vi "myRIO_BRig_RT_v0,85__PortC.vi"() -> ()   [LabVIEW 2014]
uses:
  myRIO_BRig_RT__Case_Exp_stateList.ctl
  myRIO_BRig_RT__Case_NonExp_stateList.ctl
  <vilib>/Platform/TimedLoop/XDataNode/timing_clust.ctl
  <vilib>/Platform/TimedLoop/XDataNode/nitl_modes.ctl
  <vilib>/Platform/TimedLoop/XDataNode/wakeup.ctl
  <vilib>/WebDAVClient/Advanced/SessionHandle.ctl
  <vilib>/myRIO/Common/Instrument Driver Framework/myRIO v1.0/UART/vis/myRIO v1.0 Close UART.vi
  <vilib>/FPGAPlugInAG/myRIO-1900/niLvFpga_Open_myRIO-1900.vi
  <vilib>/rvi/interface/common/dynamic/niFpgaDynamicAddResources.vi
  <vilib>/Utility/error.llb/Error Cluster From Error Code.vi
  <vilib>/rvi/errors/niLvFpgaAdjustHostInterfaceError.vi
  <vilib>/FPGAPlugInAG/Dynamic/niLvFpga_Close_Dynamic.vi
  <vilib>/myRIO/Common/Instrument Driver Framework/Utilities/vis/FPGA Ref Manager.vi
  <vilib>/myRIO/Common/Instrument Driver Framework/myRIO v1.0/myRIO v1.0 Reset FPGA.vi
  <vilib>/myRIO/Common/Instrument Driver Framework/myRIO v1.0/IRQ/vis/myRIO v1.0 IRQ Info FGV.vi
  <vilib>/myRIO/Common/Instrument Driver Framework/myRIO v1.0/IRQ/vis/myRIO v1.0 Timer IRQ Info FGV.vi
  <vilib>/myRIO/Common/Instrument Driver Framework/myRIO v1.0/IRQ/vis/myRIO v1.0 ISR Agent.vi
  <vilib>/rvi/interface/nirviOpenFPGA/nirviOpenFPGA.xnode
  myRIO_BRig_FPGA_v3,81__PortC__build.lvbitx
  myRIO_BRig_FPGA_v3,81__PortC.vi
  <vilib>/rvi/interface/nirviReadWriteControl/nirviReadWriteControl.xnode
  <vilib>/Platform/TimedLoop/XDataNode/XDataNode.xnode
  <vilib>/rvi/interface/nirviCloseFPGA/nirviCloseFPGA.xnode
  <vilib>/Platform/TimedLoop/XDataNode/XDNodeRunTimeDep.lvlib
  <vilib>/rvi/interface/Simulation/niFpgaSimulationCallBeginRW.vi
  <vilib>/myRIO/Instrument Drivers/Utilities/Utilities.lvlib
  <vilib>/WebDAVClient/NI_WebDAV.lvlib
  NiFpgaLv.dll
panel:
  in  "CueLed_baseline":bool
  out "allReward_R":bool
  out "allReward_L":bool
  in  "I_allReward":bool caption="NonSpecific Lick Direction"
  in  "Tcycle_Reward_max_R":u16=1000 caption="Max" min=5 max=5000 step=5
  in  "Tcycle_Reward_min_R":u16=1000 caption="Min" min=5 max=5000 step=5
  in  "Tcycle_Reward_step_R":u16=1000 caption="Penalty" min=1 max=10000 step=1
  in  "Tcycle_Reward_max_L":u16=1000 caption="Max" min=5 max=5000 step=5
  in  "Tcycle_Reward_min_L":u16=1000 caption="Min" min=5 max=5000 step=5
  in  "Tcycle_Reward_step_L":u16=1000 caption="Penalty" min=1 max=10000 step=1
  in  "MTrig_CueLed":bool
  out "Threshold":bool
  out "tLoop":dbl
  in  "Tcycle_Cue_LED_max":u16=1000 caption="Max" min=5 max=5000 step=5
  in  "Tcycle_Cue_LED_min":u16=1000 caption="Min" min=5 max=5000 step=5
  in  "Tcycle_CuePenalty_LED":u16=1000 caption="Penalty" min=1 max=10000 step=1
  out "power_l2":dbl
  in  "MTrig_Laser_Switch":bool
  in  "Cue1Param_AudioLed_Count_NS":u16
  in  "Cue1Param_AudioLed_Count_Switch":u16
  in  "Cue1Param_AudioLed_Probability_NS":u16
  in  "Cue1Param_CueType_NS":u16(slide) max=2 step=1 scale=0.0..2.0
  in  "Cue1Param_AudioLed_Probability_Switch":u16
  in  "Cue1Param_CueType_Switch":u16(slide) max=2 step=1 scale=0.0..2.0
  in  "CueLed_Freq":dbl=10.0
  in  "CueLed_Tpeak":dbl=2.0
  in  "Laser_power_step_l2":dbl
  in  "Laser_power_max_l2":dbl
  in  "Laser_power_min_l2":dbl
  in  "Laser_Tshutter_l2":dbl=2.0
  in  "Laser_Freq_l2":dbl=10.0
  in  "Laser_Tpeak_l2":dbl=2.0
  in  "Laser_duration_l2":u16
  in  "LC_Sel_Count_NS_l2":u16
  in  "LC_Sel_Count_Switch_l2":u16
  in  "LC_Sel_Probability_NS_l2":u16
  in  "LC_Sel_Block_NS_l2":u16(slide) max=2 step=1 scale=0.0..2.0
  in  "LC_Sel_OnOff_NS_l2":bool
  in  "LC_Sel_Probability_Switch_l2":u16
  in  "LC_Sel_Block_Switch_l2":u16(slide) max=2 step=1 scale=0.0..2.0
  in  "LC_Sel_OnOff_Switch_l2":bool
  in  "LC_Sel_Tdelay_NS_l2":u16
  in  "LC_Sel_Tdelay_Switch_l2":u16
  in  "LC_Cue1_Count_NS_l2":u16
  in  "LC_Cue1_Count_Switch_l2":u16
  in  "LC_Cue1_delayOpt_NS_l2":bool
  in  "LC_ENL1_delayOpt_NS_l2":bool
  in  "LC_ENL1_Count_NS_l2":u16
  in  "LC_ENL1_Count_Switch_l2":u16
  in  "LC_Cue1_delayOpt_Switch_l2":bool
  in  "LC_ENL1_delayOpt_Switch_l2":bool
  in  "LC_Cue1_Probability_NS_l2":u16
  in  "LC_Cue1_Block_NS_l2":u16(slide) max=2 step=1 scale=0.0..2.0
  in  "LC_Cue1_OnOff_NS_l2":bool
  in  "LC_Cue1_Probability_Switch_l2":u16
  in  "LC_Cue1_Block_Switch_l2":u16(slide) max=2 step=1 scale=0.0..2.0
  in  "LC_Cue1_OnOff_Switch_l2":bool
  in  "LC_ENL1_Probability_NS_l2":u16 max=100 step=1
  in  "LC_ENL1_Block_NS_l2":u16(slide) max=2 step=1 scale=0.0..2.0
  in  "LC_ENL1_OnOff_NS_l2":bool
  in  "LC_ENL1_Probability_Switch_l2":u16 max=100 step=1
  in  "LC_ENL1_Block_Switch_l2":u16(slide) max=2 step=1 scale=0.0..2.0
  in  "LC_Cue1_Tdelay_NS_l2":u16
  in  "LC_ENL1_Tdelay_NS_l2":u16
  in  "LC_Cue1_Tdelay_Switch_l2":u16
  in  "LC_ENL1_Tdelay_Switch_l2":u16
  in  "LC_ENL1_OnOff_Switch_l2":bool
  in  "LC_Wrong_Probability_l2":u16
  in  "LC_Wrong_Trial_l2":u16(slide) max=2 step=1 scale=0.0..2.0
  in  "LC_Wrong_Block_l2":u16(slide) max=2 step=1 scale=0.0..2.0
  in  "LC_Wrong_OnOff_l2":bool
  in  "LC_Reward_Probability_l2":u16
  in  "LC_Reward_Trial_l2":u16(slide) max=2 step=1 scale=0.0..2.0
  in  "LC_Reward_Block_l2":u16(slide) max=2 step=1 scale=0.0..2.0
  in  "LC_Reward_OnOff_l2":bool
  in  "LC_Wrong_Tdelay_l2":u16
  in  "LC_Reward_Tdelay_l2":u16
  in  "LC_Sel_Count_NS_l1":u16
  in  "LC_Sel_Count_Switch_l1":u16
  in  "LC_Sel_Probability_NS_l1":u16
  in  "LC_Sel_Block_NS_l1":u16(slide) max=2 step=1 scale=0.0..2.0
  in  "LC_Sel_OnOff_NS_l1":bool
  in  "LC_Sel_Probability_Switch_l1":u16
  in  "LC_Sel_Block_Switch_l1":u16(slide) max=2 step=1 scale=0.0..2.0
  in  "LC_Sel_OnOff_Switch_l1":bool
  in  "LC_Sel_Tdelay_NS_l1":u16
  in  "LC_Sel_Tdelay_Switch_l1":u16
  out "I_connect_TCP":bool
  in  "get_countPerMS":bool
  in  "count_warmup_R_reset":bool
  in  "count_warmup_L_reset":bool
  out "count_warmup_R":u16
  out "count_warmup_L":u16
  out "SolenoidReward":bool
  in  "SolenoidProbability_L":u16=100 caption="Reward Time [ms]" min=1 max=1000 step=1
  in  "SolenoidProbability_R":u16=100 caption="Reward Time [ms]" min=1 max=1000 step=1
  out "power_l1":dbl caption="LaserPower"
  in  "Laser_power_step_l1":dbl
  in  "Laser_power_max_l1":dbl
  in  "Recording":bool
  in  "Laser_power_min_l1":dbl
  in  "FPGA_count2ms":dbl=159.0
  in  "Laser_Tshutter_l1":dbl=2.0
  in  "Laser_Freq_l1":dbl=10.0
  in  "Laser_Tpeak_l1":dbl=2.0
  in  "Laser_duration_l1":u16
  out "error out":errorcluster
  in  "LC_Cue1_Count_NS_l1":u16
  in  "LC_Cue1_Count_Switch_l1":u16
  in  "LC_Cue1_delayOpt_NS_l1":bool
  in  "LC_ENL1_delayOpt_NS_l1":bool
  in  "LC_ENL1_Count_NS_l1":u16
  in  "LC_ENL1_Count_Switch_l1":u16
  in  "LC_Cue1_delayOpt_Switch_l1":bool
  in  "LC_ENL1_delayOpt_Switch_l1":bool
  in  "Tcycle_Cue_Audio_max":u16=1000 caption="Max" min=5 max=5000 step=5
  in  "Tcycle_Cue_Audio_min":u16=1000 caption="Min" min=5 max=5000 step=5
  in  "SendData":bool
  out "cSpout":enum16{"Left", "Right"}(ring) caption="Left or Right Spout"
  out "A4":u32 caption="LickCounter_Right"
  out "A2":u32 caption="LickCounter_Left"
  in  "LR_wrong_Event":bool
  out "SelectWrong":bool
  out "SelectReward":bool
  in  "Left(F)_or_Right(T)":bool
  in  "ignoreWrong":bool
  in  "SelectionState":bool
  in  "LR_wrong_Laser":bool
  in  "LR_reward_Laser":bool
  in  "LR_reward_Event":bool
  out "nRewards_Right":u16 caption="# Rewards Total (Right)"
  out "nRewards_Left":u16 caption="# Rewards Total (Left)"
  out "nRewards_cur":u16 caption="# Rewards in Current Block"
  out "TpB_target":u16 caption="Target Trials Per Block"
  out "cState_NonExp":T1 caption="WarmUp State"
  out "iBlock":u16 caption="Current Block"
  out "cState":T2 caption="Experimental State"
  out "iTrial":u16 caption="Current Trial"
  in  "warmupType":u8(slide) max=2 step=1 scale=0.0..2.0
  in  "TestConnection":bool
  in  "warmup":bool caption="WarmUp"
  in  "Data Set Prefix":string="Exp1_TM2"
  out "Connected To Host?":bool
  in  "Host Password":string="sabalab"
  in  "Host UserName":string="Test2"
  in  "sp_RightSpout":u16(slide)=2 max=2 step=1 scale=0.0..2.0
  in  "sp_LeftSpout":u16(slide)=2 max=2 step=1 scale=0.0..2.0
  in  "BUR_max":u16 caption="Count Reward Structure  (0 = off)"
  in  "LC_Wrong_Probability_l1":u16
  in  "LC_Wrong_Trial_l1":u16(slide) max=2 step=1 scale=0.0..2.0
  in  "LC_Wrong_Block_l1":u16(slide) max=2 step=1 scale=0.0..2.0
  in  "LC_Wrong_OnOff_l1":bool
  in  "LC_Reward_Probability_l1":u16
  in  "LC_Reward_Trial_l1":u16(slide) max=2 step=1 scale=0.0..2.0
  in  "LC_Reward_Block_l1":u16(slide) max=2 step=1 scale=0.0..2.0
  in  "LC_Reward_OnOff_l1":bool
  in  "LC_Cue1_Probability_NS_l1":u16
  in  "LC_Cue1_Block_NS_l1":u16(slide) max=2 step=1 scale=0.0..2.0
  in  "LC_Cue1_OnOff_NS_l1":bool
  in  "LC_Cue1_Probability_Switch_l1":u16
  in  "LC_Cue1_Block_Switch_l1":u16(slide) max=2 step=1 scale=0.0..2.0
  in  "LC_Cue1_OnOff_Switch_l1":bool
  in  "LC_ENL1_Probability_NS_l1":u16 max=100 step=1
  in  "LC_ENL1_Block_NS_l1":u16(slide) max=2 step=1 scale=0.0..2.0
  in  "LC_ENL1_OnOff_NS_l1":bool
  in  "LC_ENL1_Probability_Switch_l1":u16 max=100 step=1
  in  "LC_ENL1_Block_Switch_l1":u16(slide) max=2 step=1 scale=0.0..2.0
  in  "Tcycle_Timeout":u16=1000 caption="Timeout Time [ms]" min=10 max=10000 step=1
  in  "Tcycle_Wrong":u16=1000 caption="Wrong Time [ms]" min=10 max=10000 step=1
  in  "Tcycle_Selection":u16=1000 caption="Answer Time [ms]" min=1 max=10000 step=1
  in  "Tcycle_RewardPost":u16=1000 caption="Consumption Time [ms]" min=250 max=10000 step=250
  in  "TpB_Max_R":u16=4 caption="Max TrialsPerBlock" min=1 max=12 step=1
  in  "TpB_Min_R":u16=4 caption="Min TrialsPerBlock" min=1 max=12 step=1
  in  "TpB_Max_L":u16=4 caption="Max TrialsPerBlock" min=1 max=12 step=1
  in  "TpB_Min_L":u16=4 caption="Min TrialsPerBlock" min=1 max=12 step=1
  in  "BUR_min":u16 caption="Count Reward Structure\n(0 = off)"
  in  "TrialUntilReward":bool caption="Ignore Wrong Selection"
  in  "CueCycles":u16=1 caption="Cue Structure" min=1 max=1 step=1
  in  "MTrig_Laser_Tcycle":u16=10 caption="Time [ms]"
  in  "MTrig_Laser_trig":bool
  in  "MTrig_Audio_trig__R":bool caption="Trigger Audio"
  in  "MTrig_Audio_trig__L":bool caption="Trigger Audio"
  in  "RewCalib_Trig_R":bool caption="Calibrate_R"
  in  "RewCalib_Trig_L":bool caption="Calibrate_L"
  in  "MTrig_Solenoid_Tcycle__R":u16=300 caption="Time [ms]"
  in  "MTrig_Solenoid_Tcycle__L":u16=300 caption="Time [ms]"
  in  "MTrig_Solenoid_trig__R":bool caption="Solenoid"
  in  "MTrig_Solenoid_trig__L":bool caption="Solenoid"
  in  "STOP_abort":bool caption="Stop LabView\n(Stops myRio and FPGA)"
  in  "STOP_endBlock":bool caption="Stop Experiment\n@ End of Block"
  in  "STOP_endTrial":bool caption="Stop Experiment\n@ End of Trial"
  in  "START":bool caption="Start Experiment"
  in  "Tcycle_CuePenalty_Audio":u16=1000 caption="Penalty" min=1 max=10000 step=1
  in  "Audio_Amp__R":u16=100 caption="Amp"
  in  "Audio_Freq__R":u8=5 caption="Freq [kHz]" max=14 step=1
  in  "Audio_Amp__L":u16=100 caption="Amp"
  in  "Audio_Freq__L":u8=5 caption="Freq [kHz]" max=14 step=1
  in  "LC_Wrong_Tdelay_l1":u16
  in  "LC_Cue1_Tdelay_NS_l1":u16
  in  "LC_ENL1_Tdelay_NS_l1":u16
  in  "LC_Reward_Tdelay_l1":u16
  in  "LC_Cue1_Tdelay_Switch_l1":u16
  in  "LC_ENL1_Tdelay_Switch_l1":u16
  in  "LC_ENL1_OnOff_Switch_l1":bool
  in  "Tcycle_ENLPenalty":u16=100 caption="Penalty" min=10 max=10000 step=10
  in  "Tcycle_ENL_max":u16=1000 caption="Max" min=250 max=10000 step=250
  in  "Tcycle_ENL_min":u16=1000 caption="Min" min=250 max=10000 step=250
  # "Communication (Host PC)"
  # "Recording Rig"
  # "Experimental Run"
  # "Experiment Task Structure"
  # "STOP experiment at"
  # "Min            Max            Penalty"
  # "(1) = Switching\n(2) = Two Choice"
  # "Enforced\nNonLick"
  # "FPGA Count per [ms]"
  # "Cue Audio"
  # "Current State"
  # "Cue LED"
  # "Global Parameters                                                         Trial Parameters"
  # "Selection"
  # "WarmUp"
  # "Reward - Dispense Water"
  # "Left/Right        Give Reward?        Laser Power [V]"
  # "Laser1      Laser2"
  # "Left"
  # "Cue then reward (no lick)\n \nLeft                    Right"
  # "Right"
  # "Min"
  # "Max"
  # "Dispense Water Probability"
  # "Block                   Trial            Target Trials       # Rewards \n                                                            Per Block             Current"
  # "Left"
  # "WarmUp State"
  # "Trial Per Block Structure \n               Left                        Right"
  # "Lick Counter"
  # "Right"
  # "Left           Right"
  # "Reward - Consumption"
  # "Manual Control"
  # "Min"
  # "# Rewards Total\n                                                                  Left                    Right"
  # "Experimental State"
  # "Penalty - Wrong Choice"
  # "Solenoid\n \nLeft              Right"
  # "Speaker\n \nLeft                    Right"
  # "Laser 1  |  Laser 2"
  # "Max"
  # "Penalty - Choice Timeout"
  # "Time\n[ms]"
  # "Time\n[ms]"
  # "Time = Cue Min"
  # "Cue LED"
  # "Power = Min"
  # "Cue1 Control\n                                  Cue Type           LED Probability [%]      Count"
  # "Laser1 Control\n                               On/Off      Block        Probability [%]   Delay [ms]                              Count"
  # "Laser2 Control\n                               On/Off      Block        Probability [%]   Delay [ms]                              Count"
  # "Audio or LED"
  # "Cue 1"
  # "Enforced\nNonLick\n      1"
  # "Enforced\nNonLick\n      1"
  # "from end"
  # "from end"
  # "Switch\nTrial"
  # "Switch\nTrial"
  # "Switch\nTrial"
  # "from start"
  # "from start"
  # "from end"
  # "from end"
  # "NonSwitch\nTrials"
  # "NonSwitch\nTrials"
  # "NonSwitch\nTrials"
  # "from start"
  # "from start"
  # "Cue 1"
  # "Cue 1"
  # "from end"
  # "from end"
  # "Switch\nTrial"
  # "Switch\nTrial"
  # "Cue Audio Parameters"
  # "Cue LED Parameters"
  # "from start"
  # "from start"
  # "Left                  Right"
  # "Frequency\n[Hz]"
  # "Frequency\n[kHz]"
  # "from end"
  # "from end"
  # "NonSwitch\nTrials"
  # "NonSwitch\nTrials"
  # "Timing [ms]\n                    Peak Width"
  # "from start"
  # "from start"
  # "Amp\n(0 - 32,000)"
  # "Selection"
  # "Selection"
  # "from start"
  # "from start"
  # "Switch\nTrial"
  # "Switch\nTrial"
  # "Speaker\nPattern\nDuring Cue"
  # "from start"
  # "from start"
  # "NonSwitch\nTrials"
  # "NonSwitch\nTrials"
  # "Laser1 Parameters"
  # "Laser2 Parameters"
  # "Laser1 Response\n                               On/Off      Block       Trial       Probability [%]   Delay [ms]"
  # "Laser2 Response\n                               On/Off      Block       Trial       Probability [%]   Delay [ms]"
  # "Frequency\n[Hz]"
  # "Frequency\n[Hz]"
  # "Timing [ms]\n Duration     Peak Width   Shutter"
  # "Timing [ms]\n Duration     Peak Width   Shutter"
  # "Selection Reward"
  # "Selection Reward"
  # "Laser Power [V]\nMin          Max              Step"
  # "Laser Power [V]\nMin          Max              Step"
  # "Selection Wrong"
  # "Selection Wrong"
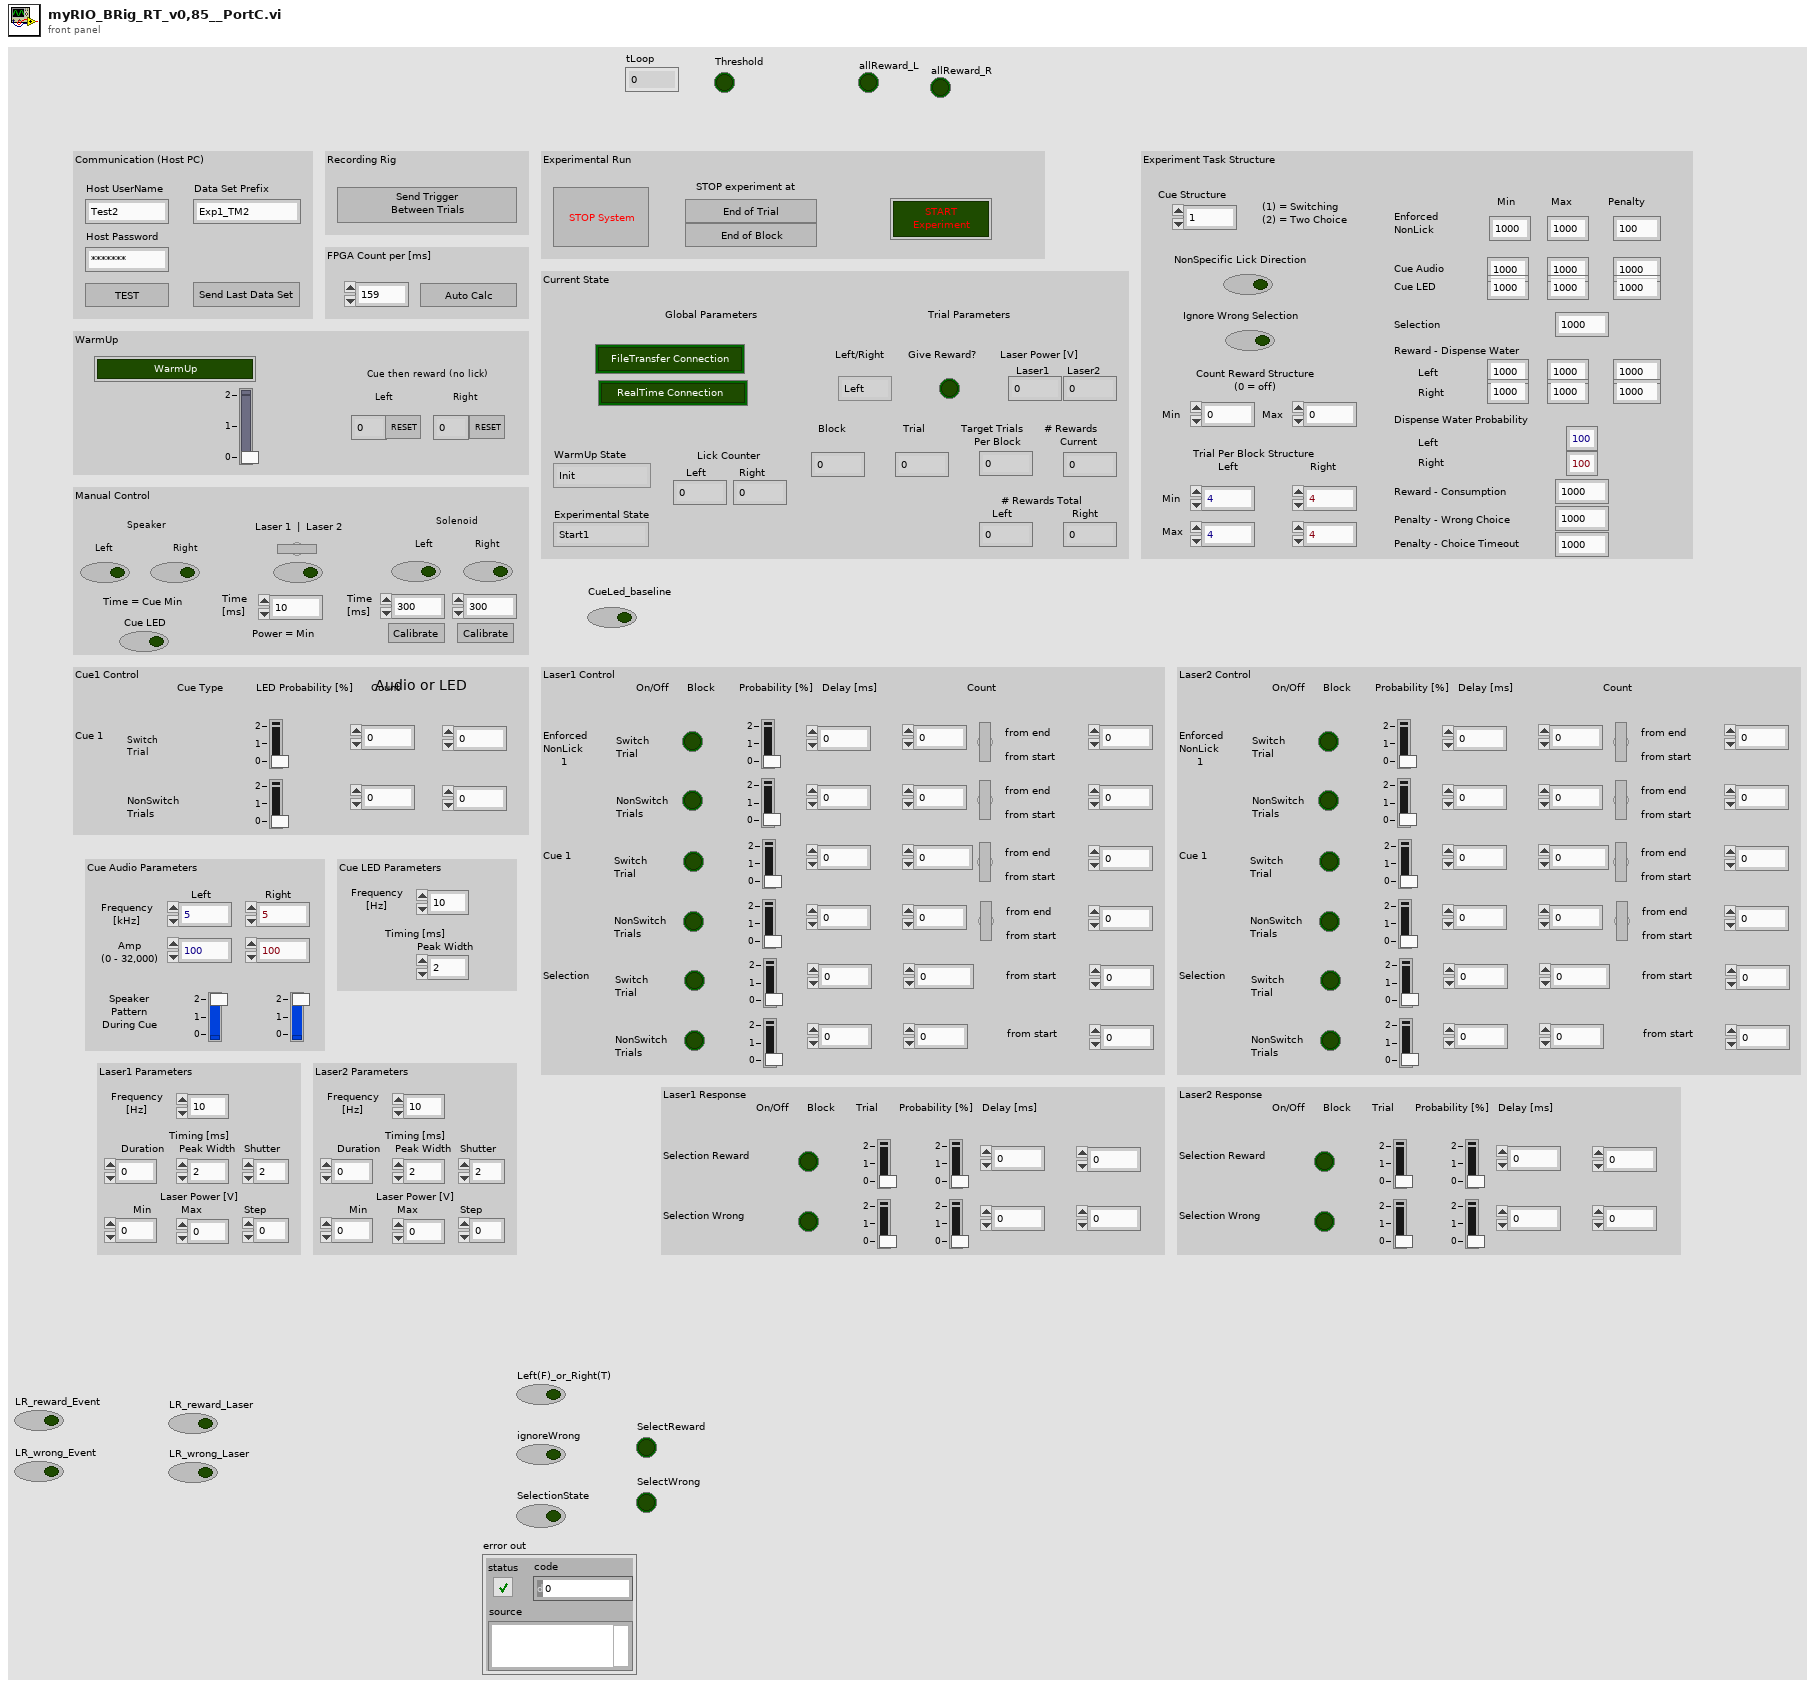
[diagram p1: front panel]
types:
  T1 = typedef "myRIO_BRig_RT__Case_NonExp_stateList.ctl" = enum16{"Init", "UploadSettings_pre", "UploadSettings_Read_dataExp", "UploadSettings_dataExp_1", "UploadSettings_dataExp_2", "UploadSettings_Read_dataLC", "UploadSettings_dataLC_1", "UploadSettings_dataLC_2", "UploadSettings_dataLC_3", "UploadSettings_dataLC_4", "UploadSettings_Read_dataMTrig", "UploadSettings_dataMTrig_1", "UploadSettings_post", "Idle_pre", "IdleEmpty", "IdleEmpty2", "IdleEmpty3", "IdleEmpty4", "Idle", "Idle_2", "Idle_3", "Idle_4", "Idle_5", "Idle_6", "Idle_post", "Cue_pre__pre", "Cue_pre", "Cue", "Cue_LED", "Cue_post", "RewardCalibration_pre", "DispenseWater_pre__pre", "DispenseWater_pre", "DispenseWater", "DispenseWater_post", "TestConnection", "SendData", "Get_FPGA_count_per_ms", "End"}
  T2 = typedef "myRIO_BRig_RT__Case_Exp_stateList.ctl" = enum16{"Start1", "Start2", "Start3", "saveSettings1", "saveSettings2", "saveSettings3", "saveSettings4", "saveSettings_LC_ENL_l1", "saveSettings_LC_ENL_l2", "saveSettings_LC_Cue_l1", "saveSettings_LC_Cue_l2", "saveSettings6_LC_l1_Other", "SaveSettings6_LC_l2_Other", "setSettings_Audio", "setSettings_Laser", "initBlock_pre", "initBlock", "initBlock2", "initBlock_post", "initTrial_pre", "initTrial", "initTrial2", "initTrial3", "initTrial4", "initTrial_LC_ENL1", "initTrial_LC_Cue1", "initTrial_LC_Cue1_2", "initTrial_LC_Sel", "initTrial_post", "ENL1_pre", "ENL1", "ENL1_post", "ENL1Penalty_pre", "ENL1Penalty", "ENL2_pre", "ENL2", "ENL2Penalty_pre", "ENL2Penalty", "Cue1_pre", "Cue1", "Cue1_post", "Cue1Penalty_pre", "Cue1Penalty", "Cue2_pre", "Cue2", "Cue2Penalty_pre", "Cue2Penalty", "Selection_pre", "Selection", "Select_post", "SelectReward_pre", "SelectReward", "SelectRewardPost_pre", "SelectRewardPost", "SelectWrong_pre", "SelectWrong", "SelectWrong_post", "SelectTimeout_pre", "SelectTimeout", "SelectTimeout_post", "endTrial_pre", "endTrial1", "endTrial2", "endTrial3", "endTrial_post", "endBlock_pre", "endBlock", "endBlock_post", "endExp", "commConnect", "commUpload_pre", "commUpload_dataBlock", "commUpload_dataCurrent", "commUpload_dataExp", "commUpload_dataLC", "commUpload_dataTrial", "commUpload_post", "saveData_pre", "saveData_dataBlock", "saveData_dataCurrent", "saveData_dataExp", "saveData_dataLC", "saveData_dataTrial", "saveData_post", "empty_endBlock1", "empty_endBlock2", "empty_endTrial1", "empty_endTrial2", "empty_endTrial3", "empty_endTrial4", "empty_endTrial5", "dummyState", "dummyState_endBlock"}
  T3 = typedef "XDNodeRunTimeDep.lvlib/timing_clust.ctl" = cluster{"Expected End [f-1]":u64, "Actual End [f-1]":u64, "Finished Late? [f-1]":bool, "Expected End [i-1]":u64, "Actual End [i-1]":u64, "Finished Late? [i-1]":bool, "Expected Start [i]":u64, "Actual Start [i]":u64, "Expected Start [f]":u64, "Actual Start [f]":u64, "Source Name":string, "Structure Name":string, "Period":i64, "Deadline":i64, "Offset":i64, "Start":i64, "Priority":i32, "Timeout":i32, "Mode":T4, "Wakeup Reason":T5, "Error":errorcluster, "Source Type":string, "Secondary Source Type":string, "Global End Time":u64, "Global Start Time":u64, "Frame Duration":u64, "Iteration Duration":u64, "Assigned CPU":i32, "I/O Scan Engine Mode":u32}
  T4 = typedef "XDNodeRunTimeDep.lvlib/nitl_modes.ctl" = enum32{"No Change", "Process missed periods, maintain original phase", "Discard missed periods, maintain original phase", "Process missed periods, ignore original phase", "Discard missed periods, ignore original phase"}
  T5 = typedef "XDNodeRunTimeDep.lvlib/wakeup.ctl" = enum32{"Normal", "Aborted", "Asynchronous wakeup", "Timing source error", "Timed loop error", "Timeout"}
  T6 = typedef "NI_WebDAV.lvlib/SessionHandle.ctl" = refnum<k1>
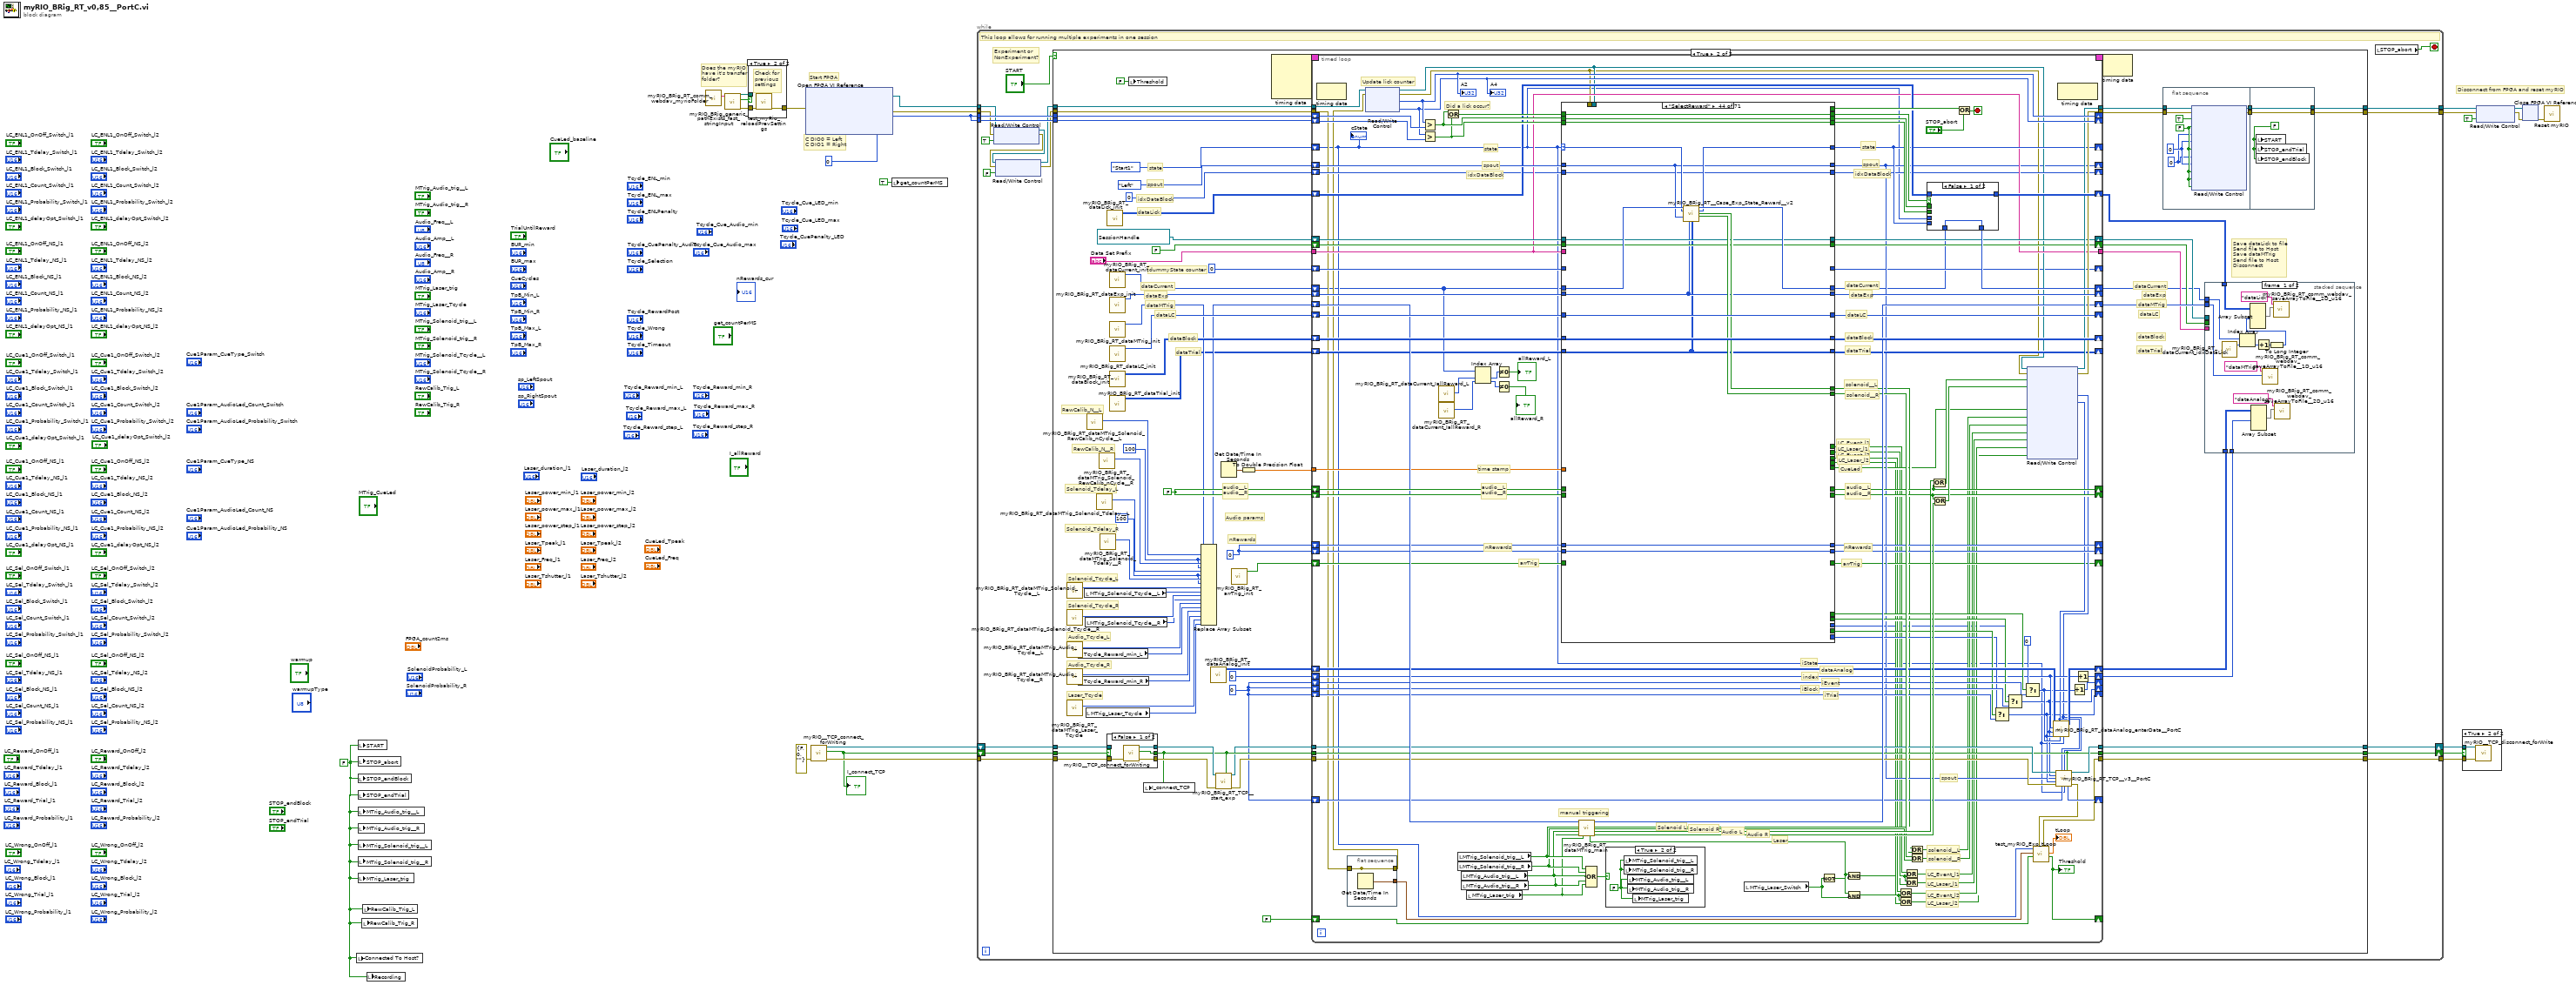
[diagram p0: block diagram]
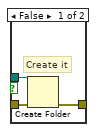
[diagram p3: hidden frame]
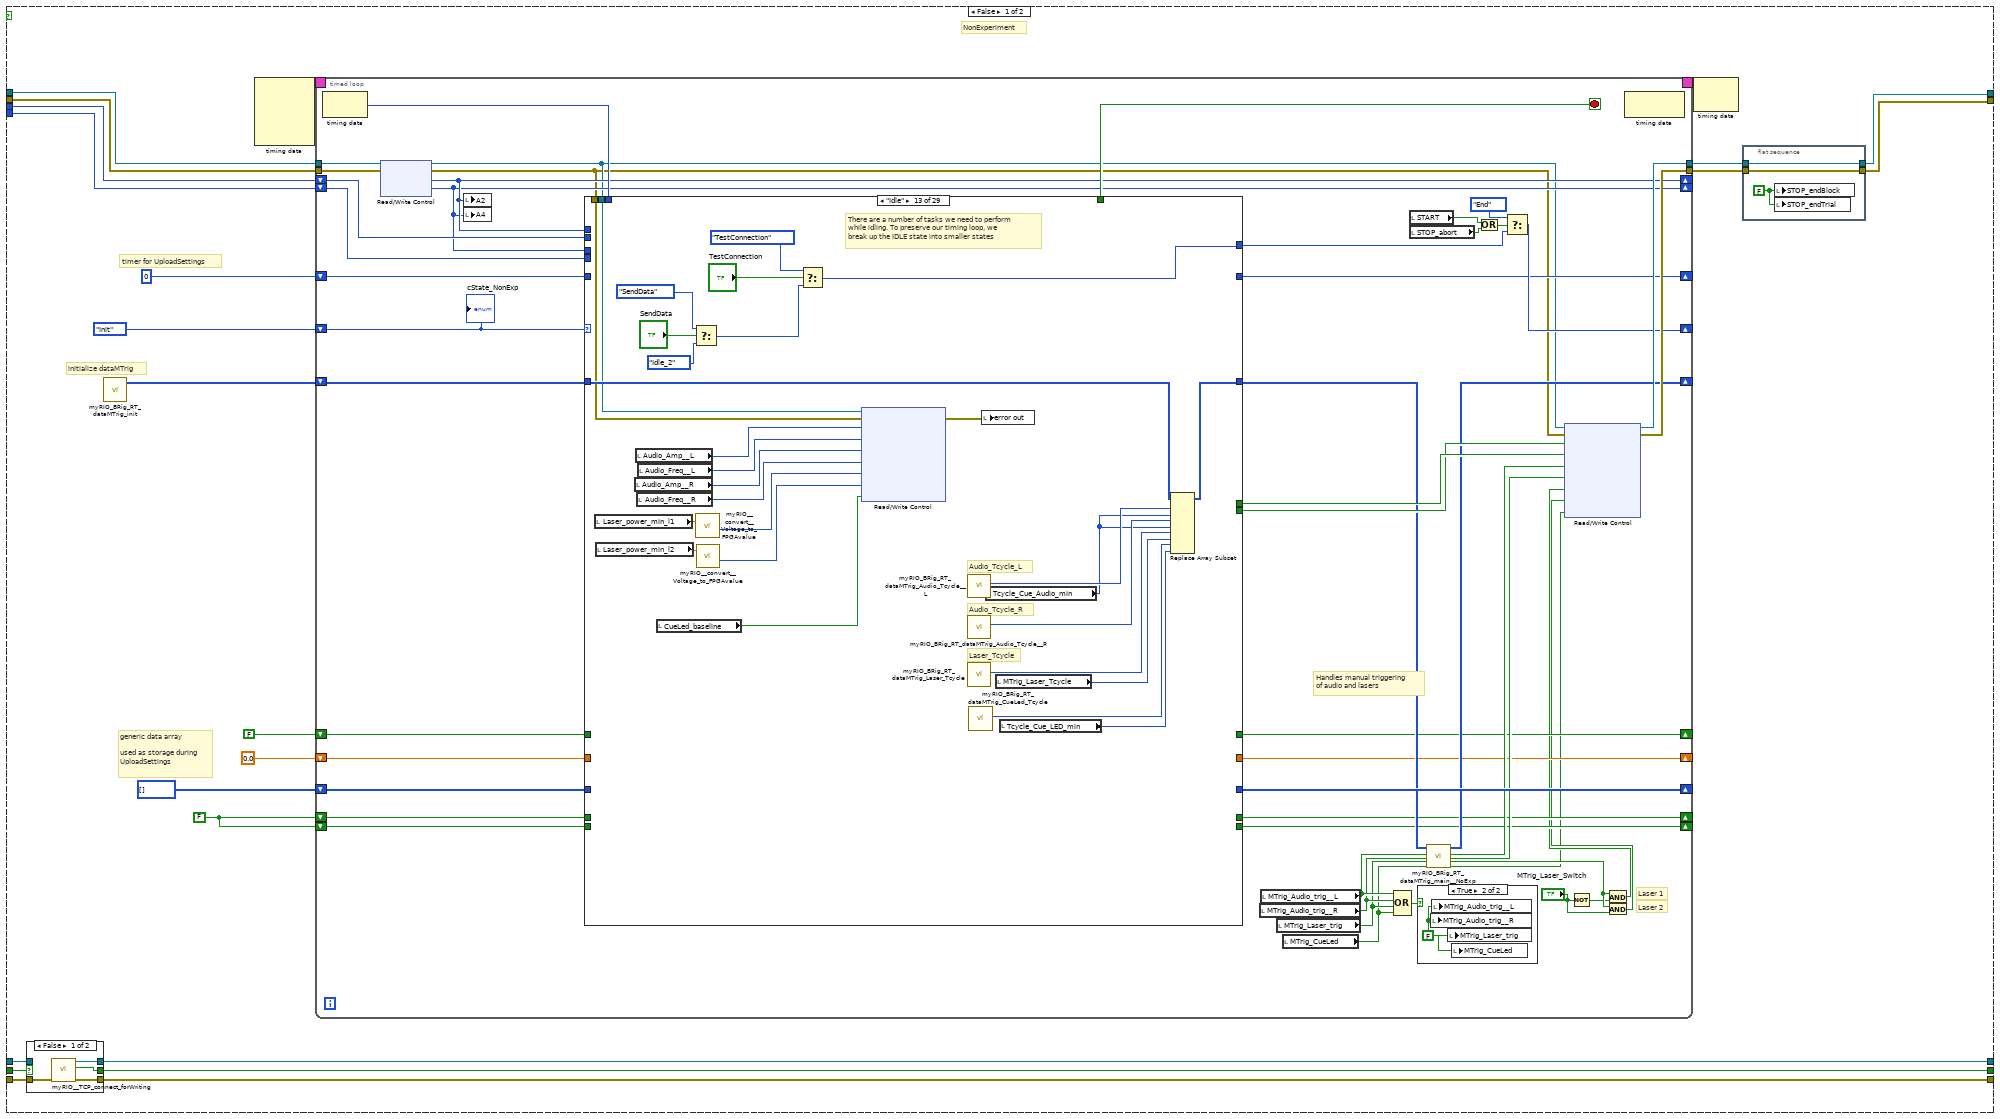
[diagram p4: hidden frame]
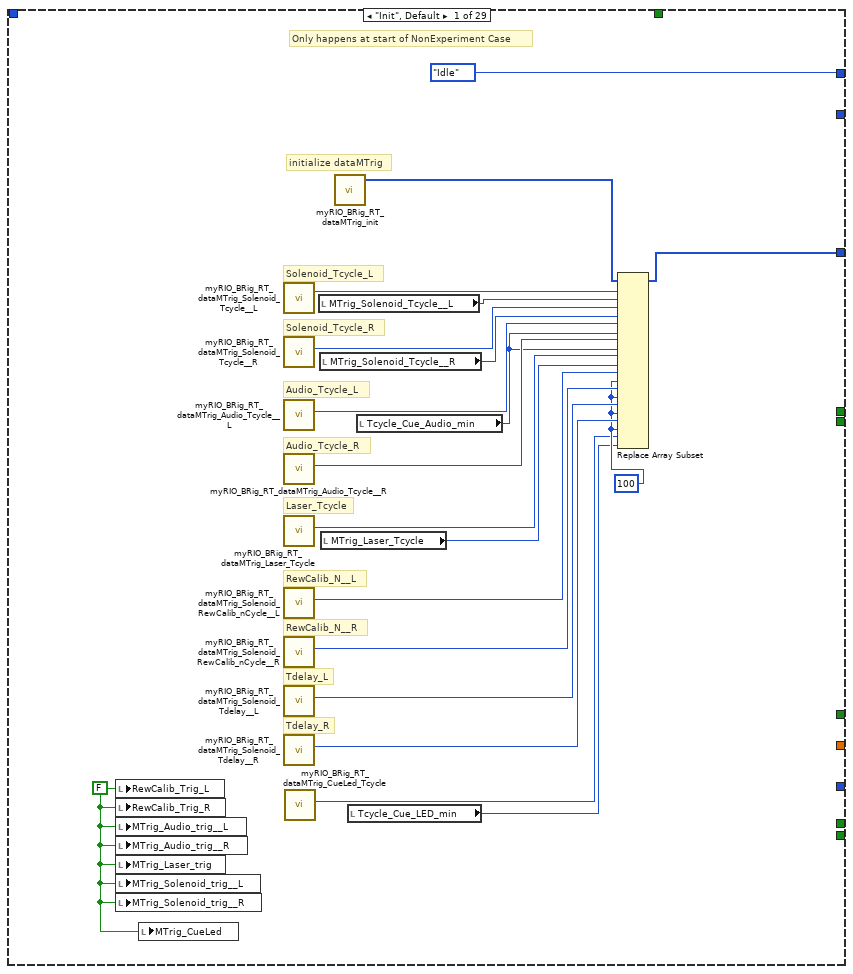
[diagram p7: hidden frame]
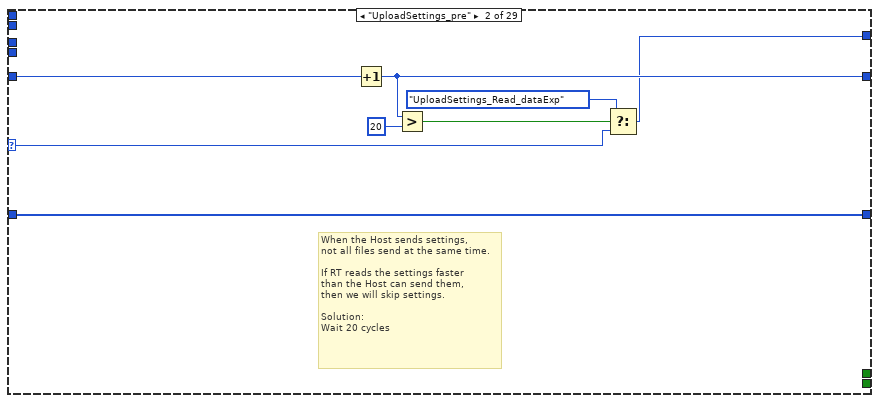
[diagram p8: hidden frame]
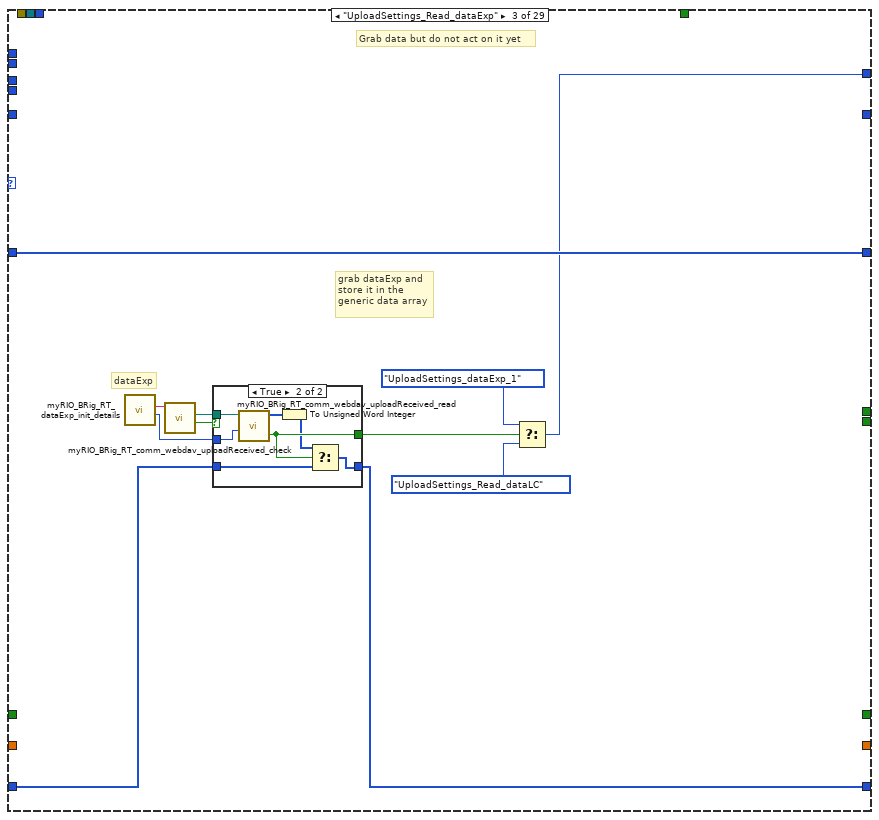
[diagram p9: hidden frame]
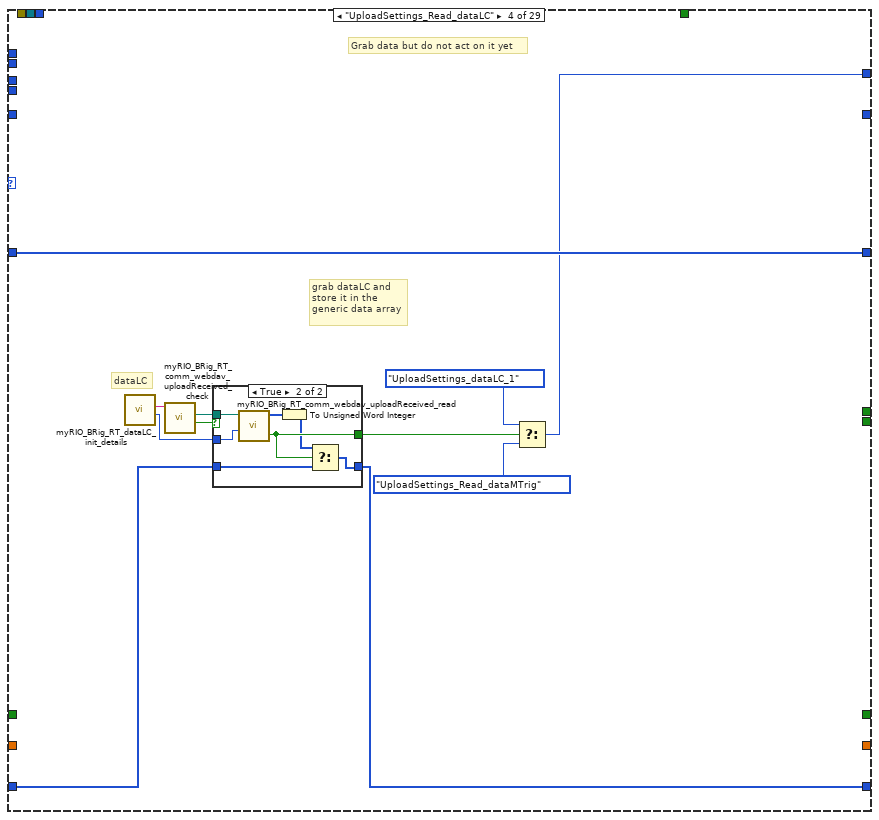
[diagram p11: hidden frame]
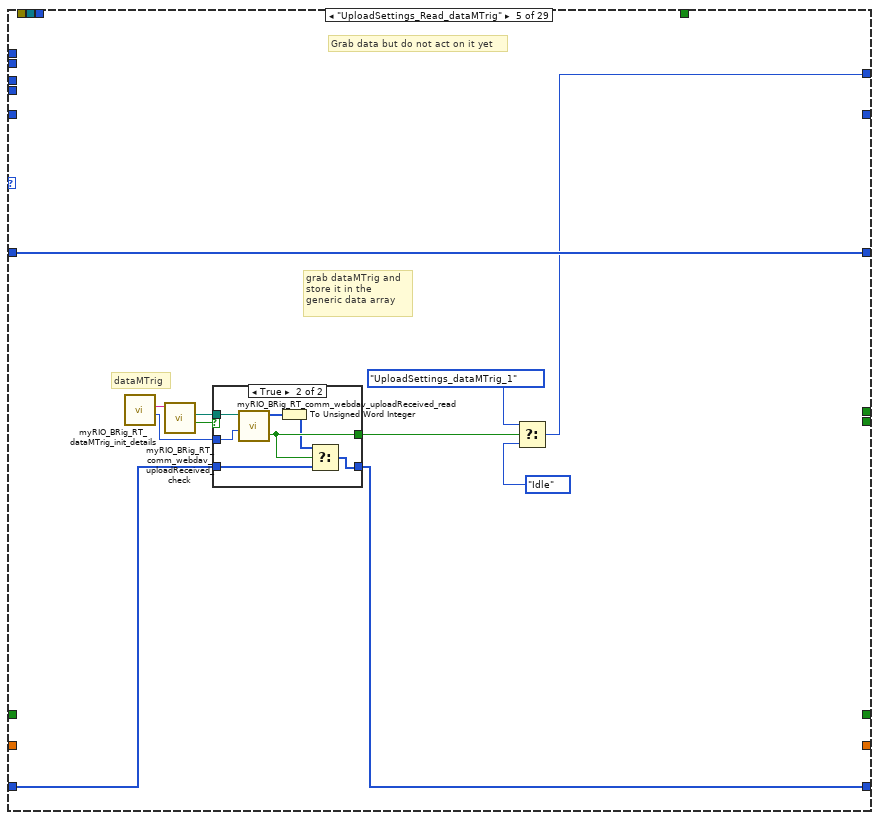
[diagram p13: hidden frame]
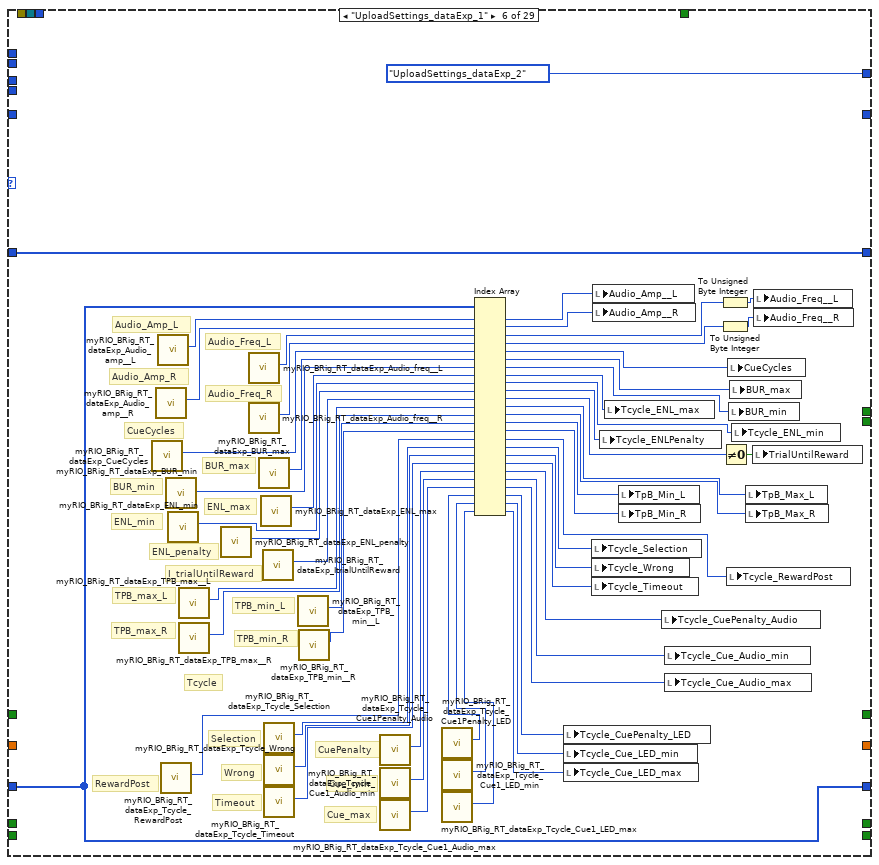
[diagram p15: hidden frame]
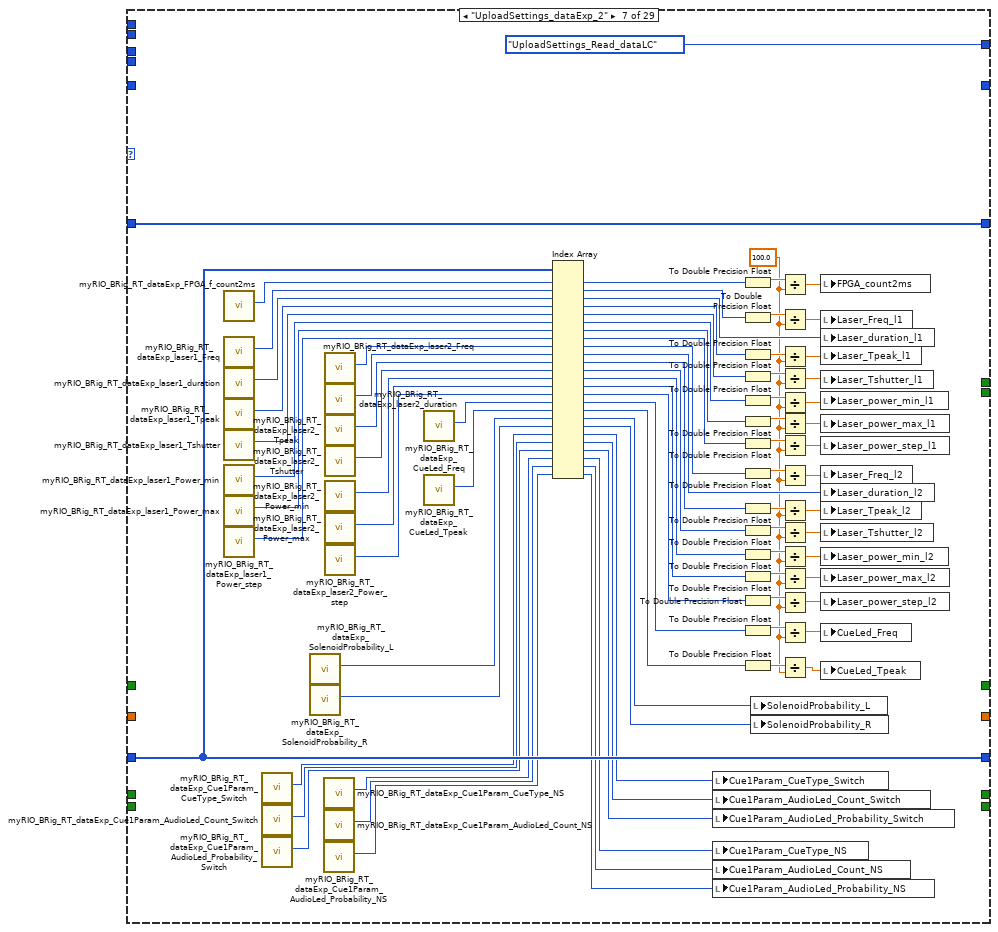
[diagram p16: hidden frame]
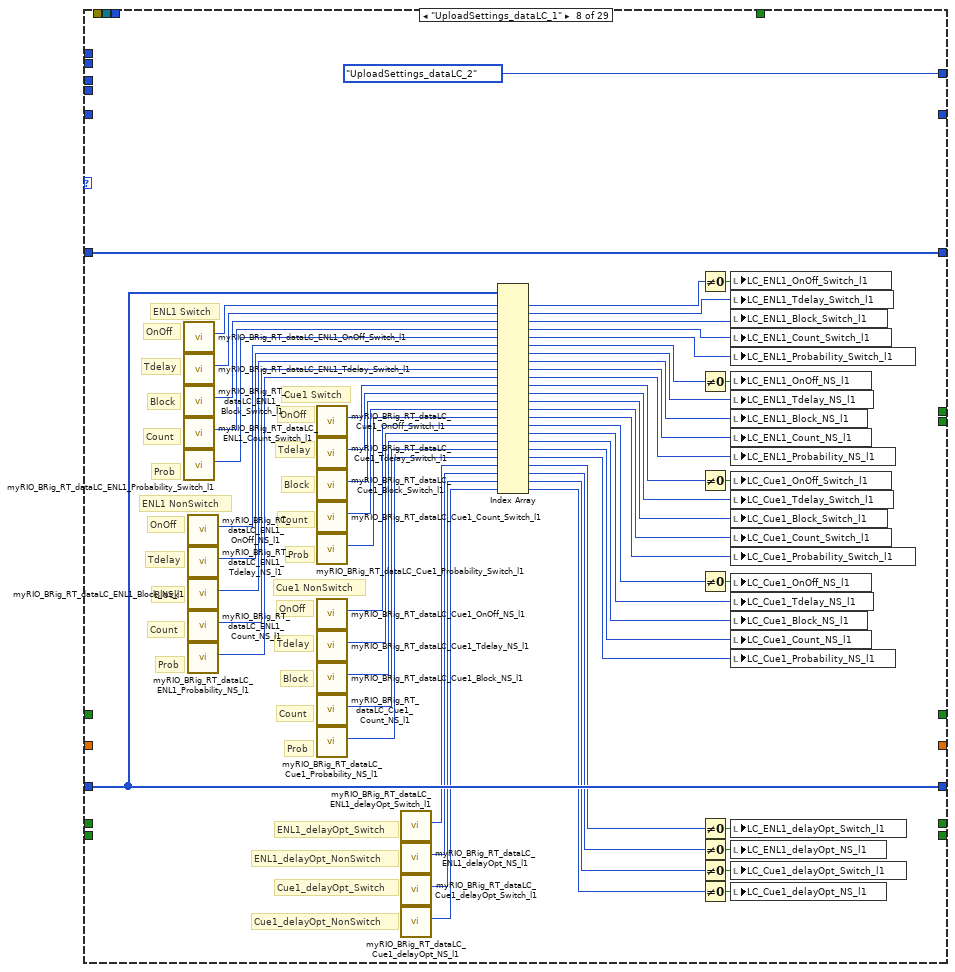
[diagram p17: hidden frame]
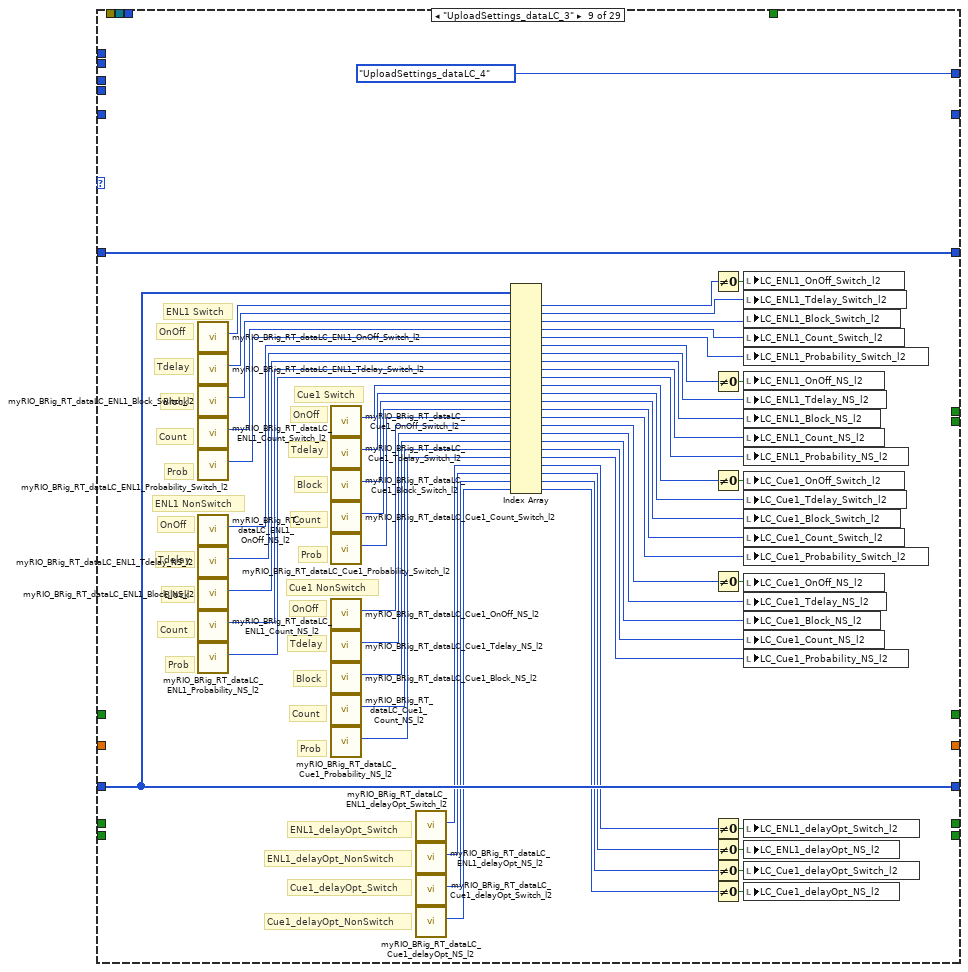
[diagram p18: hidden frame]
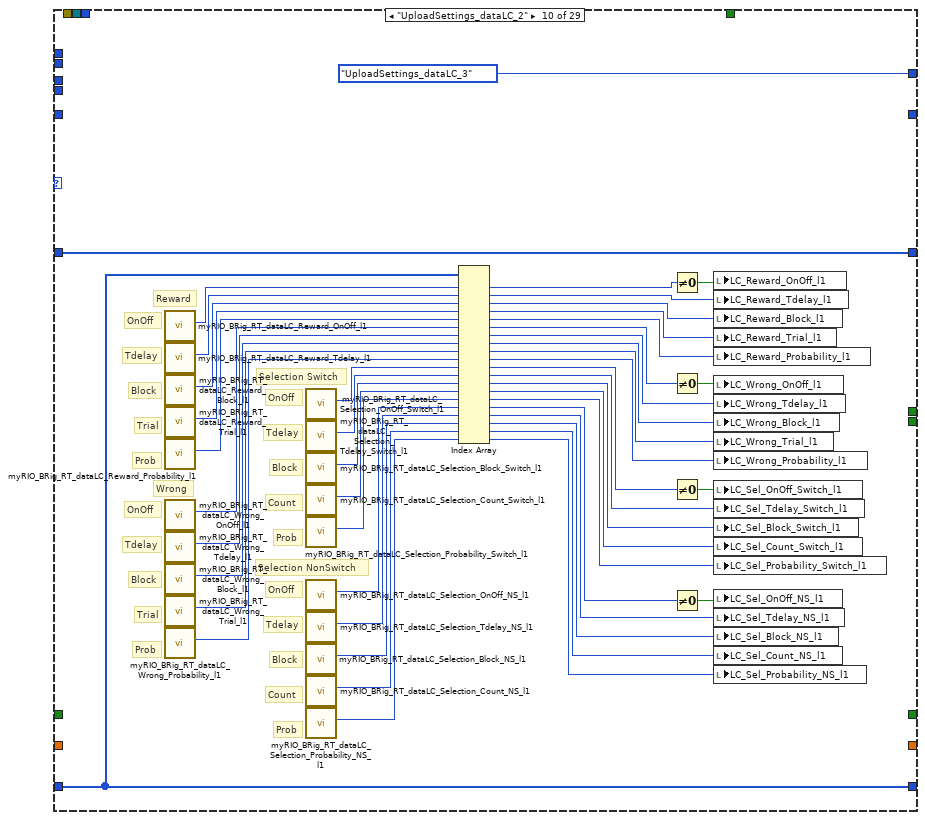
[diagram p19: hidden frame]
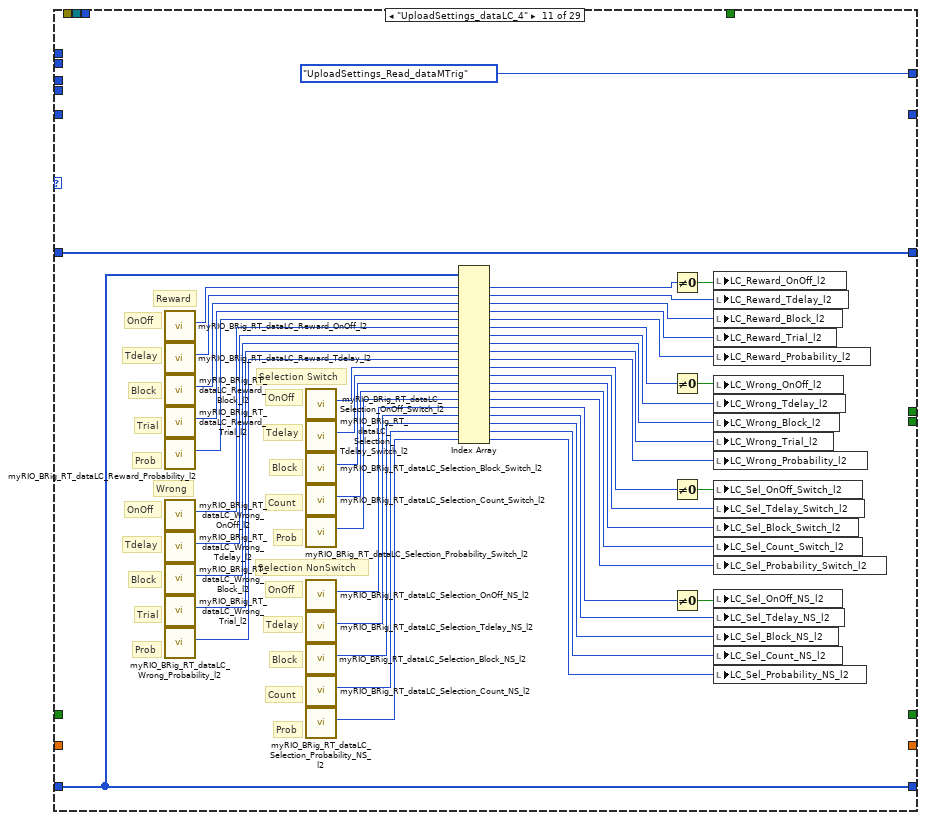
[diagram p20: hidden frame]
diagram:
  w17 = u32 0
  w1 = FALSE
  # "Does the myRIO\nhave it's transfer\nfolder?"
  # "C DIO0 = Left\nC DIO1 = Right"
  # "Start FPGA"
  # "Disconnect from FPGA and reset myRIO"
  n1 = local write "Connected To Host?"(w1) -> ()
  n2 = local write "START"(w1) -> ()
  n3 = local write "STOP_abort"(w1) -> ()
  n4 = local write "STOP_endBlock"(w1) -> ()
  n5 = local write "STOP_endTrial"(w1) -> ()
  n6 = local write "MTrig_Audio_trig__L"(w1) -> ()
  n7 = local write "MTrig_Audio_trig__R"(w1) -> ()
  n8 = local write "MTrig_Solenoid_trig__L"(w1) -> ()
  n9 = local write "MTrig_Solenoid_trig__R"(w1) -> ()
  n10 = local write "MTrig_Laser_trig"(w1) -> ()
  n11 = local write "RewCalib_Trig_R"(w1) -> ()
  n12 = local write "RewCalib_Trig_L"(w1) -> ()
  n13 = local write "Recording"(w1) -> ()
  n14 = call "myRIO_BRig_RT_comm_webdav_myrioFolder.vi"() -> ("output_myrioFolder"=w14:string)  [unwired: 11 in]
  n15 = call "myRIO_BRig_generic_pathExists_fast_stringInput.vi"("input_filePath"=w14) -> ("output_error"=w13:errorcluster, "output_Iexist"=w12:bool, "output_filePath"=w11:path)  [unwired: 8 in]
  n16 = case shown="True" w12 {
    tunnel: w11 -> [w26 _]
    tunnel: w13 -> [w25 w28]
    tunnel: [w24 w27] -> w9
    frame False {
      # "Create it"
      n17 = Create Folder(path (use dialog)=w26, error in=w25) -> (error out=w24:errorcluster)  [unwired: 1 in, 2 out]
    }
    frame True {
      # "Check for\nprevious\nsettings"
      n18 = call "test_myRio_reloadPrevSettings.vi"("input_error"=w28) -> ("output_error"=w27:errorcluster)  [unwired: 10 in]
    }
  }
  n19 = xnode "Open FPGA VI Reference"("error in"=w9) -> ("FPGA VI Reference Out"=w19:refnum<k20>, "error out"=w18:errorcluster)  [unwired: 1 in]
  n20 = call "myRIO__TCP_connect_forWriting.vi"("input_error"=errorcluster {"status"=FALSE, "code"=0, "source"=""}) -> ("output_error"=w7:errorcluster, "output_connected"=w6:bool, "output_hTCP"=w10:refnum<k5>)  [unwired: 8 in]
  "I_connect_TCP" <- w6
  n21 = local write "get_countPerMS"(TRUE ("get_countPerMS")) -> ()
  n22 = while {
    tunnel: w19 -> [w38]
    tunnel: w18 -> [w43]
    tunnel: w17 -> [w46]
    tunnel: w17 -> [w45]
    tunnel: [w36] -> w16
    tunnel: [w35] -> w15
    shift-right: [w32] -> w5
    shift-left: w6 -> [w33]
    tunnel: w7 -> [w31]
    shift-right: [w30] -> w4
    shift-left: w10 -> [w34]
    tunnel: [w29] -> w3
    stop <- w44 stop-if-true
    # "Experiment or\nNonExperiment?"
    # "This loop allows for running multiple experiments in one session"
    n23 = xnode "Read/Write Control"("FPGA VI Reference In"=w38, "error in"=w43, "Counts_Reset"=TRUE) -> ("FPGA VI Reference Out"=w40:refnum<k20>, "error out"=w41:errorcluster)
    n24 = xnode "Read/Write Control"("FPGA VI Reference In"=w40, "error in"=w41, "Counts_Reset"=FALSE) -> ("FPGA VI Reference Out"=w37:refnum<k20>, "error out"=w39:errorcluster)
    n25 = case shown="True" "START" {
      tunnel: w46 -> [w67 w1512]
      tunnel: w45 -> [w66 w1511]
      tunnel: w39 -> [w64 w1446]
      tunnel: w37 -> [w65 w1447]
      tunnel: [w62 w1508] -> w36
      tunnel: [w60 w1503] -> w35
      tunnel: w34 -> [w53 w1457]
      tunnel: [w51 w1461] -> w30
      tunnel: w33 -> [w52 w1459]
      tunnel: [w50 w1460] -> w32
      tunnel: w31 -> [w54 w1458]
      tunnel: [w49 w1456] -> w29
      frame False {
        w57 = FALSE
        # "generic data array\n\nused as storage during\nUploadSettings"
        # "timer for UploadSettings"
        # "initialize dataMTrig"
        # "NonExperiment"
        n26 = case shown="False" w52 {
          selector: w52 -> [_ w76]
          tunnel: w54 -> [w73 w78]
          tunnel: [w74 w78] -> w49
          tunnel: w53 -> [_ w77]
          tunnel: [w75 w77] -> w51
          tunnel: [w72 w76] -> w50
          frame False {
            n27 = call "myRIO__TCP_connect_forWriting.vi"("input_error"=w73) -> ("output_error"=w74:errorcluster, "output_connected"=w72:bool, "output_hTCP"=w75:refnum<k5>)  [unwired: 8 in]
          }
          frame True {
          }
        }
        n28 = call "myRIO_BRig_RT_dataMTrig_init.vi"() -> ("output_dataMTrig"=w68:u16[])  [unwired: 5 in]
        n29 = node-c288() -> (w71:T3)  [unwired: 4 in]
        n30 = timed-loop {
          timing: w71 -> [_]
          timing-out: [_] -> w70
          shift-right: [w117] -> _
          shift-left: w68 -> [w129]
          shift-right: [w111] -> _
          shift-left: myRIO_BRig_RT__Case_NonExp_stateList."Init" ("Enum") -> [w123]
          shift-right: [w105] -> _
          shift-left: w67 -> [w106]
          shift-right: [w103] -> _
          shift-left: w66 -> [w104]
          tunnel: [w125] -> w63
          tunnel: [w124] -> w61
          tunnel: w64 -> [w127]
          tunnel: w65 -> [w126]
          shift-right: [w122] -> _
          shift-left: u16[] [] ("output_data") -> [w121]
          shift-right: [w107] -> _
          shift-left: u16 0 ("Audio_Amp__L") -> [w108]
          shift-right: [w100] -> _
          shift-left: w57 -> [w102]
          shift-right: [w99] -> _
          shift-left: w57 -> [w101]
          shift-right: [w95] -> _
          shift-left: FALSE -> [w96]
          shift-right: [w93] -> _
          shift-left: 0.0 -> [w94]
          stop <- w130 stop-if-true
          # "Laser 2"
          # "Laser 1"
          # "Handles manual triggering\nof audio and lasers"
          n31 = node-c288() -> (w128:i64)  [unwired: 1 in]
          n32 = xnode "Read/Write Control"("FPGA VI Reference In"=w126, "error in"=w127) -> ("FPGA VI Reference Out"=w98:refnum<k20>, "error out"=w97:errorcluster, "A2_LickL"=w105:u32, "A4_LickR"=w103:u32)
          n33 = local write "A2"(w105) -> ()
          n34 = local write "A4"(w103) -> ()
          n35 = case shown="\"Idle\"" w123 {
            selector: w123 -> [_ w155 _ _ _ _ _ _ _ _ _ _ _ _ _ _ _ _ _ w1060 w1119 _ _ w1324 _ _ _ w1397 w1438]
            tunnel: [myRIO_BRig_RT__Case_NonExp_stateList."Idle" ("Enum") w153 w160 w179 w198 myRIO_BRig_RT__Case_NonExp_stateList."UploadSettings_dataExp_2" ("Enum") myRIO_BRig_RT__Case_NonExp_stateList."UploadSettings_Read_dataLC" ("Enum") myRIO_BRig_RT__Case_NonExp_stateList."UploadSettings_dataLC_2" ("Enum") myRIO_BRig_RT__Case_NonExp_stateList."UploadSettings_dataLC_4" ("Enum") myRIO_BRig_RT__Case_NonExp_stateList."UploadSettings_dataLC_3" ("f") myRIO_BRig_RT__Case_NonExp_stateList."UploadSettings_Read_dataMTrig" ("f") myRIO_BRig_RT__Case_NonExp_stateList."Idle" ("Enum") w607 w643 myRIO_BRig_RT__Case_NonExp_stateList."Idle_5" ("Enum") w716 w834 w996 w1027 w1055 w1114 myRIO_BRig_RT__Case_NonExp_stateList."DispenseWater_pre" ("Enum") w1270 w1322 w1344 myRIO_BRig_RT__Case_NonExp_stateList."Idle" ("Enum") myRIO_BRig_RT__Case_NonExp_stateList."Idle" ("Enum") w1396 w1438] -> w112
            tunnel: [w143 w152 w170 w189 w208 w272 w356 w409 w468 w521 w568 w584 w611 w658 w702 w721 w839 w994 w1034 w1061 w1120 w1181 w1307 w1329 w1355 w1389 w1394 w1406 w1436] -> w118
            tunnel: [_ _ _ _ _ _ _ _ _ _ _ _ _ _ _ _ _ _ _ _ _ _ _ _ _ _ _ _ TRUE] -> w130
            tunnel: w129 -> [_ w152 w170 w189 w208 w272 w356 w409 w468 w521 w568 w585 w610 w658 w702 w722 w840 w994 w1035 w1062 w1121 w1167 w1303 w1330 w1356 w1389 w1394 w1406 w1436]
            tunnel: w128 -> [_ _ _ _ _ _ _ _ _ _ _ _ _ _ _ _ _ _ _ _ _ _ _ w1334 _ _ _ _ _]
            tunnel: [_ _ w161 w180 w199 w237 w354 w410 w469 w517 w564 w569 _ _ _ _ _ _ w1023 _ w1108 _ _ _ _ _ _ _ _] -> w122
            tunnel: w121 -> [_ _ w162 w181 w200 w237 w354 w410 w469 w517 w564 w569 _ _ _ _ _ _ _ _ w1109 _ _ _ _ _ _ _ _]
            tunnel: [_ _ _ _ _ _ _ _ _ _ _ _ _ _ _ _ _ _ _ _ _ _ _ w1331 _ _ _ _ _] -> w120
            tunnel: [_ _ _ _ _ _ _ _ _ _ _ _ _ _ _ _ _ _ _ _ _ _ _ w1313 _ _ _ _ _] -> w119
            tunnel: w108 -> [_ w159 _ _ _ _ _ _ _ _ _ _ _ _ _ _ _ _ _ _ _ _ _ _ _ _ _ _ _]
            tunnel: [_ w158 _ _ _ _ _ _ _ _ _ _ _ _ _ _ _ _ _ _ _ _ _ _ _ _ _ _ _] -> w107
            tunnel: w106 -> [_ _ _ _ _ _ _ _ _ _ _ _ _ _ _ _ _ _ _ w1066 w1125 _ _ _ _ _ _ _ _]
            tunnel: w105 -> [_ _ _ _ _ _ _ _ _ _ _ _ _ _ _ _ _ _ _ w1067 w1126 _ _ _ _ _ _ _ _]
            tunnel: w104 -> [_ _ _ _ _ _ _ _ _ _ _ _ _ _ _ _ _ _ _ w1064 w1123 _ _ _ _ _ _ _ _]
            tunnel: w103 -> [_ _ _ _ _ _ _ _ _ _ _ _ _ _ _ _ _ _ _ w1065 w1124 _ _ _ _ _ _ _ _]
            tunnel: w102 -> [_ _ _ _ _ _ _ _ _ _ _ _ _ _ _ _ _ _ _ w1052 w1111 _ _ _ _ _ _ _ _]
            tunnel: w101 -> [_ _ _ _ _ _ _ _ _ _ _ _ _ _ _ _ _ _ _ w1051 w1110 _ _ _ _ _ _ _ _]
            tunnel: [_ _ _ _ _ _ _ _ _ _ _ _ _ _ _ _ _ _ w1025 w1052 w1111 _ _ _ _ _ _ _ _] -> w100
            tunnel: [_ _ _ _ _ _ _ _ _ _ _ _ _ _ _ _ _ _ w1024 w1051 w1110 _ _ _ _ _ _ _ _] -> w99
            tunnel: w98 -> [_ _ _ _ _ _ _ _ _ _ _ _ w600 w616 w704 _ _ _ _ _ w1107 _ _ _ _ _ _ w1401 _]
            tunnel: w97 -> [_ _ _ _ _ _ _ _ _ _ _ _ w599 w617 w703 _ _ _ _ _ w1106 _ _ _ _ _ _ w1400 _]
            tunnel: w96 -> [_ _ _ _ _ _ _ _ _ _ _ _ _ _ _ _ _ _ _ _ _ _ _ _ _ _ _ w1405 _]
            tunnel: [_ _ _ _ _ _ _ _ _ _ _ _ _ _ _ _ _ _ _ _ _ _ _ _ _ _ _ TRUE _] -> w95
            tunnel: w94 -> [_ _ _ _ _ _ _ _ _ _ _ _ _ _ _ _ _ _ _ _ _ _ _ _ _ _ _ w1403 _]
            tunnel: [_ _ _ _ _ _ _ _ _ _ _ _ _ _ _ _ _ _ _ _ _ _ _ _ _ _ _ w1402 _] -> w93
            frame "Init", Default {
              w134 = FALSE ("RewCalib_Trig_L")
              w135 = u16 100 ("new element/subarray")
              # "Only happens at start of NonExperiment Case"
              # "Tdelay_R"
              # "Tdelay_L"
              # "RewCalib_N__R"
              # "RewCalib_N__L"
              # "Solenoid_Tcycle_R"
              # "Solenoid_Tcycle_L"
              # "Laser_Tcycle"
              # "Audio_Tcycle_R"
              # "Audio_Tcycle_L"
              # "initialize dataMTrig"
              n36 = local write "RewCalib_Trig_L"(w134) -> ()
              n37 = local write "RewCalib_Trig_R"(w134) -> ()
              n38 = local write "MTrig_Audio_trig__L"(w134) -> ()
              n39 = local write "MTrig_Audio_trig__R"(w134) -> ()
              n40 = local write "MTrig_Laser_trig"(w134) -> ()
              n41 = local write "MTrig_Solenoid_trig__L"(w134) -> ()
              n42 = local write "MTrig_Solenoid_trig__R"(w134) -> ()
              n43 = local write "MTrig_CueLed"(w134) -> ()
              n44 = call "myRIO_BRig_RT_dataMTrig_Solenoid_Tcycle__L.vi"() -> ("output_Solenoid_Tcycle__L"=w145:i32)  [unwired: 11 in]
              n45 = call "myRIO_BRig_RT_dataMTrig_Solenoid_Tcycle__R.vi"() -> ("output_Solenoid_Tcycle__R"=w146:i32)  [unwired: 11 in]
              n46 = call "myRIO_BRig_RT_dataMTrig_Audio_Tcycle__L.vi"() -> ("output_Audio_Tcycle__L"=w147:i32)  [unwired: 11 in]
              n47 = call "myRIO_BRig_RT_dataMTrig_Audio_Tcycle__R.vi"() -> ("output_Audio_Tcycle__R"=w148:i32)  [unwired: 11 in]
              n48 = call "myRIO_BRig_RT_dataMTrig_Laser_Tcycle.vi"() -> ("output_Laser_Tcycle"=w149:i32)  [unwired: 11 in]
              n49 = call "myRIO_BRig_RT_dataMTrig_Solenoid_RewCalib_nCycle__L.vi"() -> ("output_Solenoid_RewCalib_nCycle__L"=w141:i32)  [unwired: 11 in]
              n50 = call "myRIO_BRig_RT_dataMTrig_Solenoid_RewCalib_nCycle__R.vi"() -> ("output_Solenoid_RewCalib_nCycle__R"=w140:i32)  [unwired: 11 in]
              n51 = call "myRIO_BRig_RT_dataMTrig_Solenoid_Tdelay__L.vi"() -> ("output_Solenoid_Tdelay__L"=w139:i32)  [unwired: 11 in]
              n52 = call "myRIO_BRig_RT_dataMTrig_Solenoid_Tdelay__R.vi"() -> ("output_Solenoid_Tdelay__R"=w138:i32)  [unwired: 11 in]
              n53 = call "myRIO_BRig_RT_dataMTrig_CueLed_Tcycle.vi"() -> ("output_CueLed_Tcycle"=w133:i32)  [unwired: 11 in]
              n54 = local read "MTrig_Solenoid_Tcycle__L"() -> (w150:u16)
              n55 = local read "MTrig_Solenoid_Tcycle__R"() -> (w151:u16)
              n56 = local read "MTrig_Laser_Tcycle"() -> (w136:u16)
              n57 = call "myRIO_BRig_RT_dataMTrig_init.vi"() -> ("output_dataMTrig"=w144:u16[])  [unwired: 5 in]
              n58 = local read "Tcycle_Cue_LED_min"() -> (w132:u16)
              n59 = local read "Tcycle_Cue_Audio_min"() -> (w137:u16)
              n60 = Replace Array Subset(array=w144, new element #1=w150, index #1=w145, new element #2=w151, index #2=w146, new element #3=w137, index #3=w147, new element #4=w137, index #4=w148, new element #5=w136, index #5=w149, new element #6=w135, index #6=w141, new element #7=w135, index #7=w140, new element #8=w135, index #8=w139, new element #9=w135, index #9=w138, new element #10=w132, index #10=w133) -> (w143:u16[])
            }
            frame "UploadSettings_pre" {
              # "When the Host sends settings,\nnot all files send at the same time.\n\nIf RT reads the settings faster\nthan the Host can send them,\nthen we will skip settings.\n\nSolution:\nWait 20 cycles"
              n61 = Increment(x=w159) -> (x+1=w158:u16)
              n62 = Greater?(x=w158, y=u16 20) -> (0:w156:bool)
              n63 = Select(t=myRIO_BRig_RT__Case_NonExp_stateList."UploadSettings_Read_dataExp", s=w156, f=w155) -> (s? t:f=w153:T1)
            }
            frame "UploadSettings_Read_dataExp" {
              # "Grab data but do not act on it yet"
              # "grab dataExp and\nstore it in the\ngeneric data array"
              # "dataExp"
              n64 = call "myRIO_BRig_RT_dataExp_init_details.vi"() -> ("output_dataSize"=w166:i32, "output_dataName"=w169:string)  [unwired: 10 in]
              n65 = call "myRIO_BRig_RT_comm_webdav_uploadReceived_check.vi"("input_dataName"=w169) -> ("output_Iexist"=w168:bool, "output_dataPath"=w167:path)  [unwired: 9 in]
              n66 = case shown="True" w168 {
                tunnel: w167 -> [_ w178]
                tunnel: w166 -> [_ w177]
                tunnel: [_ w176] -> w165
                tunnel: w162 -> [w171 w175]
                tunnel: [w171 w172] -> w161
                frame False {
                }
                frame True {
                  n67 = call "myRIO_BRig_RT_comm_webdav_uploadReceived_read.vi"("input_dataSize"=w177, "input_filePath"=w178) -> ("output_Ivalid"=w176:bool, "output_data"=w174:i64[])  [unwired: 8 in]
                  n68 = To Unsigned Word Integer(number=w174) -> (unsigned 16bit integer=w173:u16[])
                  n69 = Select(t=w173, s=w176, f=w175) -> (s? t:f=w172:u16[])
                }
              }
              n70 = Select(t=myRIO_BRig_RT__Case_NonExp_stateList."UploadSettings_dataExp_1", s=w165, f=myRIO_BRig_RT__Case_NonExp_stateList."UploadSettings_Read_dataLC" ("t")) -> (s? t:f=w160:T1)
            }
            frame "UploadSettings_Read_dataLC" {
              # "Grab data but do not act on it yet"
              # "grab dataLC and\nstore it in the\ngeneric data array"
              # "dataLC"
              n71 = call "myRIO_BRig_RT_dataLC_init_details.vi"() -> ("output_dataSize"=w185:i32, "output_dataName"=w188:string)  [unwired: 10 in]
              n72 = call "myRIO_BRig_RT_comm_webdav_uploadReceived_check.vi"("input_dataName"=w188) -> ("output_Iexist"=w187:bool, "output_dataPath"=w186:path)  [unwired: 9 in]
              n73 = case shown="True" w187 {
                tunnel: w186 -> [_ w197]
                tunnel: w185 -> [_ w196]
                tunnel: [_ w195] -> w184
                tunnel: w181 -> [w190 w194]
                tunnel: [w190 w191] -> w180
                frame False {
                }
                frame True {
                  n74 = call "myRIO_BRig_RT_comm_webdav_uploadReceived_read.vi"("input_dataSize"=w196, "input_filePath"=w197) -> ("output_Ivalid"=w195:bool, "output_data"=w193:i64[])  [unwired: 8 in]
                  n75 = To Unsigned Word Integer(number=w193) -> (unsigned 16bit integer=w192:u16[])
                  n76 = Select(t=w192, s=w195, f=w194) -> (s? t:f=w191:u16[])
                }
              }
              n77 = Select(t=myRIO_BRig_RT__Case_NonExp_stateList."UploadSettings_dataLC_1", s=w184, f=myRIO_BRig_RT__Case_NonExp_stateList."UploadSettings_Read_dataMTrig" ("t")) -> (s? t:f=w179:T1)
            }
            frame "UploadSettings_Read_dataMTrig" {
              # "Grab data but do not act on it yet"
              # "grab dataMTrig and\nstore it in the\ngeneric data array"
              # "dataMTrig"
              n78 = call "myRIO_BRig_RT_dataMTrig_init_details.vi"() -> ("output_dataSize"=w204:i32, "output_dataName"=w207:string)  [unwired: 10 in]
              n79 = call "myRIO_BRig_RT_comm_webdav_uploadReceived_check.vi"("input_dataName"=w207) -> ("output_Iexist"=w206:bool, "output_dataPath"=w205:path)  [unwired: 9 in]
              n80 = case shown="True" w206 {
                tunnel: w205 -> [_ w216]
                tunnel: w204 -> [_ w215]
                tunnel: [_ w214] -> w203
                tunnel: w200 -> [w209 w213]
                tunnel: [w209 w210] -> w199
                frame False {
                }
                frame True {
                  n81 = call "myRIO_BRig_RT_comm_webdav_uploadReceived_read.vi"("input_dataSize"=w215, "input_filePath"=w216) -> ("output_Ivalid"=w214:bool, "output_data"=w212:i64[])  [unwired: 8 in]
                  n82 = To Unsigned Word Integer(number=w212) -> (unsigned 16bit integer=w211:u16[])
                  n83 = Select(t=w211, s=w214, f=w213) -> (s? t:f=w210:u16[])
                }
              }
              n84 = Select(t=myRIO_BRig_RT__Case_NonExp_stateList."UploadSettings_dataMTrig_1", s=w203, f=myRIO_BRig_RT__Case_NonExp_stateList."Idle" ("t")) -> (s? t:f=w198:T1)
            }
            frame "UploadSettings_dataExp_1" {
              # "Cue_max"
              # "Cue_min"
              # "CuePenalty"
              # "Timeout"
              # "Wrong"
              # "Selection"
              # "RewardPost"
              # "Tcycle"
              # "TPB_min_R"
              # "TPB_min_L"
              # "TPB_max_R"
              # "TPB_max_L"
              # "I_trialUntilReward"
              # "ENL_penalty"
              # "ENL_min"
              # "ENL_max"
              # "BUR_max"
              # "BUR_min"
              # "CueCycles"
              # "Audio_Freq_R"
              # "Audio_Freq_L"
              # "Audio_Amp_R"
              # "Audio_Amp_L"
              n85 = call "myRIO_BRig_RT_dataExp_CueCycles.vi"() -> ("output_CueCycles"=w264:i32)  [unwired: 11 in]
              n86 = call "myRIO_BRig_RT_dataExp_Audio_amp__R.vi"() -> ("output_Audio_amp__R"=w268:i32)  [unwired: 11 in]
              n87 = call "myRIO_BRig_RT_dataExp_Audio_amp__L.vi"() -> ("output_Audio_amp__L"=w270:i32)  [unwired: 11 in]
              n88 = call "myRIO_BRig_RT_dataExp_Tcycle_RewardPost.vi"() -> ("output_Tcycle_RewardPost"=w236:i32)  [unwired: 11 in]
              n89 = call "myRIO_BRig_RT_dataExp_BUR_min.vi"() -> ("output_BUR_min"=w261:i32)  [unwired: 11 in]
              n90 = call "myRIO_BRig_RT_dataExp_ENL_min.vi"() -> ("output_ENL_min"=w257:i32)  [unwired: 11 in]
              n91 = call "myRIO_BRig_RT_dataExp_TPB_max__L.vi"() -> ("output_TPB_max__L"=w249:i32)  [unwired: 11 in]
              n92 = call "myRIO_BRig_RT_dataExp_TPB_max__R.vi"() -> ("output_TPB_max__R"=w248:i32)  [unwired: 11 in]
              n93 = call "myRIO_BRig_RT_dataExp_ENL_penalty.vi"() -> ("output_ENL_penalty"=w256:i32)  [unwired: 11 in]
              n94 = call "myRIO_BRig_RT_dataExp_Audio_freq__L.vi"() -> ("output_Audio_freq__L"=w266:i32)  [unwired: 11 in]
              n95 = call "myRIO_BRig_RT_dataExp_Audio_freq__R.vi"() -> ("output_Audio_freq__R"=w265:i32)  [unwired: 11 in]
              n96 = call "myRIO_BRig_RT_dataExp_BUR_max.vi"() -> ("output_BUR_max"=w262:i32)  [unwired: 11 in]
              n97 = call "myRIO_BRig_RT_dataExp_ENL_max.vi"() -> ("output_ENL_max"=w258:i32)  [unwired: 11 in]
              n98 = call "myRIO_BRig_RT_dataExp_ItrialUntilReward.vi"() -> ("output_I_trialUntilReward"=w252:i32)  [unwired: 11 in]
              n99 = call "myRIO_BRig_RT_dataExp_Tcycle_Selection.vi"() -> ("output_Tcycle_Selection"=w235:i32)  [unwired: 11 in]
              n100 = call "myRIO_BRig_RT_dataExp_Tcycle_Wrong.vi"() -> ("output_Tcycle_Wrong"=w234:i32)  [unwired: 11 in]
              n101 = call "myRIO_BRig_RT_dataExp_Tcycle_Timeout.vi"() -> ("output_Tcycle_Timeout"=w230:i32)  [unwired: 11 in]
              n102 = call "myRIO_BRig_RT_dataExp_TPB_min__L.vi"() -> ("output_TPB_min__L"=w247:i32)  [unwired: 11 in]
              n103 = call "myRIO_BRig_RT_dataExp_TPB_min__R.vi"() -> ("output_TPB_min__R"=w246:i32)  [unwired: 11 in]
              n104 = call "myRIO_BRig_RT_dataExp_Tcycle_Cue1Penalty_Audio.vi"() -> ("output_Tcycle_Cue1Penalty_Audio"=w228:i32)  [unwired: 11 in]
              n105 = call "myRIO_BRig_RT_dataExp_Tcycle_Cue1_Audio_min.vi"() -> ("output_Tcycle_Cue1_Audio_min"=w226:i32)  [unwired: 11 in]
              n106 = call "myRIO_BRig_RT_dataExp_Tcycle_Cue1_Audio_max.vi"() -> ("output_Tcycle_Cue1_Audio_max"=w224:i32)  [unwired: 11 in]
              n107 = call "myRIO_BRig_RT_dataExp_Tcycle_Cue1Penalty_LED.vi"() -> ("output_Tcycle_Cue1Penalty_LED"=w222:i32)  [unwired: 11 in]
              n108 = call "myRIO_BRig_RT_dataExp_Tcycle_Cue1_LED_min.vi"() -> ("output_Tcycle_Cue1_LED_min"=w221:i32)  [unwired: 11 in]
              n109 = call "myRIO_BRig_RT_dataExp_Tcycle_Cue1_LED_max.vi"() -> ("output_Tcycle_Cue1_LED_max"=w220:i32)  [unwired: 11 in]
              n110 = Index Array(array=w237, index #1=w270, index #2=w268, index #3=w266, index #4=w265, index #5=w264, index #6=w262, index #7=w261, index #8=w258, index #9=w257, index #10=w256, index #11=w252, index #12=w249, index #13=w248, index #14=w247, index #15=w246, index #16=w236, index #17=w235, index #18=w234, index #19=w230, index #20=w228, index #21=w226, index #22=w224, index #23=w222, index #24=w221, index #25=w220) -> (element #1=w269:u16, element #2=w267:u16, element #3=w240:u16, element #4=w239:u16, element #5=w263:u16, element #6=w260:u16, element #7=w259:u16, element #8=w255:u16, element #9=w254:u16, element #10=w253:u16, element #11=w250:u16, element #12=w245:u16, element #13=w244:u16, element #14=w243:u16, element #15=w242:u16, element #16=w233:u16, element #17=w232:u16, element #18=w231:u16, element #19=w229:u16, element #20=w227:u16, element #21=w225:u16, element #22=w223:u16, element #23=w219:u16, element #24=w218:u16, element #25=w217:u16)
              n111 = local write "Tcycle_CuePenalty_LED"(w219) -> ()
              n112 = local write "Tcycle_Cue_LED_min"(w218) -> ()
              n113 = local write "Tcycle_Cue_LED_max"(w217) -> ()
              n114 = local write "Tcycle_Selection"(w232) -> ()
              n115 = local write "Tcycle_Wrong"(w231) -> ()
              n116 = local write "Tcycle_Timeout"(w229) -> ()
              n117 = local write "Audio_Amp__L"(w269) -> ()
              n118 = local write "Audio_Amp__R"(w267) -> ()
              n119 = local write "Tcycle_ENLPenalty"(w253) -> ()
              n120 = local write "Tcycle_ENL_max"(w255) -> ()
              n121 = local write "TpB_Min_L"(w243) -> ()
              n122 = local write "TpB_Min_R"(w242) -> ()
              n123 = local write "Tcycle_CuePenalty_Audio"(w227) -> ()
              n124 = local write "Tcycle_Cue_Audio_min"(w225) -> ()
              n125 = local write "Tcycle_Cue_Audio_max"(w223) -> ()
              n126 = To Unsigned Byte Integer(number=w240) -> (unsigned 8bit integer=w241:u8)
              n127 = To Unsigned Byte Integer(number=w239) -> (unsigned 8bit integer=w238:u8)
              n128 = Not Equal To 0?(x=w250) -> (x != 0?=w251:bool)
              n129 = local write "Tcycle_RewardPost"(w233) -> ()
              n130 = local write "CueCycles"(w263) -> ()
              n131 = local write "BUR_min"(w259) -> ()
              n132 = local write "BUR_max"(w260) -> ()
              n133 = local write "Tcycle_ENL_min"(w254) -> ()
              n134 = local write "TpB_Max_L"(w245) -> ()
              n135 = local write "TpB_Max_R"(w244) -> ()
              n136 = local write "TrialUntilReward"(w251) -> ()
              n137 = local write "Audio_Freq__L"(w241) -> ()
              n138 = local write "Audio_Freq__R"(w238) -> ()
            }
            frame "UploadSettings_dataExp_2" {
              w292 = 100.0 ("y")
              n139 = call "myRIO_BRig_RT_dataExp_FPGA_f_count2ms.vi"() -> ("output_FPGA_f_count2ms"=w353:i32)  [unwired: 11 in]
              n140 = call "myRIO_BRig_RT_dataExp_laser1_Freq.vi"() -> ("output_laser1_Freq"=w341:i32)  [unwired: 11 in]
              n141 = call "myRIO_BRig_RT_dataExp_laser1_duration.vi"() -> ("output_laser1_duration"=w340:i32)  [unwired: 11 in]
              n142 = call "myRIO_BRig_RT_dataExp_laser1_Tpeak.vi"() -> ("output_laser1_Tpeak"=w339:i32)  [unwired: 11 in]
              n143 = call "myRIO_BRig_RT_dataExp_laser1_Tshutter.vi"() -> ("output_laser1_Tshutter"=w338:i32)  [unwired: 11 in]
              n144 = call "myRIO_BRig_RT_dataExp_laser1_Power_min.vi"() -> ("output_laser1_Power_min"=w337:i32)  [unwired: 11 in]
              n145 = call "myRIO_BRig_RT_dataExp_laser1_Power_max.vi"() -> ("output_laser1_Power_max"=w336:i32)  [unwired: 11 in]
              n146 = call "myRIO_BRig_RT_dataExp_laser1_Power_step.vi"() -> ("output_laser1_Power_step"=w335:i32)  [unwired: 11 in]
              n147 = call "myRIO_BRig_RT_dataExp_Cue1Param_CueType_Switch.vi"() -> ("output_Cue1Param_CueType_Switch"=w286:i32)  [unwired: 11 in]
              n148 = call "myRIO_BRig_RT_dataExp_Cue1Param_AudioLed_Count_Switch.vi"() -> ("output_Cue1Param_AudioLed_Count_Switch"=w285:i32)  [unwired: 11 in]
              n149 = call "myRIO_BRig_RT_dataExp_Cue1Param_AudioLed_Probability_Switch.vi"() -> ("output_Cue1Param_AudioLed_Probability_Switch"=w284:i32)  [unwired: 11 in]
              n150 = call "myRIO_BRig_RT_dataExp_SolenoidProbability_L.vi"() -> ("output_SolenoidProbability_L"=w288:i32)  [unwired: 11 in]
              n151 = call "myRIO_BRig_RT_dataExp_SolenoidProbability_R.vi"() -> ("output_SolenoidProbability_R"=w287:i32)  [unwired: 11 in]
              n152 = call "myRIO_BRig_RT_dataExp_Cue1Param_CueType_NS.vi"() -> ("output_Cue1Param_CueType_NS"=w283:i32)  [unwired: 11 in]
              n153 = call "myRIO_BRig_RT_dataExp_Cue1Param_AudioLed_Count_NS.vi"() -> ("output_Cue1Param_AudioLed_Count_NS"=w282:i32)  [unwired: 11 in]
              n154 = call "myRIO_BRig_RT_dataExp_Cue1Param_AudioLed_Probability_NS.vi"() -> ("output_Cue1Param_AudioLed_Probability_NS"=w281:i32)  [unwired: 11 in]
              n155 = call "myRIO_BRig_RT_dataExp_laser2_Freq.vi"() -> ("output_laser2_Freq"=w334:i32)  [unwired: 11 in]
              n156 = call "myRIO_BRig_RT_dataExp_laser2_duration.vi"() -> ("output_laser2_duration"=w333:i32)  [unwired: 11 in]
              n157 = call "myRIO_BRig_RT_dataExp_laser2_Tpeak.vi"() -> ("output_laser2_Tpeak"=w332:i32)  [unwired: 11 in]
              n158 = call "myRIO_BRig_RT_dataExp_laser2_Tshutter.vi"() -> ("output_laser2_Tshutter"=w331:i32)  [unwired: 11 in]
              n159 = call "myRIO_BRig_RT_dataExp_laser2_Power_min.vi"() -> ("output_laser2_Power_min"=w330:i32)  [unwired: 11 in]
              n160 = call "myRIO_BRig_RT_dataExp_laser2_Power_max.vi"() -> ("output_laser2_Power_max"=w329:i32)  [unwired: 11 in]
              n161 = call "myRIO_BRig_RT_dataExp_laser2_Power_step.vi"() -> ("output_laser2_Power_step"=w328:i32)  [unwired: 11 in]
              n162 = call "myRIO_BRig_RT_dataExp_CueLed_Freq.vi"() -> ("output_CueLed_Freq"=w297:i32)  [unwired: 11 in]
              n163 = call "myRIO_BRig_RT_dataExp_CueLed_Tpeak.vi"() -> ("output_CueLed_Tpeak"=w290:i32)  [unwired: 11 in]
              n164 = Index Array(array=w354, index #1=w353, index #2=w341, index #3=w340, index #4=w339, index #5=w338, index #6=w337, index #7=w336, index #8=w335, index #9=w334, index #10=w333, index #11=w332, index #12=w331, index #13=w330, index #14=w329, index #15=w328, index #16=w297, index #17=w290, index #18=w288, index #19=w287, index #20=w286, index #21=w285, index #22=w284, index #23=w283, index #24=w282, index #25=w281) -> (element #1=w352:u16, element #2=w327:u16, element #3=w326:u16, element #4=w325:u16, element #5=w324:u16, element #6=w323:u16, element #7=w313:u16, element #8=w312:u16, element #9=w308:u16, element #10=w307:u16, element #11=w306:u16, element #12=w305:u16, element #13=w304:u16, element #14=w299:u16, element #15=w298:u16, element #16=w291:u16, element #17=w289:u16, element #18=w280:u16, element #19=w279:u16, element #20=w278:u16, element #21=w277:u16, element #22=w276:u16, element #23=w275:u16, element #24=w274:u16, element #25=w273:u16)
              n165 = local write "Cue1Param_CueType_Switch"(w278) -> ()
              n166 = local write "Cue1Param_AudioLed_Count_Switch"(w277) -> ()
              n167 = local write "Cue1Param_AudioLed_Probability_Switch"(w276) -> ()
              n168 = local write "Cue1Param_CueType_NS"(w275) -> ()
              n169 = local write "Cue1Param_AudioLed_Count_NS"(w274) -> ()
              n170 = local write "Cue1Param_AudioLed_Probability_NS"(w273) -> ()
              n171 = To Double Precision Float(number=w352) -> (double precision float=w351:dbl)
              n172 = To Double Precision Float(number=w327) -> (double precision float=w349:dbl)
              n173 = To Double Precision Float(number=w325) -> (double precision float=w346:dbl)
              n174 = To Double Precision Float(number=w324) -> (double precision float=w345:dbl)
              n175 = To Double Precision Float(number=w323) -> (double precision float=w347:dbl)
              n176 = To Double Precision Float(number=w313) -> (double precision float=w318:dbl)
              n177 = To Double Precision Float(number=w312) -> (double precision float=w314:dbl)
              n178 = To Double Precision Float(number=w308) -> (double precision float=w319:dbl)
              n179 = To Double Precision Float(number=w306) -> (double precision float=w321:dbl)
              n180 = To Double Precision Float(number=w305) -> (double precision float=w322:dbl)
              n181 = To Double Precision Float(number=w304) -> (double precision float=w320:dbl)
              n182 = To Double Precision Float(number=w299) -> (double precision float=w302:dbl)
              n183 = To Double Precision Float(number=w298) -> (double precision float=w303:dbl)
              n184 = To Double Precision Float(number=w291) -> (double precision float=w296:dbl)
              n185 = To Double Precision Float(number=w289) -> (double precision float=w295:dbl)
              n186 = local write "SolenoidProbability_L"(w280) -> ()
              n187 = local write "SolenoidProbability_R"(w279) -> ()
              n188 = Divide(x=w351, y=w292) -> (x/y=w350:dbl)
              n189 = Divide(x=w349, y=w292) -> (x/y=w348:dbl)
              n190 = Divide(x=w346, y=w292) -> (x/y=w343:dbl)
              n191 = Divide(x=w345, y=w292) -> (x/y=w342:dbl)
              n192 = Divide(x=w347, y=w292) -> (x/y=w344:dbl)
              n193 = Divide(x=w318, y=w292) -> (x/y=w316:dbl)
              n194 = Divide(x=w314, y=w292) -> (x/y=w315:dbl)
              n195 = Divide(x=w319, y=w292) -> (x/y=w317:dbl)
              n196 = Divide(x=w321, y=w292) -> (x/y=w311:dbl)
              n197 = Divide(x=w322, y=w292) -> (x/y=w310:dbl)
              n198 = Divide(x=w320, y=w292) -> (x/y=w309:dbl)
              n199 = Divide(x=w302, y=w292) -> (x/y=w301:dbl)
              n200 = Divide(x=w303, y=w292) -> (x/y=w300:dbl)
              n201 = Divide(x=w296, y=w292) -> (x/y=w294:dbl)
              n202 = Divide(x=w295, y=w292) -> (x/y=w293:dbl)
              n203 = local write "FPGA_count2ms"(w350) -> ()
              n204 = local write "Laser_Freq_l1"(w348) -> ()
              n205 = local write "Laser_duration_l1"(w326) -> ()
              n206 = local write "Laser_Tpeak_l1"(w343) -> ()
              n207 = local write "Laser_Tshutter_l1"(w342) -> ()
              n208 = local write "Laser_power_min_l1"(w344) -> ()
              n209 = local write "Laser_power_max_l1"(w316) -> ()
              n210 = local write "Laser_power_step_l1"(w315) -> ()
              n211 = local write "Laser_Freq_l2"(w317) -> ()
              n212 = local write "Laser_duration_l2"(w307) -> ()
              n213 = local write "Laser_Tpeak_l2"(w311) -> ()
              n214 = local write "Laser_Tshutter_l2"(w310) -> ()
              n215 = local write "Laser_power_min_l2"(w309) -> ()
              n216 = local write "Laser_power_max_l2"(w301) -> ()
              n217 = local write "Laser_power_step_l2"(w300) -> ()
              n218 = local write "CueLed_Freq"(w294) -> ()
              n219 = local write "CueLed_Tpeak"(w293) -> ()
            }
            frame "UploadSettings_dataLC_1" {
              # "Cue1_delayOpt_NonSwitch"
              # "ENL1_delayOpt_NonSwitch"
              # "Cue1_delayOpt_Switch"
              # "ENL1_delayOpt_Switch"
              # "Count"
              # "Tdelay"
              # "Prob"
              # "OnOff"
              # "Block"
              # "Count"
              # "Tdelay"
              # "Prob"
              # "OnOff"
              # "Block"
              # "Count"
              # "Tdelay"
              # "Prob"
              # "OnOff"
              # "Block"
              # "ENL1 Switch"
              # "Cue1 NonSwitch"
              # "Cue1 Switch"
              # "ENL1 NonSwitch"
              # "Count"
              # "Tdelay"
              # "Prob"
              # "OnOff"
              # "Block"
              n220 = call "myRIO_BRig_RT_dataLC_ENL1_OnOff_Switch_l1.vi"() -> ("output_ENL1_OnOff_Switch_l1"=w408:i32)  [unwired: 11 in]
              n221 = call "myRIO_BRig_RT_dataLC_ENL1_Tdelay_Switch_l1.vi"() -> ("output_ENL1_Tdelay_Switch_l1"=w407:i32)  [unwired: 11 in]
              n222 = call "myRIO_BRig_RT_dataLC_ENL1_Block_Switch_l1.vi"() -> ("output_ENL1_Block_Switch_l1"=w406:i32)  [unwired: 11 in]
              n223 = call "myRIO_BRig_RT_dataLC_ENL1_Count_Switch_l1.vi"() -> ("output_ENL1_Count_Switch_l1"=w405:i32)  [unwired: 11 in]
              n224 = call "myRIO_BRig_RT_dataLC_ENL1_Probability_Switch_l1.vi"() -> ("output_ENL1_Probability_Switch_l1"=w404:i32)  [unwired: 11 in]
              n225 = call "myRIO_BRig_RT_dataLC_ENL1_OnOff_NS_l1.vi"() -> ("output_ENL1_OnOff_NS_l1"=w403:i32)  [unwired: 11 in]
              n226 = call "myRIO_BRig_RT_dataLC_ENL1_Tdelay_NS_l1.vi"() -> ("output_ENL1_Tdelay_NS_l1"=w402:i32)  [unwired: 11 in]
              n227 = call "myRIO_BRig_RT_dataLC_ENL1_Block_NS_l1.vi"() -> ("output_ENL1_All_Block"=w401:i32)  [unwired: 11 in]
              n228 = call "myRIO_BRig_RT_dataLC_ENL1_Count_NS_l1.vi"() -> ("output_ENL1_Count_NS_l1"=w400:i32)  [unwired: 11 in]
              n229 = call "myRIO_BRig_RT_dataLC_ENL1_Probability_NS_l1.vi"() -> ("output_ENL1_Probability_NS_l1"=w399:i32)  [unwired: 11 in]
              n230 = call "myRIO_BRig_RT_dataLC_Cue1_OnOff_Switch_l1.vi"() -> ("output_Cue1_OnOff_Switch_l1"=w398:i32)  [unwired: 11 in]
              n231 = call "myRIO_BRig_RT_dataLC_Cue1_Tdelay_Switch_l1.vi"() -> ("output_Cue1_Tdelay_Switch_l1"=w397:i32)  [unwired: 11 in]
              n232 = call "myRIO_BRig_RT_dataLC_Cue1_Block_Switch_l1.vi"() -> ("output_Cue1_Block_Switch_l1"=w396:i32)  [unwired: 11 in]
              n233 = call "myRIO_BRig_RT_dataLC_Cue1_Count_Switch_l1.vi"() -> ("output_Cue1_Count_Switch_l1"=w395:i32)  [unwired: 11 in]
              n234 = call "myRIO_BRig_RT_dataLC_Cue1_Probability_Switch_l1.vi"() -> ("output_Cue1_Probability_Switch_l1"=w394:i32)  [unwired: 11 in]
              n235 = call "myRIO_BRig_RT_dataLC_Cue1_OnOff_NS_l1.vi"() -> ("output_Cue1_OnOff_NS_l1"=w393:i32)  [unwired: 11 in]
              n236 = call "myRIO_BRig_RT_dataLC_Cue1_Tdelay_NS_l1.vi"() -> ("output_Cue1_Tdelay_NS_l1"=w392:i32)  [unwired: 11 in]
              n237 = call "myRIO_BRig_RT_dataLC_Cue1_Block_NS_l1.vi"() -> ("output_Cue1_Block_NS_l1"=w391:i32)  [unwired: 11 in]
              n238 = call "myRIO_BRig_RT_dataLC_Cue1_Count_NS_l1.vi"() -> ("output_Cue1_Count_NS_l1"=w390:i32)  [unwired: 11 in]
              n239 = call "myRIO_BRig_RT_dataLC_Cue1_Probability_NS_l1.vi"() -> ("output_Cue1_l1_All_Probability"=w389:i32)  [unwired: 11 in]
              n240 = call "myRIO_BRig_RT_dataLC_ENL1_delayOpt_Switch_l1.vi"() -> ("output_ENL1_delayOpt_Switch_l1"=w368:i32)  [unwired: 11 in]
              n241 = call "myRIO_BRig_RT_dataLC_ENL1_delayOpt_NS_l1.vi"() -> ("output_ENL1_delayOpt_NS_l1"=w367:i32)  [unwired: 11 in]
              n242 = call "myRIO_BRig_RT_dataLC_Cue1_delayOpt_Switch_l1.vi"() -> ("output_Cue1_delayOpt_Switch_l1"=w366:i32)  [unwired: 11 in]
              n243 = call "myRIO_BRig_RT_dataLC_Cue1_delayOpt_NS_l1.vi"() -> ("output_Cue1_delayOpt_NS_l1"=w365:i32)  [unwired: 11 in]
              n244 = Index Array(array=w410, index #1=w408, index #2=w407, index #3=w406, index #4=w405, index #5=w404, index #6=w403, index #7=w402, index #8=w401, index #9=w400, index #10=w399, index #11=w398, index #12=w397, index #13=w396, index #14=w395, index #15=w394, index #16=w393, index #17=w392, index #18=w391, index #19=w390, index #20=w389, index #21=w368, index #22=w367, index #23=w366, index #24=w365) -> (element #1=w388:u16, element #2=w387:u16, element #3=w386:u16, element #4=w385:u16, element #5=w384:u16, element #6=w383:u16, element #7=w382:u16, element #8=w381:u16, element #9=w380:u16, element #10=w379:u16, element #11=w378:u16, element #12=w377:u16, element #13=w376:u16, element #14=w375:u16, element #15=w374:u16, element #16=w373:u16, element #17=w372:u16, element #18=w371:u16, element #19=w370:u16, element #20=w369:u16, element #21=w360:u16, element #22=w359:u16, element #23=w358:u16, element #24=w357:u16)
              n245 = Not Equal To 0?(x=w388) -> (x != 0?=w412:bool)
              n246 = Not Equal To 0?(x=w383) -> (x != 0?=w411:bool)
              n247 = Not Equal To 0?(x=w378) -> (x != 0?=w414:bool)
              n248 = Not Equal To 0?(x=w373) -> (x != 0?=w413:bool)
              n249 = Not Equal To 0?(x=w360) -> (x != 0?=w362:bool)
              n250 = Not Equal To 0?(x=w359) -> (x != 0?=w363:bool)
              n251 = Not Equal To 0?(x=w358) -> (x != 0?=w364:bool)
              n252 = Not Equal To 0?(x=w357) -> (x != 0?=w361:bool)
              n253 = local write "LC_ENL1_OnOff_Switch_l1"(w412) -> ()
              n254 = local write "LC_ENL1_Tdelay_Switch_l1"(w387) -> ()
              n255 = local write "LC_ENL1_Block_Switch_l1"(w386) -> ()
              n256 = local write "LC_ENL1_Count_Switch_l1"(w385) -> ()
              n257 = local write "LC_ENL1_Probability_Switch_l1"(w384) -> ()
              n258 = local write "LC_ENL1_OnOff_NS_l1"(w411) -> ()
              n259 = local write "LC_ENL1_Tdelay_NS_l1"(w382) -> ()
              n260 = local write "LC_ENL1_Block_NS_l1"(w381) -> ()
              n261 = local write "LC_ENL1_Count_NS_l1"(w380) -> ()
              n262 = local write "LC_ENL1_Probability_NS_l1"(w379) -> ()
              n263 = local write "LC_Cue1_OnOff_Switch_l1"(w414) -> ()
              n264 = local write "LC_Cue1_Tdelay_Switch_l1"(w377) -> ()
              n265 = local write "LC_Cue1_Block_Switch_l1"(w376) -> ()
              n266 = local write "LC_Cue1_Count_Switch_l1"(w375) -> ()
              n267 = local write "LC_Cue1_Probability_Switch_l1"(w374) -> ()
              n268 = local write "LC_Cue1_OnOff_NS_l1"(w413) -> ()
              n269 = local write "LC_Cue1_Tdelay_NS_l1"(w372) -> ()
              n270 = local write "LC_Cue1_Block_NS_l1"(w371) -> ()
              n271 = local write "LC_Cue1_Count_NS_l1"(w370) -> ()
              n272 = local write "LC_Cue1_Probability_NS_l1"(w369) -> ()
              n273 = local write "LC_ENL1_delayOpt_Switch_l1"(w362) -> ()
              n274 = local write "LC_ENL1_delayOpt_NS_l1"(w363) -> ()
              n275 = local write "LC_Cue1_delayOpt_Switch_l1"(w364) -> ()
              n276 = local write "LC_Cue1_delayOpt_NS_l1"(w361) -> ()
            }
            frame "UploadSettings_dataLC_3" {
              # "Cue1_delayOpt_NonSwitch"
              # "ENL1_delayOpt_NonSwitch"
              # "Cue1_delayOpt_Switch"
              # "ENL1_delayOpt_Switch"
              # "Count"
              # "Tdelay"
              # "Prob"
              # "OnOff"
              # "Block"
              # "Count"
              # "Tdelay"
              # "Prob"
              # "OnOff"
              # "Block"
              # "Count"
              # "Tdelay"
              # "Prob"
              # "OnOff"
              # "Block"
              # "ENL1 Switch"
              # "Cue1 NonSwitch"
              # "Cue1 Switch"
              # "ENL1 NonSwitch"
              # "Count"
              # "Tdelay"
              # "Prob"
              # "OnOff"
              # "Block"
              n277 = call "myRIO_BRig_RT_dataLC_ENL1_OnOff_Switch_l2.vi"() -> ("output_ENL1_OnOff_Switch_l2"=w435:i32)  [unwired: 11 in]
              n278 = call "myRIO_BRig_RT_dataLC_ENL1_Tdelay_Switch_l2.vi"() -> ("output_ENL1_Tdelay_Switch_l2"=w436:i32)  [unwired: 11 in]
              n279 = call "myRIO_BRig_RT_dataLC_ENL1_Block_Switch_l2.vi"() -> ("output_ENL1_Block_Switch_l2"=w437:i32)  [unwired: 11 in]
              n280 = call "myRIO_BRig_RT_dataLC_ENL1_Count_Switch_l2.vi"() -> ("output_ENL1_Count_Switch_l2"=w438:i32)  [unwired: 11 in]
              n281 = call "myRIO_BRig_RT_dataLC_ENL1_Probability_Switch_l2.vi"() -> ("output_ENL1_Probability_Switch_l2"=w439:i32)  [unwired: 11 in]
              n282 = call "myRIO_BRig_RT_dataLC_ENL1_OnOff_NS_l2.vi"() -> ("output_ENL1_OnOff_NS_l2"=w430:i32)  [unwired: 11 in]
              n283 = call "myRIO_BRig_RT_dataLC_ENL1_Tdelay_NS_l2.vi"() -> ("output_ENL1_Tdelay_NS_l2"=w431:i32)  [unwired: 11 in]
              n284 = call "myRIO_BRig_RT_dataLC_ENL1_Block_NS_l2.vi"() -> ("output_ENL1_Block_NS_l2"=w432:i32)  [unwired: 11 in]
              n285 = call "myRIO_BRig_RT_dataLC_ENL1_Count_NS_l2.vi"() -> ("output_ENL1_Count_NS_l2"=w433:i32)  [unwired: 11 in]
              n286 = call "myRIO_BRig_RT_dataLC_ENL1_Probability_NS_l2.vi"() -> ("output_ENL1_Probability_NS_l2"=w434:i32)  [unwired: 11 in]
              n287 = call "myRIO_BRig_RT_dataLC_Cue1_OnOff_Switch_l2.vi"() -> ("output_Cue1_OnOff_Switch_l2"=w425:i32)  [unwired: 11 in]
              n288 = call "myRIO_BRig_RT_dataLC_Cue1_Tdelay_Switch_l2.vi"() -> ("output_Cue1_Tdelay_Switch_l2"=w426:i32)  [unwired: 11 in]
              n289 = call "myRIO_BRig_RT_dataLC_Cue1_Block_Switch_l2.vi"() -> ("output_Cue1_Block_Switch_l2"=w427:i32)  [unwired: 11 in]
              n290 = call "myRIO_BRig_RT_dataLC_Cue1_Count_Switch_l2.vi"() -> ("output_Cue1_Count_Switch_l2"=w428:i32)  [unwired: 11 in]
              n291 = call "myRIO_BRig_RT_dataLC_Cue1_Probability_Switch_l2.vi"() -> ("output_Cue1_l2_First_Probability"=w429:i32)  [unwired: 11 in]
              n292 = call "myRIO_BRig_RT_dataLC_Cue1_OnOff_NS_l2.vi"() -> ("output_Cue1_OnOff_NS_l2"=w420:i32)  [unwired: 11 in]
              n293 = call "myRIO_BRig_RT_dataLC_Cue1_Tdelay_NS_l2.vi"() -> ("output_Cue1_Tdelay_NS_l2"=w421:i32)  [unwired: 11 in]
              n294 = call "myRIO_BRig_RT_dataLC_Cue1_Block_NS_l2.vi"() -> ("output_Cue1_Block_NS_l2"=w422:i32)  [unwired: 11 in]
              n295 = call "myRIO_BRig_RT_dataLC_Cue1_Count_NS_l2.vi"() -> ("output_Cue1_Count_NS_l2"=w423:i32)  [unwired: 11 in]
              n296 = call "myRIO_BRig_RT_dataLC_Cue1_Probability_NS_l2.vi"() -> ("output_Cue1_l2_All_Probability"=w424:i32)  [unwired: 11 in]
              n297 = call "myRIO_BRig_RT_dataLC_ENL1_delayOpt_Switch_l2.vi"() -> ("output_ENL1_delayOpt_Switch_l2"=w416:i32)  [unwired: 11 in]
              n298 = call "myRIO_BRig_RT_dataLC_ENL1_delayOpt_NS_l2.vi"() -> ("output_ENL1_delayOpt_NS_l2"=w417:i32)  [unwired: 11 in]
              n299 = call "myRIO_BRig_RT_dataLC_Cue1_delayOpt_Switch_l2.vi"() -> ("output_Cue1_delayOpt_Switch_l2"=w418:i32)  [unwired: 11 in]
              n300 = call "myRIO_BRig_RT_dataLC_Cue1_delayOpt_NS_l2.vi"() -> ("output_Cue1_delayOpt_NS_l2"=w419:i32)  [unwired: 11 in]
              n301 = Index Array(array=w469, index #1=w435, index #2=w436, index #3=w437, index #4=w438, index #5=w439, index #6=w430, index #7=w431, index #8=w432, index #9=w433, index #10=w434, index #11=w425, index #12=w426, index #13=w427, index #14=w428, index #15=w429, index #16=w420, index #17=w421, index #18=w422, index #19=w423, index #20=w424, index #21=w416, index #22=w417, index #23=w418, index #24=w419) -> (element #1=w467:u16, element #2=w466:u16, element #3=w465:u16, element #4=w464:u16, element #5=w463:u16, element #6=w462:u16, element #7=w461:u16, element #8=w460:u16, element #9=w459:u16, element #10=w458:u16, element #11=w457:u16, element #12=w456:u16, element #13=w455:u16, element #14=w454:u16, element #15=w453:u16, element #16=w452:u16, element #17=w451:u16, element #18=w450:u16, element #19=w449:u16, element #20=w448:u16, element #21=w443:u16, element #22=w442:u16, element #23=w441:u16, element #24=w440:u16)
              n302 = Not Equal To 0?(x=w467) -> (x != 0?=w471:bool)
              n303 = Not Equal To 0?(x=w462) -> (x != 0?=w470:bool)
              n304 = Not Equal To 0?(x=w457) -> (x != 0?=w473:bool)
              n305 = Not Equal To 0?(x=w452) -> (x != 0?=w472:bool)
              n306 = Not Equal To 0?(x=w443) -> (x != 0?=w445:bool)
              n307 = Not Equal To 0?(x=w442) -> (x != 0?=w446:bool)
              n308 = Not Equal To 0?(x=w441) -> (x != 0?=w447:bool)
              n309 = Not Equal To 0?(x=w440) -> (x != 0?=w444:bool)
              n310 = local write "LC_ENL1_OnOff_Switch_l2"(w471) -> ()
              n311 = local write "LC_ENL1_Tdelay_Switch_l2"(w466) -> ()
              n312 = local write "LC_ENL1_Block_Switch_l2"(w465) -> ()
              n313 = local write "LC_ENL1_Count_Switch_l2"(w464) -> ()
              n314 = local write "LC_ENL1_Probability_Switch_l2"(w463) -> ()
              n315 = local write "LC_ENL1_OnOff_NS_l2"(w470) -> ()
              n316 = local write "LC_ENL1_Tdelay_NS_l2"(w461) -> ()
              n317 = local write "LC_ENL1_Block_NS_l2"(w460) -> ()
              n318 = local write "LC_ENL1_Count_NS_l2"(w459) -> ()
              n319 = local write "LC_ENL1_Probability_NS_l2"(w458) -> ()
              n320 = local write "LC_Cue1_OnOff_Switch_l2"(w473) -> ()
              n321 = local write "LC_Cue1_Tdelay_Switch_l2"(w456) -> ()
              n322 = local write "LC_Cue1_Block_Switch_l2"(w455) -> ()
              n323 = local write "LC_Cue1_Count_Switch_l2"(w454) -> ()
              n324 = local write "LC_Cue1_Probability_Switch_l2"(w453) -> ()
              n325 = local write "LC_Cue1_OnOff_NS_l2"(w472) -> ()
              n326 = local write "LC_Cue1_Tdelay_NS_l2"(w451) -> ()
              n327 = local write "LC_Cue1_Block_NS_l2"(w450) -> ()
              n328 = local write "LC_Cue1_Count_NS_l2"(w449) -> ()
              n329 = local write "LC_Cue1_Probability_NS_l2"(w448) -> ()
              n330 = local write "LC_ENL1_delayOpt_Switch_l2"(w445) -> ()
              n331 = local write "LC_ENL1_delayOpt_NS_l2"(w446) -> ()
              n332 = local write "LC_Cue1_delayOpt_Switch_l2"(w447) -> ()
              n333 = local write "LC_Cue1_delayOpt_NS_l2"(w444) -> ()
            }
            frame "UploadSettings_dataLC_2" {
              # "Count"
              # "Tdelay"
              # "Prob"
              # "OnOff"
              # "Block"
              # "Selection NonSwitch"
              # "Count"
              # "Tdelay"
              # "Prob"
              # "OnOff"
              # "Block"
              # "Selection Switch"
              # "Trial"
              # "Tdelay"
              # "Prob"
              # "OnOff"
              # "Block"
              # "Wrong"
              # "Reward"
              # "Trial"
              # "Tdelay"
              # "Prob"
              # "OnOff"
              # "Block"
              n334 = call "myRIO_BRig_RT_dataLC_Reward_OnOff_l1.vi"() -> ("output_Reward_OnOff_l1"=w516:i32)  [unwired: 11 in]
              n335 = call "myRIO_BRig_RT_dataLC_Reward_Tdelay_l1.vi"() -> ("output_Reward_Tdelay_l1"=w515:i32)  [unwired: 11 in]
              n336 = call "myRIO_BRig_RT_dataLC_Reward_Block_l1.vi"() -> ("output_Reward_Block_l1"=w514:i32)  [unwired: 11 in]
              n337 = call "myRIO_BRig_RT_dataLC_Reward_Trial_l1.vi"() -> ("output_Reward_Trial_l1"=w513:i32)  [unwired: 11 in]
              n338 = call "myRIO_BRig_RT_dataLC_Reward_Probability_l1.vi"() -> ("output_Reward_Probability_l1"=w512:i32)  [unwired: 11 in]
              n339 = call "myRIO_BRig_RT_dataLC_Wrong_OnOff_l1.vi"() -> ("output_Wrong_OnOff_l1"=w505:i32)  [unwired: 11 in]
              n340 = call "myRIO_BRig_RT_dataLC_Wrong_Tdelay_l1.vi"() -> ("output_Wrong_Tdelay_l1"=w504:i32)  [unwired: 11 in]
              n341 = call "myRIO_BRig_RT_dataLC_Wrong_Block_l1.vi"() -> ("output_Wrong_Block_l1"=w503:i32)  [unwired: 11 in]
              n342 = call "myRIO_BRig_RT_dataLC_Wrong_Trial_l1.vi"() -> ("output_Wrong_Trial_l1"=w502:i32)  [unwired: 11 in]
              n343 = call "myRIO_BRig_RT_dataLC_Wrong_Probability_l1.vi"() -> ("output_Wrong_Probability_l1"=w501:i32)  [unwired: 11 in]
              n344 = call "myRIO_BRig_RT_dataLC_Selection_OnOff_Switch_l1.vi"() -> ("output_Selection_OnOff_Switch_l1"=w496:i32)  [unwired: 11 in]
              n345 = call "myRIO_BRig_RT_dataLC_Selection_Tdelay_Switch_l1.vi"() -> ("output_Selection_Tdelay_Switch_l1"=w495:i32)  [unwired: 11 in]
              n346 = call "myRIO_BRig_RT_dataLC_Selection_Block_Switch_l1.vi"() -> ("output_Selection_Block_Switch_l1"=w494:i32)  [unwired: 11 in]
              n347 = call "myRIO_BRig_RT_dataLC_Selection_Count_Switch_l1.vi"() -> ("output_Selection_Count_Switch_l1"=w493:i32)  [unwired: 11 in]
              n348 = call "myRIO_BRig_RT_dataLC_Selection_Probability_Switch_l1.vi"() -> ("output_Selection_Probability_Switch_l1"=w492:i32)  [unwired: 11 in]
              n349 = call "myRIO_BRig_RT_dataLC_Selection_OnOff_NS_l1.vi"() -> ("output_Selection_OnOff_NS_l1"=w491:i32)  [unwired: 11 in]
              n350 = call "myRIO_BRig_RT_dataLC_Selection_Tdelay_NS_l1.vi"() -> ("output_Selection_Tdelay_NS_l1"=w490:i32)  [unwired: 11 in]
              n351 = call "myRIO_BRig_RT_dataLC_Selection_Block_NS_l1.vi"() -> ("output_Selection_Block_NS_l1"=w489:i32)  [unwired: 11 in]
              n352 = call "myRIO_BRig_RT_dataLC_Selection_Count_NS_l1.vi"() -> ("output_Selection_Count_NS_l1"=w488:i32)  [unwired: 11 in]
              n353 = call "myRIO_BRig_RT_dataLC_Selection_Probability_NS_l1.vi"() -> ("output_Selection_Probability_NS_l1"=w487:i32)  [unwired: 11 in]
              n354 = Index Array(array=w517, index #1=w516, index #2=w515, index #3=w514, index #4=w513, index #5=w512, index #6=w505, index #7=w504, index #8=w503, index #9=w502, index #10=w501, index #11=w496, index #12=w495, index #13=w494, index #14=w493, index #15=w492, index #16=w491, index #17=w490, index #18=w489, index #19=w488, index #20=w487) -> (element #1=w511:u16, element #2=w510:u16, element #3=w509:u16, element #4=w508:u16, element #5=w507:u16, element #6=w506:u16, element #7=w500:u16, element #8=w499:u16, element #9=w498:u16, element #10=w497:u16, element #11=w484:u16, element #12=w483:u16, element #13=w482:u16, element #14=w481:u16, element #15=w480:u16, element #16=w479:u16, element #17=w478:u16, element #18=w477:u16, element #19=w476:u16, element #20=w475:u16)
              n355 = Not Equal To 0?(x=w511) -> (x != 0?=w519:bool)
              n356 = Not Equal To 0?(x=w506) -> (x != 0?=w518:bool)
              n357 = Not Equal To 0?(x=w484) -> (x != 0?=w486:bool)
              n358 = Not Equal To 0?(x=w479) -> (x != 0?=w485:bool)
              n359 = local write "LC_Reward_OnOff_l1"(w519) -> ()
              n360 = local write "LC_Reward_Tdelay_l1"(w510) -> ()
              n361 = local write "LC_Reward_Block_l1"(w509) -> ()
              n362 = local write "LC_Reward_Trial_l1"(w508) -> ()
              n363 = local write "LC_Reward_Probability_l1"(w507) -> ()
              n364 = local write "LC_Wrong_OnOff_l1"(w518) -> ()
              n365 = local write "LC_Wrong_Tdelay_l1"(w500) -> ()
              n366 = local write "LC_Wrong_Block_l1"(w499) -> ()
              n367 = local write "LC_Wrong_Trial_l1"(w498) -> ()
              n368 = local write "LC_Wrong_Probability_l1"(w497) -> ()
              n369 = local write "LC_Sel_OnOff_Switch_l1"(w486) -> ()
              n370 = local write "LC_Sel_Tdelay_Switch_l1"(w483) -> ()
              n371 = local write "LC_Sel_Block_Switch_l1"(w482) -> ()
              n372 = local write "LC_Sel_Count_Switch_l1"(w481) -> ()
              n373 = local write "LC_Sel_Probability_Switch_l1"(w480) -> ()
              n374 = local write "LC_Sel_OnOff_NS_l1"(w485) -> ()
              n375 = local write "LC_Sel_Tdelay_NS_l1"(w478) -> ()
              n376 = local write "LC_Sel_Block_NS_l1"(w477) -> ()
              n377 = local write "LC_Sel_Count_NS_l1"(w476) -> ()
              n378 = local write "LC_Sel_Probability_NS_l1"(w475) -> ()
            }
            frame "UploadSettings_dataLC_4" {
              # "Count"
              # "Tdelay"
              # "Prob"
              # "OnOff"
              # "Block"
              # "Selection NonSwitch"
              # "Count"
              # "Tdelay"
              # "Prob"
              # "OnOff"
              # "Block"
              # "Selection Switch"
              # "Trial"
              # "Tdelay"
              # "Prob"
              # "OnOff"
              # "Block"
              # "Wrong"
              # "Reward"
              # "Trial"
              # "Tdelay"
              # "Prob"
              # "OnOff"
              # "Block"
              n379 = call "myRIO_BRig_RT_dataLC_Reward_OnOff_l2.vi"() -> ("output_Reward_OnOff_l2"=w527:i32)  [unwired: 11 in]
              n380 = call "myRIO_BRig_RT_dataLC_Reward_Tdelay_l2.vi"() -> ("output_Reward_Tdelay_l2"=w528:i32)  [unwired: 11 in]
              n381 = call "myRIO_BRig_RT_dataLC_Reward_Block_l2.vi"() -> ("output_Reward_Block_l2"=w529:i32)  [unwired: 11 in]
              n382 = call "myRIO_BRig_RT_dataLC_Reward_Trial_l2.vi"() -> ("output_Reward_Trial_l2"=w530:i32)  [unwired: 11 in]
              n383 = call "myRIO_BRig_RT_dataLC_Reward_Probability_l2.vi"() -> ("output_Reward_Probability_l2"=w531:i32)  [unwired: 11 in]
              n384 = call "myRIO_BRig_RT_dataLC_Wrong_OnOff_l2.vi"() -> ("output_Wrong_OnOff_l2"=w522:i32)  [unwired: 11 in]
              n385 = call "myRIO_BRig_RT_dataLC_Wrong_Tdelay_l2.vi"() -> ("output_Wrong_Tdelay_l2"=w523:i32)  [unwired: 11 in]
              n386 = call "myRIO_BRig_RT_dataLC_Wrong_Block_l2.vi"() -> ("output_Wrong_Block_l2"=w524:i32)  [unwired: 11 in]
              n387 = call "myRIO_BRig_RT_dataLC_Wrong_Trial_l2.vi"() -> ("output_Wrong_Trial_l2"=w525:i32)  [unwired: 11 in]
              n388 = call "myRIO_BRig_RT_dataLC_Wrong_Probability_l2.vi"() -> ("output_Wrong_Probability_l2"=w526:i32)  [unwired: 11 in]
              n389 = call "myRIO_BRig_RT_dataLC_Selection_OnOff_Switch_l2.vi"() -> ("output_Selection_OnOff_Switch_l2"=w537:i32)  [unwired: 11 in]
              n390 = call "myRIO_BRig_RT_dataLC_Selection_Tdelay_Switch_l2.vi"() -> ("output_Selection_Tdelay_Switch_l2"=w538:i32)  [unwired: 11 in]
              n391 = call "myRIO_BRig_RT_dataLC_Selection_Block_Switch_l2.vi"() -> ("output_Selection_Block_Switch_l2"=w539:i32)  [unwired: 11 in]
              n392 = call "myRIO_BRig_RT_dataLC_Selection_Count_Switch_l2.vi"() -> ("output_Selection_Count_Switch_l2"=w540:i32)  [unwired: 11 in]
              n393 = call "myRIO_BRig_RT_dataLC_Selection_Probability_Switch_l2.vi"() -> ("output_Selection_Probability_Switch_l1"=w541:i32)  [unwired: 11 in]
              n394 = call "myRIO_BRig_RT_dataLC_Selection_OnOff_NS_l2.vi"() -> ("output_Selection_OnOff_NS_l2"=w532:i32)  [unwired: 11 in]
              n395 = call "myRIO_BRig_RT_dataLC_Selection_Tdelay_NS_l2.vi"() -> ("output_Selection_Tdelay_NS_l2"=w533:i32)  [unwired: 11 in]
              n396 = call "myRIO_BRig_RT_dataLC_Selection_Block_NS_l2.vi"() -> ("output_Selection_Block_NS_l2"=w534:i32)  [unwired: 11 in]
              n397 = call "myRIO_BRig_RT_dataLC_Selection_Count_NS_l2.vi"() -> ("output_Selection_Count_NS_l2"=w535:i32)  [unwired: 11 in]
              n398 = call "myRIO_BRig_RT_dataLC_Selection_Probability_NS_l2.vi"() -> ("output_Selection_Probability_NS_l2"=w536:i32)  [unwired: 11 in]
              n399 = Index Array(array=w564, index #1=w527, index #2=w528, index #3=w529, index #4=w530, index #5=w531, index #6=w522, index #7=w523, index #8=w524, index #9=w525, index #10=w526, index #11=w537, index #12=w538, index #13=w539, index #14=w540, index #15=w541, index #16=w532, index #17=w533, index #18=w534, index #19=w535, index #20=w536) -> (element #1=w563:u16, element #2=w562:u16, element #3=w561:u16, element #4=w560:u16, element #5=w559:u16, element #6=w558:u16, element #7=w557:u16, element #8=w556:u16, element #9=w555:u16, element #10=w554:u16, element #11=w551:u16, element #12=w550:u16, element #13=w549:u16, element #14=w548:u16, element #15=w547:u16, element #16=w546:u16, element #17=w545:u16, element #18=w544:u16, element #19=w543:u16, element #20=w542:u16)
              n400 = Not Equal To 0?(x=w563) -> (x != 0?=w566:bool)
              n401 = Not Equal To 0?(x=w558) -> (x != 0?=w565:bool)
              n402 = Not Equal To 0?(x=w551) -> (x != 0?=w553:bool)
              n403 = Not Equal To 0?(x=w546) -> (x != 0?=w552:bool)
              n404 = local write "LC_Reward_OnOff_l2"(w566) -> ()
              n405 = local write "LC_Reward_Tdelay_l2"(w562) -> ()
              n406 = local write "LC_Reward_Block_l2"(w561) -> ()
              n407 = local write "LC_Reward_Trial_l2"(w560) -> ()
              n408 = local write "LC_Reward_Probability_l2"(w559) -> ()
              n409 = local write "LC_Wrong_OnOff_l2"(w565) -> ()
              n410 = local write "LC_Wrong_Tdelay_l2"(w557) -> ()
              n411 = local write "LC_Wrong_Block_l2"(w556) -> ()
              n412 = local write "LC_Wrong_Trial_l2"(w555) -> ()
              n413 = local write "LC_Wrong_Probability_l2"(w554) -> ()
              n414 = local write "LC_Sel_OnOff_Switch_l2"(w553) -> ()
              n415 = local write "LC_Sel_Tdelay_Switch_l2"(w550) -> ()
              n416 = local write "LC_Sel_Block_Switch_l2"(w549) -> ()
              n417 = local write "LC_Sel_Count_Switch_l2"(w548) -> ()
              n418 = local write "LC_Sel_Probability_Switch_l2"(w547) -> ()
              n419 = local write "LC_Sel_OnOff_NS_l2"(w552) -> ()
              n420 = local write "LC_Sel_Tdelay_NS_l2"(w545) -> ()
              n421 = local write "LC_Sel_Block_NS_l2"(w544) -> ()
              n422 = local write "LC_Sel_Count_NS_l2"(w543) -> ()
              n423 = local write "LC_Sel_Probability_NS_l2"(w542) -> ()
            }
            frame "UploadSettings_dataMTrig_1" {
              # "Tdelay_R"
              # "Tdelay_L"
              # "Tcycle_R"
              # "Tcycle_L"
              # "RewCalib_nCycle_R"
              # "RewCalib_nCycle_L"
              # "Solenoid"
              # "Laser_Tcycle"
              n424 = call "myRIO_BRig_RT_dataMTrig_Laser_Tcycle.vi"() -> ("output_Laser_Tcycle"=w576:i32)  [unwired: 11 in]
              n425 = call "myRIO_BRig_RT_dataMTrig_Solenoid_RewCalib_nCycle__L.vi"() -> ("output_Solenoid_RewCalib_nCycle__L"=w575:i32)  [unwired: 11 in]
              n426 = call "myRIO_BRig_RT_dataMTrig_Solenoid_RewCalib_nCycle__R.vi"() -> ("output_Solenoid_RewCalib_nCycle__R"=w574:i32)  [unwired: 11 in]
              n427 = call "myRIO_BRig_RT_dataMTrig_Solenoid_Tdelay__L.vi"() -> ("output_Solenoid_Tdelay__L"=w571:i32)  [unwired: 11 in]
              n428 = call "myRIO_BRig_RT_dataMTrig_Solenoid_Tdelay__R.vi"() -> ("output_Solenoid_Tdelay__R"=w570:i32)  [unwired: 11 in]
              n429 = call "myRIO_BRig_RT_dataMTrig_Solenoid_Tcycle__L.vi"() -> ("output_Solenoid_Tcycle__L"=w573:i32)  [unwired: 11 in]
              n430 = call "myRIO_BRig_RT_dataMTrig_Solenoid_Tcycle__R.vi"() -> ("output_Solenoid_Tcycle__R"=w572:i32)  [unwired: 11 in]
              n431 = Index Array(array=w569, index #1=w576, index #2=w575, index #3=w574, index #4=w573, index #5=w572, index #6=w571, index #7=w570) -> (element #1=w583:u16, element #2=w582:u16, element #3=w581:u16, element #4=w580:u16, element #5=w579:u16, element #6=w578:u16, element #7=w577:u16)
              n432 = Replace Array Subset(array=w585, new element #1=w583, index #1=w576, new element #2=w582, index #2=w575, new element #3=w581, index #3=w574, new element #4=w580, index #4=w573, new element #5=w579, index #5=w572, new element #6=w578, index #6=w571, new element #7=w577, index #7=w570) -> (w584:u16[])
              n433 = local write "MTrig_Solenoid_Tcycle__L"(w580) -> ()
              n434 = local write "MTrig_Solenoid_Tcycle__R"(w579) -> ()
              n435 = local write "MTrig_Laser_Tcycle"(w583) -> ()
            }
            frame "Idle" {
              # "There are a number of tasks we need to perform\nwhile idling. To preserve our timing loop, we\nbreak up the IDLE state into smaller states"
              # "Laser_Tcycle"
              # "Audio_Tcycle_R"
              # "Audio_Tcycle_L"
              n436 = local read "Laser_power_min_l1"() -> (w594:dbl)
              n437 = local read "Laser_power_min_l2"() -> (w592:dbl)
              n438 = local read "Audio_Amp__R"() -> (w596:u16)
              n439 = local read "Audio_Amp__L"() -> (w598:u16)
              n440 = local read "Audio_Freq__R"() -> (w595:u8)
              n441 = local read "Audio_Freq__L"() -> (w597:u8)
              n442 = local read "CueLed_baseline"() -> (w587:bool)
              n443 = Select(t=myRIO_BRig_RT__Case_NonExp_stateList."SendData" ("Enum"), s="SendData", f=myRIO_BRig_RT__Case_NonExp_stateList."Idle_2" ("Enum")) -> (s? t:f=w603:T1)
              n444 = call "myRIO__convert__Voltage_to_FPGAvalue.vi"("input_voltage"=w594) -> ("output_PortC"=w593:i16)  [unwired: 9 in, 1 out]
              n445 = call "myRIO__convert__Voltage_to_FPGAvalue.vi"("input_voltage"=w592) -> ("output_PortC"=w591:i16)  [unwired: 9 in, 1 out]
              n446 = Select(t=myRIO_BRig_RT__Case_NonExp_stateList."TestConnection" ("Enum"), s="TestConnection", f=w603) -> (s? t:f=w607:T1)
              n447 = xnode "Read/Write Control"("FPGA VI Reference In"=w600, "error in"=w599, "audioAmp_L"=w598, "audioFreq_L_kHz"=w597, "audioAmp_R"=w596, "audioFreq_R_kHz"=w595, "AnaOut_0"=w593, "AnaOut_1"=w591, "CueLed_Baseline"=w587) -> ("error out"=w590:errorcluster)  [unwired: 1 out]
              n448 = call "myRIO_BRig_RT_dataMTrig_Audio_Tcycle__L.vi"() -> ("output_Audio_Tcycle__L"=w614:i32)  [unwired: 11 in]
              n449 = call "myRIO_BRig_RT_dataMTrig_Audio_Tcycle__R.vi"() -> ("output_Audio_Tcycle__R"=w613:i32)  [unwired: 11 in]
              n450 = call "myRIO_BRig_RT_dataMTrig_Laser_Tcycle.vi"() -> ("output_Laser_Tcycle"=w612:i32)  [unwired: 11 in]
              n451 = call "myRIO_BRig_RT_dataMTrig_CueLed_Tcycle.vi"() -> ("output_CueLed_Tcycle"=w589:i32)  [unwired: 11 in]
              n452 = local write "error out"(w590) -> ()
              n453 = local read "Tcycle_Cue_Audio_min"() -> (w602:u16)
              n454 = local read "MTrig_Laser_Tcycle"() -> (w601:u16)
              n455 = local read "Tcycle_Cue_LED_min"() -> (w588:u16)
              n456 = Replace Array Subset(array=w610, new element #1=w602, index #1=w614, new element #2=w602, index #2=w613, new element #3=w601, index #3=w612, new element #4=w588, index #4=w589) -> (w611:u16[])
            }
            frame "Idle_2" {
              w637 = u16 0 ("t")
              # "There are a number of tasks we need to perform\nwhile idling. To preserve our timing loop, we\nbreak up the IDLE state into smaller states"
              # "Ncycles"
              # "Ncycles"
              # "RewCalib"
              # "RewCalib"
              # "Solenoid R"
              # "Solenoid L"
              n457 = local read "MTrig_Laser_Switch"() -> (w630:bool)
              n458 = local read "count_warmup_R"() -> (w636:u16)
              n459 = local read "count_warmup_L"() -> (w641:u16)
              n460 = call "myRIO_BRig_RT_dataMTrig_Solenoid_RewCalib_OnOff__R.vi"() -> ("output_Solenoid_RewCalib_OnOff__R"=w652:i32)  [unwired: 11 in]
              n461 = call "myRIO_BRig_RT_dataMTrig_Solenoid_N__R.vi"() -> ("output_Solenoid_N__R"=w651:i32)  [unwired: 11 in]
              n462 = call "myRIO_BRig_RT_dataMTrig_Solenoid_RewCalib_OnOff__L.vi"() -> ("output_Solenoid_RewCalib_OnOff__L"=w667:i32)  [unwired: 11 in]
              n463 = call "myRIO_BRig_RT_dataMTrig_Solenoid_N__L.vi"() -> ("output_Solenoid_N__L"=w655:i32)  [unwired: 11 in]
              n464 = case shown="False" w630 {
                tunnel: "LR_reward_Event" -> [w673 w677]
                tunnel: "LR_wrong_Event" -> [w672 w676]
                tunnel: "LR_reward_Laser" -> [w671 w675]
                tunnel: "LR_wrong_Laser" -> [w670 w674]
                tunnel: [w673 _] -> w625
                tunnel: [w672 _] -> w624
                tunnel: [w671 _] -> w623
                tunnel: [w670 _] -> w622
                tunnel: [_ w677] -> w621
                tunnel: [_ w676] -> w620
                tunnel: [_ w675] -> w619
                tunnel: [_ w674] -> w618
                frame False {
                }
                frame True {
                }
              }
              n465 = Index Array(array=w658, index #1=w667, index #2=w655, index #3=w652, index #4=w651) -> (element #1=w654:u16, element #2=w649:u16, element #3=w650:u16, element #4=w648:u16)
              n466 = Select(t=w637, s="count_warmup_L_reset", f=w641) -> (s? t:f=→"count_warmup_L":u16)
              n467 = Select(t=w637, s="count_warmup_R_reset", f=w636) -> (s? t:f=→"count_warmup_R":u16)
              n468 = local read "RewCalib_Trig_L"() -> (w647:bool)
              n469 = local read "RewCalib_Trig_R"() -> (w646:bool)
              n470 = Equal To 0?(x=w649) -> (x = 0?=w657:bool)
              n471 = Equal To 0?(x=w648) -> (x = 0?=w656:bool)
              n472 = Not Equal To 0?(x=w650) -> (x != 0?=w668:bool)
              n473 = Not Equal To 0?(x=w654) -> (x != 0?=w669:bool)
              n474 = And(x=w657, y=w656) -> (x .and. y?=w661:bool)
              n475 = Or(x=w647, y=w646) -> (x .or. y?=w662:bool)
              n476 = Not Exclusive Or(1:w669, 2:w647) -> (0:w664:bool)
              n477 = xnode "Read/Write Control"("FPGA VI Reference In"=w616, "error in"=w617, "Left(F)_or_Right(T)"="Left(F)_or_Right(T)", "SelectionState"="SelectionState", "ignoreWrong"="ignoreWrong", "LR_reward_Event_l1"=w625, "LR_wrong_Event_l1"=w624, "LR_reward_Laser_l1"=w623, "LR_wrong_Laser_l1"=w622, "LR_reward_Event_l2"=w621, "LR_wrong_Event_l2"=w620, "LR_reward_Laser_l2"=w619, "LR_wrong_laser_l2"=w618) -> ("error out"=w615:errorcluster, "SelectReward"=→"SelectReward":bool, "SelectWrong"=→"SelectWrong":bool)  [unwired: 1 out]
              n478 = Not Exclusive Or(1:w668, 2:w646) -> (0:w666:bool)
              n479 = And(x=w662, y=w661) -> (x .and. y?=w644:bool)
              n480 = Not(x=w664) -> (.not. x?=w663:bool)
              n481 = Not(x=w666) -> (.not. x?=w665:bool)
              n482 = Or(x=w663, y=w665) -> (x .or. y?=w645:bool)
              n483 = Or(x=w644, y=w645) -> (x .or. y?=w660:bool)
              n484 = local write "error out"(w615) -> ()
              n485 = Select(t=myRIO_BRig_RT__Case_NonExp_stateList."RewardCalibration_pre" ("Enum"), s=w660, f=myRIO_BRig_RT__Case_NonExp_stateList."Idle_3" ("Enum")) -> (s? t:f=w643:T1)
            }
            frame "Idle_3" {
              # "There are a number of tasks we need to perform\nwhile idling. To preserve our timing loop, we\nbreak up the IDLE state into smaller states"
              n486 = local read "Laser_Tshutter_l1"() -> (w696:dbl)
              n487 = local read "Laser_duration_l1"() -> (w695:u16)
              n488 = local read "Laser_Tshutter_l2"() -> (w692:dbl)
              n489 = local read "Laser_duration_l2"() -> (w691:u16)
              n490 = local read "Laser_Tpeak_l1"() -> (w698:dbl)
              n491 = local read "Laser_Tpeak_l2"() -> (w694:dbl)
              n492 = local read "CueLed_Tpeak"() -> (w689:dbl)
              n493 = local read "Laser_Freq_l1"() -> (w697:dbl)
              n494 = local read "Laser_Freq_l2"() -> (w693:dbl)
              n495 = local read "CueLed_Freq"() -> (w688:dbl)
              n496 = local read "FPGA_count2ms"() -> (w690:dbl)
              n497 = To Unsigned Word Integer(number=w690) -> (unsigned 16bit integer=w699:u16)
              n498 = call "myRIO_BRig_RT__calc_laser_FPGA_N.vi"("input_FPGA_ms2count"=w690, "input_Tpeak"=w698, "input_Freq"=w697, "input_Tshutter"=w696, "input_duration"=w695) -> ("output_laser_Npeak"=w687:u32, "output_laser_Nvalley"=w685:u32, "output_laser_Nshutter"=w683:u32, "output_laser_Nduration"=w681:u32)  [unwired: 6 in, 1 out]
              n499 = call "myRIO_BRig_RT__calc_laser_FPGA_N.vi"("input_FPGA_ms2count"=w690, "input_Tpeak"=w694, "input_Freq"=w693, "input_Tshutter"=w692, "input_duration"=w691) -> ("output_laser_Npeak"=w686:u32, "output_laser_Nvalley"=w684:u32, "output_laser_Nshutter"=w682:u32, "output_laser_Nduration"=w680:u32)  [unwired: 6 in, 1 out]
              n500 = call "myRIO_BRig_RT__calc_laser_FPGA_N__CueLed.vi"("input_FPGA_ms2count"=w690, "input_Tpeak"=w689, "input_Freq"=w688) -> ("output_laser_Npeak"=w679:u32, "output_laser_Nvalley"=w678:u32)  [unwired: 11 in]
              n501 = xnode "Read/Write Control"("FPGA VI Reference In"=w704, "error in"=w703, "k1__counter_per_ms"=w699, "LC_nPeak_l1"=w687, "LC_nPeak_l2"=w686, "LC_nValley_l1"=w685, "LC_nValley_l2"=w684, "LC_nShutter_l1"=w683, "LC_nShutter_l2"=w682, "LR_reward_nTotal_l1"=w681, "LR_wrong_nTotal_l1"=w681, "LR_reward_nTotal_l2"=w680, "LR_wrong_nTotal_l2"=w680, "CueLed_nPeak"=w679, "CueLed_nValley"=w678) -> ("error out"=w700:errorcluster)  [unwired: 1 out]
              n502 = local write "error out"(w700) -> ()
            }
            frame "Idle_4" {
              w726 = u8 0 ("f")
              # "There are a number of tasks we need to perform\nwhile idling. To preserve our timing loop, we\nbreak up the IDLE state into smaller states"
              n503 = local read "MTrig_Solenoid_trig__L"() -> (w717:bool)
              n504 = local read "MTrig_Solenoid_trig__R"() -> (w727:bool)
              n505 = local read "warmupType"() -> (w710:u8)
              n506 = local read "warmup"() -> (w719:bool)
              n507 = Not Equal To 0?(x=w710) -> (x != 0?=w709:bool)
              n508 = Not(x=w709) -> (.not. x?=w720:bool)
              n509 = Select(t=u8 1, s=w717, f=w726) -> (s? t:f=w725:u8)
              n510 = Select(t=u8 2, s=w727, f=w726) -> (s? t:f=w724:u8)
              n511 = And(x=w719, y=w720) -> (x .and. y?=w718:bool)
              n512 = And(x=w719, y=w709) -> (x .and. y?=w713:bool)
              n513 = Add(x=w725, y=w724) -> (x+y=w723:u8)
              n514 = case shown="3" w723 {
                tunnel: w722 -> [w730 w734 w767 w798]
                tunnel: [w730 w733 w766 w797] -> w721
                tunnel: w718 -> [_ w732 w765 w796]
                tunnel: [_ TRUE TRUE TRUE] -> w715
                frame 0, Default {
                }
                frame 1 {
                  n515 = case shown="False" w732 {
                    tunnel: w734 -> [w747 w762]
                    tunnel: [w746 w761] -> w733
                    frame True {
                      # "Audio_L"
                      # "Solenoid_L"
                      n516 = call "myRIO_BRig_RT_dataMTrig_Solenoid_N__L.vi"() -> ("output_Solenoid_N__L"=w744:i32)  [unwired: 11 in]
                      n517 = call "myRIO_BRig_RT_dataMTrig_Audio_N__L.vi"() -> ("output_Audio_N__L"=w742:i32)  [unwired: 11 in]
                      n518 = call "myRIO_BRig_RT_dataMTrig_Audio_N__R.vi"() -> ("output_Audio_N__R"=w737:i32)  [unwired: 11 in]
                      n519 = local read "sp_LeftSpout"() -> (w741:u16)
                      n520 = Index Array(array=w747, index #1=w744, index #2=w742, index #3=w737) -> (element #1=w745:u16, element #2=w740:u16, element #3=w739:u16)
                      n521 = Increment(x=w745) -> (x+1=w743:u16)
                      n522 = case shown="2" w741 {
                        tunnel: w740 -> [w750 w753 w755]
                        tunnel: w739 -> [w748 w752 w757]
                        tunnel: [w749 w753 w754] -> w738
                        tunnel: [w748 w751 w756] -> w736
                        frame 0, Default {
                          n523 = Increment(x=w750) -> (x+1=w749:u16)
                        }
                        frame 1 {
                          n524 = Increment(x=w752) -> (x+1=w751:u16)
                        }
                        frame 2 {
                          n525 = Increment(x=w757) -> (x+1=w756:u16)
                          n526 = Increment(x=w755) -> (x+1=w754:u16)
                        }
                      }
                      n527 = Replace Array Subset(array=w747, new element #1=w743, index #1=w744, new element #2=w738, index #2=w742, new element #3=w736, index #3=w737) -> (w746:u16[])
                    }
                    frame False {
                      # "Solenoid_L"
                      n528 = call "myRIO_BRig_RT_dataMTrig_Solenoid_N__L.vi"() -> ("output_Solenoid_N__L"=w759:i32)  [unwired: 11 in]
                      n529 = Index Array(array=w762, index=w759) -> (element=w760:u16)
                      n530 = Increment(x=w760) -> (x+1=w758:u16)
                      n531 = Replace Array Subset(array=w762, new element=w758, index=w759) -> (w761:u16[])
                    }
                  }
                  n532 = local write "MTrig_Solenoid_trig__L"(FALSE) -> ()
                }
                frame 2 {
                  n533 = case shown="True" w765 {
                    tunnel: w767 -> [w779 w794]
                    tunnel: [w778 w793] -> w766
                    frame True {
                      # "Solenoid_R"
                      n534 = call "myRIO_BRig_RT_dataMTrig_Solenoid_N__R.vi"() -> ("output_Solenoid_N__R"=w768:i32)  [unwired: 11 in]
                      n535 = call "myRIO_BRig_RT_dataMTrig_Audio_N__L.vi"() -> ("output_Audio_N__L"=w775:i32)  [unwired: 11 in]
                      n536 = call "myRIO_BRig_RT_dataMTrig_Audio_N__R.vi"() -> ("output_Audio_N__R"=w770:i32)  [unwired: 11 in]
                      n537 = local read "sp_RightSpout"() -> (w774:u16)
                      n538 = Index Array(array=w779, index #1=w768, index #2=w775, index #3=w770) -> (element #1=w777:u16, element #2=w773:u16, element #3=w772:u16)
                      n539 = Increment(x=w777) -> (x+1=w776:u16)
                      n540 = case shown="2" w774 {
                        tunnel: w773 -> [w782 w785 w787]
                        tunnel: w772 -> [w780 w784 w789]
                        tunnel: [w781 w785 w786] -> w771
                        tunnel: [w780 w783 w788] -> w769
                        frame 0, Default {
                          n541 = Increment(x=w782) -> (x+1=w781:u16)
                        }
                        frame 1 {
                          n542 = Increment(x=w784) -> (x+1=w783:u16)
                        }
                        frame 2 {
                          n543 = Increment(x=w789) -> (x+1=w788:u16)
                          n544 = Increment(x=w787) -> (x+1=w786:u16)
                        }
                      }
                      n545 = Replace Array Subset(array=w779, new element #1=w776, index #1=w768, new element #2=w771, index #2=w775, new element #3=w769, index #3=w770) -> (w778:u16[])
                    }
                    frame False {
                      # "Solenoid_R"
                      n546 = call "myRIO_BRig_RT_dataMTrig_Solenoid_N__R.vi"() -> ("output_Solenoid_N__R"=w790:i32)  [unwired: 11 in]
                      n547 = Index Array(array=w794, index=w790) -> (element=w792:u16)
                      n548 = Increment(x=w792) -> (x+1=w791:u16)
                      n549 = Replace Array Subset(array=w794, new element=w791, index=w790) -> (w793:u16[])
                    }
                  }
                  n550 = local write "MTrig_Solenoid_trig__R"(FALSE) -> ()
                }
                frame 3 {
                  w799 = FALSE
                  n551 = case shown="True" w796 {
                    tunnel: w798 -> [w813 w821]
                    tunnel: [w812 w820] -> w797
                    frame True {
                      # "Audio_R"
                      # "Solenoid_R"
                      # "Audio_L"
                      # "Solenoid_L"
                      n552 = call "myRIO_BRig_RT_dataMTrig_Solenoid_N__L.vi"() -> ("output_Solenoid_N__L"=w807:i32)  [unwired: 11 in]
                      n553 = call "myRIO_BRig_RT_dataMTrig_Audio_N__L.vi"() -> ("output_Audio_N__L"=w805:i32)  [unwired: 11 in]
                      n554 = call "myRIO_BRig_RT_dataMTrig_Solenoid_N__R.vi"() -> ("output_Solenoid_N__R"=w803:i32)  [unwired: 11 in]
                      n555 = call "myRIO_BRig_RT_dataMTrig_Audio_N__R.vi"() -> ("output_Audio_N__R"=w802:i32)  [unwired: 11 in]
                      n556 = Index Array(array=w813, index #1=w807, index #2=w805, index #3=w803, index #4=w802) -> (element #1=w811:u16, element #2=w810:u16, element #3=w809:u16, element #4=w808:u16)
                      n557 = Increment(x=w808) -> (x+1=w800:u16)
                      n558 = Increment(x=w811) -> (x+1=w806:u16)
                      n559 = Increment(x=w810) -> (x+1=w804:u16)
                      n560 = Increment(x=w809) -> (x+1=w801:u16)
                      n561 = Replace Array Subset(array=w813, new element #1=w806, index #1=w807, new element #2=w804, index #2=w805, new element #3=w801, index #3=w803, new element #4=w800, index #4=w802) -> (w812:u16[])
                    }
                    frame False {
                      # "Solenoid_R"
                      # "Solenoid_L"
                      n562 = call "myRIO_BRig_RT_dataMTrig_Solenoid_N__L.vi"() -> ("output_Solenoid_N__L"=w817:i32)  [unwired: 11 in]
                      n563 = call "myRIO_BRig_RT_dataMTrig_Solenoid_N__R.vi"() -> ("output_Solenoid_N__R"=w814:i32)  [unwired: 11 in]
                      n564 = Index Array(array=w821, index #1=w817, index #2=w814) -> (element #1=w819:u16, element #2=w818:u16)
                      n565 = Increment(x=w819) -> (x+1=w816:u16)
                      n566 = Increment(x=w818) -> (x+1=w815:u16)
                      n567 = Replace Array Subset(array=w821, new element #1=w816, index #1=w817, new element #2=w815, index #2=w814) -> (w820:u16[])
                    }
                  }
                  n568 = local write "MTrig_Solenoid_trig__L"(w799) -> ()
                  n569 = local write "MTrig_Solenoid_trig__R"(w799) -> ()
                }
              }
              n570 = local read "get_countPerMS"() -> (w708:bool)
              n571 = Select(t=myRIO_BRig_RT__Case_NonExp_stateList."Get_FPGA_count_per_ms" ("Enum"), s=w708, f=myRIO_BRig_RT__Case_NonExp_stateList."Idle_6" ("Enum")) -> (s? t:f=w706:T1)
              n572 = Select(t=myRIO_BRig_RT__Case_NonExp_stateList."Cue_pre", s=w713, f=myRIO_BRig_RT__Case_NonExp_stateList."DispenseWater_pre" ("Enum")) -> (s? t:f=w711:T1)
              n573 = Select(t=w711, s=w715, f=w706) -> (s? t:f=w716:T1)
            }
            frame "Idle_5" {
              w844 = u8 0 ("f")
              # "There are a number of tasks we need to perform\nwhile idling. To preserve our timing loop, we\nbreak up the IDLE state into smaller states"
              n574 = local read "MTrig_Solenoid_trig__L"() -> (w835:bool)
              n575 = local read "MTrig_Solenoid_trig__R"() -> (w845:bool)
              n576 = local read "warmupType"() -> (w823:u8)
              n577 = local read "Cue1Param_CueType_Switch"() -> (w822:u16)
              n578 = local read "warmup"() -> (w837:bool)
              n579 = Not Equal To 0?(x=w823) -> (x != 0?=w828:bool)
              n580 = Not(x=w828) -> (.not. x?=w838:bool)
              n581 = Select(t=u8 1, s=w835, f=w844) -> (s? t:f=w843:u8)
              n582 = Select(t=u8 2, s=w845, f=w844) -> (s? t:f=w842:u8)
              n583 = And(x=w837, y=w838) -> (x .and. y?=w836:bool)
              n584 = And(x=w837, y=w828) -> (x .and. y?=w831:bool)
              n585 = Add(x=w843, y=w842) -> (x+y=w841:u8)
              n586 = case shown="2" w841 {
                tunnel: w840 -> [w848 w853 w902 w952]
                tunnel: [w848 w852 w901 w951] -> w839
                tunnel: w836 -> [_ w851 w900 w950]
                tunnel: [_ TRUE TRUE TRUE] -> w833
                tunnel: w822 -> [_ w849 w898 w948]
                frame 0, Default {
                }
                frame 1 {
                  n587 = case shown="True" w851 {
                    tunnel: w853 -> [w858 w897]
                    tunnel: [w857 w896] -> w852
                    tunnel: w849 -> [w856 _]
                    frame True {
                      n588 = case shown="0, Default" w856 {
                        tunnel: [TRUE _ w890] -> w855
                        frame 0, Default {
                          # "Audio"
                        }
                        frame 1 {
                          # "LED"
                        }
                        frame 2 {
                          # "Audio or LED"
                          n589 = local read "Cue1Param_AudioLed_Probability_Switch"() -> (w892:u16)
                          n590 = call "myRIO__convert__Probability_to_TrueFalse.vi"("input_probability_u16"=w892) -> ("output_TF"=w891:bool)  [unwired: 10 in]
                          n591 = Not(x=w891) -> (.not. x?=w890:bool)
                        }
                      }
                      n592 = case shown="True" w855 {
                        tunnel: w858 -> [w870 w888]
                        tunnel: [w869 w887] -> w857
                        frame True {
                          n593 = call "myRIO_BRig_RT_dataMTrig_Solenoid_N__L.vi"() -> ("output_Solenoid_N__L"=w867:i32)  [unwired: 11 in]
                          n594 = call "myRIO_BRig_RT_dataMTrig_Audio_N__L.vi"() -> ("output_Audio_N__L"=w865:i32)  [unwired: 11 in]
                          n595 = call "myRIO_BRig_RT_dataMTrig_Audio_N__R.vi"() -> ("output_Audio_N__R"=w860:i32)  [unwired: 11 in]
                          n596 = local read "sp_LeftSpout"() -> (w864:u16)
                          n597 = Index Array(array=w870, index #1=w867, index #2=w865, index #3=w860) -> (element #1=w868:u16, element #2=w863:u16, element #3=w862:u16)
                          n598 = case shown="2" w864 {
                            tunnel: w863 -> [w873 w876 w878]
                            tunnel: w862 -> [w871 w875 w880]
                            tunnel: [w872 w876 w877] -> w861
                            tunnel: [w871 w874 w879] -> w859
                            frame 0, Default {
                              n599 = Increment(x=w873) -> (x+1=w872:u16)
                            }
                            frame 1 {
                              n600 = Increment(x=w875) -> (x+1=w874:u16)
                            }
                            frame 2 {
                              n601 = Increment(x=w880) -> (x+1=w879:u16)
                              n602 = Increment(x=w878) -> (x+1=w877:u16)
                            }
                          }
                          n603 = Increment(x=w868) -> (x+1=w866:u16)
                          n604 = Replace Array Subset(array=w870, new element #1=w866, index #1=w867, new element #2=w861, index #2=w865, new element #3=w859, index #3=w860) -> (w869:u16[])
                        }
                        frame False {
                          n605 = call "myRIO_BRig_RT_dataMTrig_Solenoid_N__L.vi"() -> ("output_Solenoid_N__L"=w885:i32)  [unwired: 11 in]
                          n606 = call "myRIO_BRig_RT_dataMTrig_CueLed_N.vi"() -> ("output_CueLed_N"=w883:i32)  [unwired: 11 in]
                          n607 = Index Array(array=w888, index #1=w885, index #2=w883) -> (element #1=w886:u16, element #2=w882:u16)
                          n608 = Increment(x=w886) -> (x+1=w884:u16)
                          n609 = Increment(x=w882) -> (x+1=w881:u16)
                          n610 = Replace Array Subset(array=w888, new element #1=w884, index #1=w885, new element #2=w881, index #2=w883) -> (w887:u16[])
                        }
                      }
                    }
                    frame False {
                      # "Solenoid_L"
                      n611 = call "myRIO_BRig_RT_dataMTrig_Solenoid_N__L.vi"() -> ("output_Solenoid_N__L"=w894:i32)  [unwired: 11 in]
                      n612 = Index Array(array=w897, index=w894) -> (element=w895:u16)
                      n613 = Increment(x=w895) -> (x+1=w893:u16)
                      n614 = Replace Array Subset(array=w897, new element=w893, index=w894) -> (w896:u16[])
                    }
                  }
                  n615 = local write "MTrig_Solenoid_trig__L"(FALSE) -> ()
                }
                frame 2 {
                  n616 = case shown="True" w900 {
                    tunnel: w902 -> [w907 w946]
                    tunnel: [w906 w945] -> w901
                    tunnel: w898 -> [w905 _]
                    frame True {
                      n617 = case shown="0, Default" w905 {
                        tunnel: [TRUE _ w939] -> w904
                        frame 0, Default {
                          # "Audio"
                        }
                        frame 1 {
                          # "LED"
                        }
                        frame 2 {
                          # "Audio or LED"
                          n618 = local read "Cue1Param_AudioLed_Probability_Switch"() -> (w941:u16)
                          n619 = call "myRIO__convert__Probability_to_TrueFalse.vi"("input_probability_u16"=w941) -> ("output_TF"=w940:bool)  [unwired: 10 in]
                          n620 = Not(x=w940) -> (.not. x?=w939:bool)
                        }
                      }
                      n621 = case shown="True" w904 {
                        tunnel: w907 -> [w919 w937]
                        tunnel: [w918 w936] -> w906
                        frame True {
                          n622 = call "myRIO_BRig_RT_dataMTrig_Solenoid_N__R.vi"() -> ("output_Solenoid_N__R"=w916:i32)  [unwired: 11 in]
                          n623 = call "myRIO_BRig_RT_dataMTrig_Audio_N__L.vi"() -> ("output_Audio_N__L"=w914:i32)  [unwired: 11 in]
                          n624 = call "myRIO_BRig_RT_dataMTrig_Audio_N__R.vi"() -> ("output_Audio_N__R"=w909:i32)  [unwired: 11 in]
                          n625 = local read "sp_RightSpout"() -> (w913:u16)
                          n626 = Index Array(array=w919, index #1=w916, index #2=w914, index #3=w909) -> (element #1=w917:u16, element #2=w912:u16, element #3=w911:u16)
                          n627 = case shown="2" w913 {
                            tunnel: w912 -> [w922 w925 w927]
                            tunnel: w911 -> [w920 w924 w929]
                            tunnel: [w921 w925 w926] -> w910
                            tunnel: [w920 w923 w928] -> w908
                            frame 0, Default {
                              n628 = Increment(x=w922) -> (x+1=w921:u16)
                            }
                            frame 1 {
                              n629 = Increment(x=w924) -> (x+1=w923:u16)
                            }
                            frame 2 {
                              n630 = Increment(x=w929) -> (x+1=w928:u16)
                              n631 = Increment(x=w927) -> (x+1=w926:u16)
                            }
                          }
                          n632 = Increment(x=w917) -> (x+1=w915:u16)
                          n633 = Replace Array Subset(array=w919, new element #1=w915, index #1=w916, new element #2=w910, index #2=w914, new element #3=w908, index #3=w909) -> (w918:u16[])
                        }
                        frame False {
                          n634 = call "myRIO_BRig_RT_dataMTrig_Solenoid_N__R.vi"() -> ("output_Solenoid_N__R"=w934:i32)  [unwired: 11 in]
                          n635 = call "myRIO_BRig_RT_dataMTrig_CueLed_N.vi"() -> ("output_CueLed_N"=w932:i32)  [unwired: 11 in]
                          n636 = Index Array(array=w937, index #1=w934, index #2=w932) -> (element #1=w935:u16, element #2=w931:u16)
                          n637 = Increment(x=w935) -> (x+1=w933:u16)
                          n638 = Increment(x=w931) -> (x+1=w930:u16)
                          n639 = Replace Array Subset(array=w937, new element #1=w933, index #1=w934, new element #2=w930, index #2=w932) -> (w936:u16[])
                        }
                      }
                    }
                    frame False {
                      # "Solenoid_R"
                      n640 = call "myRIO_BRig_RT_dataMTrig_Solenoid_N__R.vi"() -> ("output_Solenoid_N__R"=w943:i32)  [unwired: 11 in]
                      n641 = Index Array(array=w946, index=w943) -> (element=w944:u16)
                      n642 = Increment(x=w944) -> (x+1=w942:u16)
                      n643 = Replace Array Subset(array=w946, new element=w942, index=w943) -> (w945:u16[])
                    }
                  }
                  n644 = local write "MTrig_Solenoid_trig__R"(FALSE) -> ()
                }
                frame 3 {
                  w947 = FALSE
                  n645 = case shown="True" w950 {
                    tunnel: w952 -> [w956 w993]
                    tunnel: [w955 w992] -> w951
                    tunnel: w948 -> [w954 _]
                    frame True {
                      n646 = case shown="2" w954 {
                        tunnel: [TRUE _ w983] -> w953
                        frame 0, Default {
                          # "Audio"
                        }
                        frame 1 {
                          # "LED"
                        }
                        frame 2 {
                          # "Audio or LED"
                          n647 = local read "Cue1Param_AudioLed_Probability_Switch"() -> (w985:u16)
                          n648 = call "myRIO__convert__Probability_to_TrueFalse.vi"("input_probability_u16"=w985) -> ("output_TF"=w984:bool)  [unwired: 10 in]
                          n649 = Not(x=w984) -> (.not. x?=w983:bool)
                        }
                      }
                      n650 = case shown="True" w953 {
                        tunnel: w956 -> [w970 w981]
                        tunnel: [w969 w980] -> w955
                        frame True {
                          n651 = call "myRIO_BRig_RT_dataMTrig_Solenoid_N__L.vi"() -> ("output_Solenoid_N__L"=w958:i32)  [unwired: 11 in]
                          n652 = call "myRIO_BRig_RT_dataMTrig_Solenoid_N__R.vi"() -> ("output_Solenoid_N__R"=w967:i32)  [unwired: 11 in]
                          n653 = call "myRIO_BRig_RT_dataMTrig_Audio_N__L.vi"() -> ("output_Audio_N__L"=w965:i32)  [unwired: 11 in]
                          n654 = call "myRIO_BRig_RT_dataMTrig_Audio_N__R.vi"() -> ("output_Audio_N__R"=w961:i32)  [unwired: 11 in]
                          n655 = Index Array(array=w970, index #1=w958, index #2=w967, index #3=w965, index #4=w961) -> (element #1=w959:u16, element #2=w968:u16, element #3=w964:u16, element #4=w963:u16)
                          n656 = Increment(x=w959) -> (x+1=w957:u16)
                          n657 = Increment(x=w968) -> (x+1=w966:u16)
                          n658 = Increment(x=w963) -> (x+1=w960:u16)
                          n659 = Increment(x=w964) -> (x+1=w962:u16)
                          n660 = Replace Array Subset(array=w970, new element #1=w957, index #1=w958, new element #2=w966, index #2=w967, new element #3=w962, index #3=w965, new element #4=w960, index #4=w961) -> (w969:u16[])
                        }
                        frame False {
                          n661 = call "myRIO_BRig_RT_dataMTrig_Solenoid_N__L.vi"() -> ("output_Solenoid_N__L"=w971:i32)  [unwired: 11 in]
                          n662 = call "myRIO_BRig_RT_dataMTrig_Solenoid_N__R.vi"() -> ("output_Solenoid_N__R"=w978:i32)  [unwired: 11 in]
                          n663 = call "myRIO_BRig_RT_dataMTrig_CueLed_N.vi"() -> ("output_CueLed_N"=w976:i32)  [unwired: 11 in]
                          n664 = Index Array(array=w981, index #1=w971, index #2=w978, index #3=w976) -> (element #1=w973:u16, element #2=w979:u16, element #3=w975:u16)
                          n665 = Increment(x=w973) -> (x+1=w972:u16)
                          n666 = Increment(x=w979) -> (x+1=w977:u16)
                          n667 = Increment(x=w975) -> (x+1=w974:u16)
                          n668 = Replace Array Subset(array=w981, new element #1=w972, index #1=w971, new element #2=w977, index #2=w978, new element #3=w974, index #3=w976) -> (w980:u16[])
                        }
                      }
                    }
                    frame False {
                      n669 = call "myRIO_BRig_RT_dataMTrig_Solenoid_N__L.vi"() -> ("output_Solenoid_N__L"=w989:i32)  [unwired: 11 in]
                      n670 = call "myRIO_BRig_RT_dataMTrig_Solenoid_N__R.vi"() -> ("output_Solenoid_N__R"=w988:i32)  [unwired: 11 in]
                      n671 = Index Array(array=w993, index #1=w989, index #2=w988) -> (element #1=w991:u16, element #2=w987:u16)
                      n672 = Increment(x=w987) -> (x+1=w986:u16)
                      n673 = Increment(x=w991) -> (x+1=w990:u16)
                      n674 = Replace Array Subset(array=w993, new element #1=w990, index #1=w989, new element #2=w986, index #2=w988) -> (w992:u16[])
                    }
                  }
                  n675 = local write "MTrig_Solenoid_trig__L"(w947) -> ()
                  n676 = local write "MTrig_Solenoid_trig__R"(w947) -> ()
                }
              }
              n677 = local read "get_countPerMS"() -> (w827:bool)
              n678 = Select(t=myRIO_BRig_RT__Case_NonExp_stateList."Get_FPGA_count_per_ms" ("Enum"), s=w827, f=myRIO_BRig_RT__Case_NonExp_stateList."Idle_6" ("Enum")) -> (s? t:f=w825:T1)
              n679 = Select(t=myRIO_BRig_RT__Case_NonExp_stateList."Cue_pre", s=w831, f=myRIO_BRig_RT__Case_NonExp_stateList."DispenseWater_pre" ("Enum")) -> (s? t:f=w829:T1)
              n680 = Select(t=w829, s=w833, f=w825) -> (s? t:f=w834:T1)
            }
            frame "Idle_6" {
              # "There are a number of tasks we need to perform\nwhile idling. To preserve our timing loop, we\nbreak up the IDLE state into smaller states"
              # "use dataMTrig as it is one of the last to transfer"
              n681 = call "myRIO_BRig_RT_comm_webdav_uploadReceived_check_v2,0.vi"("input_dataName"="dataMTrig") -> ("output_Iexist"=w998:bool)  [unwired: 9 in, 1 out]
              n682 = Select(t=myRIO_BRig_RT__Case_NonExp_stateList."UploadSettings_pre" ("Enum"), s=w998, f=myRIO_BRig_RT__Case_NonExp_stateList."Idle") -> (s? t:f=w996:T1)
            }
            frame "Cue_pre" {
              w1005 = u16 0 ("new element/subarray")
              # "Audio cue or LED cue?"
              # "Audio, LED, or \"Audio or LED\""
              # "Right Audio?"
              # "Left Audio?"
              # "Left or Right?"
              # "Cue Audio?\n(T=Audio, F=LED)"
              # "Ncycle"
              # "count"
              # "Audio_R"
              # "Ncycle"
              # "count"
              # "Audio_L"
              n683 = local read "Cue1Param_CueType_Switch"() -> (w1029:u16)
              n684 = case shown="2" w1029 {
                tunnel: [TRUE _ w1047] -> w1001
                frame 0, Default {
                  # "Audio"
                }
                frame 1 {
                  # "LED"
                }
                frame 2 {
                  # "Audio or LED"
                  n685 = local read "Cue1Param_AudioLed_Probability_Switch"() -> (w1049:u16)
                  n686 = call "myRIO__convert__Probability_to_TrueFalse.vi"("input_probability_u16"=w1049) -> ("output_TF"=w1048:bool)  [unwired: 10 in]
                  n687 = Not(x=w1048) -> (.not. x?=w1047:bool)
                }
              }
              n688 = call "myRIO_BRig_RT_dataMTrig_Solenoid_N__L.vi"() -> ("output_Solenoid_N__L"=w1039:i32)  [unwired: 11 in]
              n689 = call "myRIO_BRig_RT_dataMTrig_Solenoid_N__R.vi"() -> ("output_Solenoid_N__R"=w1038:i32)  [unwired: 11 in]
              n690 = Index Array(array=w1035, index #1=w1039, index #2=w1038) -> (element #1=w1037:u16, element #2=w1036:u16)
              n691 = Not Equal To 0?(x=w1037) -> (x != 0?=w1025:bool)
              n692 = Not Equal To 0?(x=w1036) -> (x != 0?=w1024:bool)
              n693 = Not(x=w1001) -> (.not. x?=w1000:bool)
              n694 = And(x=w1001, y=w1025) -> (x .and. y?=w1019:bool)
              n695 = And(x=w1001, y=w1024) -> (x .and. y?=w1017:bool)
              n696 = Select(t=myRIO_BRig_RT__Case_NonExp_stateList."Cue", s=w1001, f=myRIO_BRig_RT__Case_NonExp_stateList."Cue") -> (s? t:f=w1027:T1)
              n697 = local read "sp_RightSpout"() -> (w1018:u16)
              n698 = local read "sp_LeftSpout"() -> (w1020:u16)
              n699 = Boolean To (0,1)(Boolean=w1000) -> (0, 1=w1003:i16)
              n700 = To Unsigned Word Integer(number=w1003) -> (unsigned 16bit integer=w1002:u16)
              n701 = case shown="0, Default" w1020 {
                tunnel: [w1043 _ w1045] -> w1016
                tunnel: [_ w1044 w1045] -> w1014
                tunnel: w1019 -> [w1043 w1044 w1045]
                frame 0, Default {
                }
                frame 1 {
                }
                frame 2 {
                }
              }
              n702 = case shown="0, Default" w1018 {
                tunnel: [w1040 _ w1042] -> w1015
                tunnel: [_ w1041 w1042] -> w1013
                tunnel: w1017 -> [w1040 w1041 w1042]
                frame 0, Default {
                }
                frame 1 {
                }
                frame 2 {
                }
              }
              n703 = call "myRIO_BRig_RT_dataMTrig_Audio_c__L.vi"() -> ("output_Audio_c__L"=w1033:i32)  [unwired: 11 in]
              n704 = call "myRIO_BRig_RT_dataMTrig_Audio_N__L.vi"() -> ("output_Audio_N__L"=w1032:i32)  [unwired: 11 in]
              n705 = call "myRIO_BRig_RT_dataMTrig_Audio_c__R.vi"() -> ("output_Audio_c__R"=w1031:i32)  [unwired: 11 in]
              n706 = call "myRIO_BRig_RT_dataMTrig_Audio_N__R.vi"() -> ("output_Audio_N__R"=w1030:i32)  [unwired: 11 in]
              n707 = call "myRIO_BRig_RT_dataMTrig_CueLed_c.vi"() -> ("output_CueLed_c"=w1006:i32)  [unwired: 11 in]
              n708 = call "myRIO_BRig_RT_dataMTrig_CueLed_N.vi"() -> ("output_CueLed_N"=w1004:i32)  [unwired: 11 in]
              n709 = Or(x=w1016, y=w1015) -> (x .or. y?=w1012:bool)
              n710 = Boolean To (0,1)(Boolean=w1012) -> (0, 1=w1010:i16)
              n711 = To Unsigned Word Integer(number=w1010) -> (unsigned 16bit integer=w1009:u16)
              n712 = Or(x=w1014, y=w1013) -> (x .or. y?=w1011:bool)
              n713 = Boolean To (0,1)(Boolean=w1011) -> (0, 1=w1008:i16)
              n714 = To Unsigned Word Integer(number=w1008) -> (unsigned 16bit integer=w1007:u16)
              n715 = Replace Array Subset(array=w1035, new element #1=w1005, index #1=w1033, new element #2=w1009, index #2=w1032, new element #3=w1005, index #3=w1031, new element #4=w1007, index #4=w1030, new element #5=w1005, index #5=w1006, new element #6=w1002, index #6=w1004) -> (w1034:u16[])
              n716 = Initialize Array(u16 0 ("element"), 1 ("dimension size")) -> (w1023:u16[])
            }
            frame "Cue" {
              # "warmupType\n0 = Cue with reward (not possible to be in this state with value==0)\n1 = Cue then reward\n2 = Cue then reward (no lick)"
              # "Audio cue"
              # "lick did not occur or warmupType==1"
              # "lick occurred?"
              # "Ncycle"
              # "Audio_R"
              # "Ncycle"
              # "Audio_L"
              n717 = local read "warmupType"() -> (w1059:u8)
              n718 = Greater?(x=w1065, y=w1064) -> (0:w1068:bool)
              n719 = Greater?(x=w1067, y=w1066) -> (0:w1063:bool)
              n720 = Or(x=w1063, y=w1068) -> (x .or. y?=w1057:bool)
              n721 = Equal?(x=w1059, y=u8 1) -> (x = y?=w1053:bool)
              n722 = Not(x=w1057) -> (.not. x?=w1056:bool)
              n723 = call "myRIO_BRig_RT_dataMTrig_Audio_N__L.vi"() -> ("output_Audio_N__L"=w1070:i32)  [unwired: 11 in]
              n724 = call "myRIO_BRig_RT_dataMTrig_Audio_N__R.vi"() -> ("output_Audio_N__R"=w1069:i32)  [unwired: 11 in]
              n725 = call "myRIO_BRig_RT_dataMTrig_CueLed_N.vi"() -> ("output_CueLed_N"=w1050:i32)  [unwired: 11 in]
              n726 = Or(x=w1056, y=w1053) -> (x .or. y?=w1054:bool)
              n727 = case shown="True" w1054 {
                tunnel: w1070 -> [w1076 w1097]
                tunnel: w1069 -> [w1075 w1096]
                tunnel: w1062 -> [w1078 w1091]
                tunnel: [w1077 w1091] -> w1061
                tunnel: w1060 -> [_ w1089]
                tunnel: [myRIO_BRig_RT__Case_NonExp_stateList."Idle" ("t") w1088] -> w1055
                tunnel: w1053 -> [_ w1087]
                tunnel: w1052 -> [_ w1083]
                tunnel: w1051 -> [_ w1082]
                tunnel: w1050 -> [_ w1081]
                frame False {
                  w1071 = u16 0 ("new element/subarray")
                  # "lick occurred and warmupType==2"
                  n728 = call "myRIO_BRig_RT_dataMTrig_Solenoid_N__R.vi"() -> ("output_Solenoid_N__R"=w1072:i32)  [unwired: 11 in]
                  n729 = call "myRIO_BRig_RT_dataMTrig_Solenoid_N__L.vi"() -> ("output_Solenoid_N__L"=w1073:i32)  [unwired: 11 in]
                  n730 = Replace Array Subset(array=w1078, new element #1=w1071, index #1=w1076, new element #2=w1071, index #2=w1075, new element #3=w1071, index #3=w1073, new element #4=w1071, index #4=w1072) -> (w1077:u16[])
                }
                frame True {
                  n731 = Not(x=w1087) -> (.not. x?=w1086:bool)
                  n732 = Index Array(array=w1091, index #1=w1097, index #2=w1096, index #3=w1081) -> (element #1=w1095:u16, element #2=w1094:u16, element #3=w1080:u16)
                  n733 = Equal To 0?(x=w1095) -> (x = 0?=w1093:bool)
                  n734 = Equal To 0?(x=w1094) -> (x = 0?=w1092:bool)
                  n735 = Equal To 0?(x=w1080) -> (x = 0?=w1079:bool)
                  n736 = Compound Arithmetic op=AND(w1093, w1092, w1079) -> (w1085:bool)
                  n737 = And(x=w1085, y=w1086) -> (x .and. y?=w1084:bool)
                  n738 = case shown="True" w1084 {
                    tunnel: w1083 -> [_ w1105]
                    tunnel: w1082 -> [_ w1100]
                    frame False {
                    }
                    frame True {
                      n739 = local read "count_warmup_R"() -> (w1098:u16)
                      n740 = local read "count_warmup_L"() -> (w1103:u16)
                      n741 = Increment(x=w1098) -> (x+1=w1101:u16)
                      n742 = Increment(x=w1103) -> (x+1=w1104:u16)
                      n743 = Select(t=w1101, s=w1100, f=w1098) -> (s? t:f=w1099:u16)
                      n744 = Select(t=w1104, s=w1105, f=w1103) -> (s? t:f=w1102:u16)
                      n745 = local write "count_warmup_R"(w1099) -> ()
                      n746 = local write "count_warmup_L"(w1102) -> ()
                    }
                  }
                  n747 = Select(t=myRIO_BRig_RT__Case_NonExp_stateList."DispenseWater_pre", s=w1085, f=w1089) -> (s? t:f=w1088:T1)
                }
              }
            }
            frame "Cue_LED" {
              # "LED Cue"
              # "lick did not occur or warmupType==1"
              # "lick occurred?"
              n748 = local read "warmupType"() -> (w1118:u8)
              n749 = Greater?(x=w1124, y=w1123) -> (0:w1127:bool)
              n750 = Greater?(x=w1126, y=w1125) -> (0:w1122:bool)
              n751 = Or(x=w1122, y=w1127) -> (x .or. y?=w1116:bool)
              n752 = Equal?(x=w1118, y=u8 1) -> (x = y?=w1112:bool)
              n753 = Not(x=w1116) -> (.not. x?=w1115:bool)
              n754 = Or(x=w1115, y=w1112) -> (x .or. y?=w1113:bool)
              n755 = case shown="True" w1113 {
                tunnel: w1121 -> [w1134 w1154]
                tunnel: [w1133 w1154] -> w1120
                tunnel: w1119 -> [_ w1140]
                tunnel: [myRIO_BRig_RT__Case_NonExp_stateList."Idle" ("t") w1153] -> w1114
                tunnel: w1112 -> [_ w1139]
                tunnel: w1111 -> [_ w1151]
                tunnel: w1110 -> [_ w1150]
                tunnel: w1109 -> [w1128 w1149]
                tunnel: [w1128 w1142] -> w1108
                tunnel: w1107 -> [_ w1137]
                tunnel: w1106 -> [_ w1136]
                frame False {
                  w1129 = u16 0 ("new element/subarray")
                  # "lick occurred and warmupType==2"
                  n756 = call "myRIO_BRig_RT_dataMTrig_Solenoid_N__R.vi"() -> ("output_Solenoid_N__R"=w1130:i32)  [unwired: 11 in]
                  n757 = call "myRIO_BRig_RT_dataMTrig_Solenoid_N__L.vi"() -> ("output_Solenoid_N__L"=w1131:i32)  [unwired: 11 in]
                  n758 = Replace Array Subset(array=w1134, new element #1=w1129, new element #2=w1129, index #2=w1131, new element #3=w1129, index #3=w1130) -> (w1133:u16[])  [unwired: 1 in]
                }
                frame True {
                  w1147 = 0 ("index")
                  n759 = local read "Tcycle_Cue_LED_min"() -> (w1143:u16)
                  n760 = Index Array(array=w1149, index=w1147) -> (element=w1148:u16)
                  n761 = Increment(x=w1148) -> (x+1=w1146:u16)
                  n762 = Multiply(x=w1146, y=u16 5) -> (x*y=w1144:u16)
                  n763 = Replace Array Subset(array=w1149, new element=w1146, index=w1147) -> (w1142:u16[])
                  n764 = Less?(x=w1144, y=w1143) -> (x < y?=w1138:bool)
                  n765 = Not Or(1:w1139, 2:w1138) -> (0:w1152:bool)
                  n766 = case shown="True" w1152 {
                    tunnel: w1151 -> [_ w1162]
                    tunnel: w1150 -> [_ w1157]
                    frame False {
                    }
                    frame True {
                      n767 = local read "count_warmup_R"() -> (w1155:u16)
                      n768 = local read "count_warmup_L"() -> (w1160:u16)
                      n769 = Increment(x=w1155) -> (x+1=w1158:u16)
                      n770 = Increment(x=w1160) -> (x+1=w1161:u16)
                      n771 = Select(t=w1158, s=w1157, f=w1155) -> (s? t:f=w1156:u16)
                      n772 = Select(t=w1161, s=w1162, f=w1160) -> (s? t:f=w1159:u16)
                      n773 = local write "count_warmup_R"(w1156) -> ()
                      n774 = local write "count_warmup_L"(w1159) -> ()
                    }
                  }
                  n775 = Select(t=w1140, s=w1138, f=myRIO_BRig_RT__Case_NonExp_stateList."DispenseWater_pre" ("t")) -> (s? t:f=w1153:T1)
                  n776 = xnode "Read/Write Control"("FPGA VI Reference In"=w1137, "error in"=w1136, "CueLed_Event"=w1138) -> ("error out"=w1135:errorcluster)  [unwired: 1 out]
                  n777 = local write "error out"(w1135) -> ()
                }
              }
            }
            frame "RewardCalibration_pre" {
              (unwired) FALSE
              w1163 = FALSE
              w1174 = u8 0
              w1190 = u8 0
              # "Are we starting a RewardCalibration?\nOr are we stopping a RewardCalibration?\nOr is a RewardCalibration over?"
              # "RewCalib\nOnOff"
              # "N"
              # "Solenoid R"
              # "RewCalib\nOnOff"
              # "N"
              # "Solenoid L"
              n778 = local read "RewCalib_Trig_L"() -> (w1197:bool)
              n779 = local read "RewCalib_Trig_R"() -> (w1166:bool)
              n780 = call "myRIO_BRig_RT_dataMTrig_Solenoid_N__R.vi"() -> ("output_Solenoid_N__R"=w1168:i32)  [unwired: 11 in]
              n781 = call "myRIO_BRig_RT_dataMTrig_Solenoid_RewCalib_OnOff__R.vi"() -> ("output_Solenoid_RewCalib_OnOff__R"=w1165:i32)  [unwired: 11 in]
              n782 = call "myRIO_BRig_RT_dataMTrig_Solenoid_N__L.vi"() -> ("output_Solenoid_N__L"=w1183:i32)  [unwired: 11 in]
              n783 = call "myRIO_BRig_RT_dataMTrig_Solenoid_RewCalib_OnOff__L.vi"() -> ("output_Solenoid_RewCalib_OnOff__L"=w1184:i32)  [unwired: 11 in]
              n784 = Index Array(array=w1167, index #1=w1168, index #2=w1165) -> (element #1=w1178:u16, element #2=w1173:u16)
              n785 = Index Array(array=w1167, index #1=w1183, index #2=w1184) -> (element #1=w1194:u16, element #2=w1189:u16)
              n786 = Equal To 0?(x=w1178) -> (x = 0?=w1179:bool)
              n787 = Not Equal To 0?(x=w1173) -> (x != 0?=w1176:bool)
              n788 = Equal To 0?(x=w1194) -> (x = 0?=w1195:bool)
              n789 = Not Equal To 0?(x=w1189) -> (x != 0?=w1192:bool)
              n790 = local write "MTrig_Solenoid_trig__L"(w1163) -> ()
              n791 = local write "MTrig_Solenoid_trig__R"(w1163) -> ()
              n792 = Select(t=u8 1, s=w1166, f=w1174) -> (s? t:f=w1170:u8)
              n793 = Select(t=u8 1, s=w1197, f=w1190) -> (s? t:f=w1186:u8)
              n794 = Select(t=u8 2, s=w1179, f=w1174) -> (s? t:f=w1171:u8)
              n795 = Select(t=u8 4, s=w1176, f=w1174) -> (s? t:f=w1172:u8)
              n796 = Select(t=u8 2, s=w1195, f=w1190) -> (s? t:f=w1187:u8)
              n797 = Select(t=u8 4, s=w1192, f=w1190) -> (s? t:f=w1188:u8)
              n798 = Compound Arithmetic op=ADD(w1170, w1171, w1172) -> (w1169:u8)
              n799 = Compound Arithmetic op=ADD(w1186, w1187, w1188) -> (w1185:u8)
              n800 = case shown="7" w1185 {
                tunnel: w1167 -> [w1227 w1232 w1234 w1239 w1244 w1246 w1249 w1254]
                tunnel: [w1227 w1233 w1234 w1240 w1245 w1246 w1250 w1255] -> w1182
                tunnel: w1184 -> [_ w1230 _ w1237 w1242 _ w1248 w1253]
                tunnel: w1183 -> [_ w1231 _ w1238 w1243 _ _ _]
                frame 0, Default {
                }
                frame 1 {
                  n801 = Replace Array Subset(array=w1232, new element #1=u16 100 ("new element/subarray"), index #1=w1231, new element #2=u16 1 ("new element/subarray"), index #2=w1230) -> (w1233:u16[])
                }
                frame 2 {
                }
                frame 3 {
                  n802 = Replace Array Subset(array=w1239, new element #1=u16 100 ("new element/subarray"), index #1=w1238, new element #2=u16 1 ("new element/subarray"), index #2=w1237) -> (w1240:u16[])
                }
                frame 4 {
                  w1241 = u16 0 ("new element/subarray")
                  n803 = Replace Array Subset(array=w1244, new element #1=w1241, index #1=w1243, new element #2=w1241, index #2=w1242) -> (w1245:u16[])
                }
                frame 5 {
                }
                frame 6 {
                  n804 = Replace Array Subset(array=w1249, new element=u16 0 ("new element/subarray"), index=w1248) -> (w1250:u16[])
                }
                frame 7 {
                  n805 = local write "RewCalib_Trig_L"(FALSE ("RewCalib_Trig_L")) -> ()
                  n806 = Replace Array Subset(array=w1254, new element=u16 0 ("new element/subarray"), index=w1253) -> (w1255:u16[])
                }
              }
              n807 = case shown="7" w1169 {
                tunnel: w1182 -> [w1198 w1203 w1205 w1210 w1215 w1217 w1220 w1225]
                tunnel: [w1198 w1204 w1205 w1211 w1216 w1217 w1221 w1226] -> w1181
                tunnel: w1165 -> [_ w1201 _ w1208 w1213 _ w1219 w1224]
                tunnel: w1168 -> [_ w1202 _ w1209 w1214 _ _ _]
                frame 0, Default {
                }
                frame 1 {
                  n808 = Replace Array Subset(array=w1203, new element #1=u16 100 ("new element/subarray"), index #1=w1202, new element #2=u16 1 ("new element/subarray"), index #2=w1201) -> (w1204:u16[])
                }
                frame 2 {
                }
                frame 3 {
                  n809 = Replace Array Subset(array=w1210, new element #1=u16 100 ("new element/subarray"), index #1=w1209, new element #2=u16 1 ("new element/subarray"), index #2=w1208) -> (w1211:u16[])
                }
                frame 4 {
                  w1212 = u16 0 ("new element/subarray")
                  n810 = Replace Array Subset(array=w1215, new element #1=w1212, index #1=w1214, new element #2=w1212, index #2=w1213) -> (w1216:u16[])
                }
                frame 5 {
                }
                frame 6 {
                  n811 = Replace Array Subset(array=w1220, new element=u16 0 ("new element/subarray"), index=w1219) -> (w1221:u16[])
                }
                frame 7 {
                  n812 = local write "RewCalib_Trig_R"(FALSE ("RewCalib_Trig_L")) -> ()
                  n813 = Replace Array Subset(array=w1225, new element=u16 0 ("new element/subarray"), index=w1224) -> (w1226:u16[])
                }
              }
            }
            frame "DispenseWater_pre" {
              w1261 = u16 0 ("t")
              w1304 = u16 0 ("new element/subarray")
              # "just trust me on this one"
              # "RewCalib\nOnOff"
              # "RewCalib\nOnOff"
              # "nCycle"
              # "Solenoid__R"
              # "Tdelay"
              # "delay"
              # "nCycle"
              # "Solenoid__L"
              # "Tdelay"
              # "delay"
              # "Solenoid__R"
              # "count"
              # "Solenoid_Tcycle_R"
              # "Solenoid_Tcycle_L"
              # "Solenoid__L"
              # "count"
              n814 = call "myRIO_BRig_RT_dataMTrig_Solenoid_RewCalib_OnOff__L.vi"() -> ("output_Solenoid_RewCalib_OnOff__L"=w1268:i32)  [unwired: 11 in]
              n815 = call "myRIO_BRig_RT_dataMTrig_Solenoid_N__L.vi"() -> ("output_Solenoid_N__L"=w1259:i32)  [unwired: 11 in]
              n816 = call "myRIO_BRig_RT_dataMTrig_Solenoid_delay__L.vi"() -> ("output_Solenoid_delay__L"=w1302:i32)  [unwired: 11 in]
              n817 = call "myRIO_BRig_RT_dataMTrig_Solenoid_Tdelay__L.vi"() -> ("output_Solenoid_Tdelay__L"=w1301:i32)  [unwired: 11 in]
              n818 = call "myRIO_BRig_RT_dataMTrig_Solenoid_N__R.vi"() -> ("output_Solenoid_N__R"=w1257:i32)  [unwired: 11 in]
              n819 = call "myRIO_BRig_RT_dataMTrig_Solenoid_delay__R.vi"() -> ("output_Solenoid_delay__R"=w1291:i32)  [unwired: 11 in]
              n820 = call "myRIO_BRig_RT_dataMTrig_Solenoid_Tdelay__R.vi"() -> ("output_Solenoid_Tdelay__R"=w1290:i32)  [unwired: 11 in]
              n821 = call "myRIO_BRig_RT_dataMTrig_Solenoid_RewCalib_OnOff__R.vi"() -> ("output_Solenoid_RewCalib_OnOff__R"=w1264:i32)  [unwired: 11 in]
              n822 = Index Array(array=w1303, index #1=w1259, index #2=w1302, index #3=w1301, index #4=w1257, index #5=w1291, index #6=w1290, index #7=w1268, index #8=w1264) -> (element #1=w1260:u16, element #2=w1300:u16, element #3=w1295:u16, element #4=w1263:u16, element #5=w1285:u16, element #6=w1284:u16, element #7=w1269:u16, element #8=w1266:u16)
              n823 = Equal To 0?(x=w1300) -> (x = 0?=w1299:bool)
              n824 = Equal To 0?(x=w1285) -> (x = 0?=w1289:bool)
              n825 = local read "RewCalib_Trig_L"() -> (w1280:bool)
              n826 = local read "RewCalib_Trig_R"() -> (w1275:bool)
              n827 = Not Equal To 0?(x=w1260) -> (x != 0?=w1298:bool)
              n828 = Not Equal To 0?(x=w1263) -> (x != 0?=w1288:bool)
              n829 = local read "MTrig_Solenoid_Tcycle__L"() -> (w1297:u16)
              n830 = local read "MTrig_Solenoid_Tcycle__R"() -> (w1283:u16)
              n831 = Not Equal To 0?(x=w1269) -> (x != 0?=w1279:bool)
              n832 = Not Equal To 0?(x=w1266) -> (x != 0?=w1277:bool)
              n833 = Not(x=w1280) -> (.not. x?=w1278:bool)
              n834 = Not(x=w1275) -> (.not. x?=w1276:bool)
              n835 = And(x=w1279, y=w1278) -> (x .and. y?=w1274:bool)
              n836 = And(x=w1277, y=w1276) -> (x .and. y?=w1273:bool)
              n837 = call "myRIO_BRig_RT_dataMTrig_Solenoid_c__L.vi"() -> ("output_Solenoid_c__L"=w1306:i32)  [unwired: 11 in]
              n838 = call "myRIO_BRig_RT_dataMTrig_Solenoid_c__R.vi"() -> ("output_Solenoid_c__R"=w1305:i32)  [unwired: 11 in]
              n839 = Select(t=w1297, s=w1298, f=u16 0) -> (s? t:f=w1294:u16)
              n840 = Or(x=w1274, y=w1273) -> (x .or. y?=w1262:bool)
              n841 = Select(t=w1283, s=w1288, f=u16 0) -> (s? t:f=w1286:u16)
              n842 = Select(t=w1294, s=w1299, f=w1295) -> (s? t:f=w1292:u16)
              n843 = Select(t=w1286, s=w1289, f=w1284) -> (s? t:f=w1281:u16)
              n844 = call "myRIO_BRig_RT_dataMTrig_Solenoid_Tcycle__L.vi"() -> ("output_Solenoid_Tcycle__L"=w1293:i32)  [unwired: 11 in]
              n845 = call "myRIO_BRig_RT_dataMTrig_Solenoid_Tcycle__R.vi"() -> ("output_Solenoid_Tcycle__R"=w1282:i32)  [unwired: 11 in]
              n846 = Select(t=w1261, s=w1262, f=w1260) -> (s? t:f=w1258:u16)
              n847 = Select(t=w1261, s=w1262, f=w1263) -> (s? t:f=w1256:u16)
              n848 = Select(t=myRIO_BRig_RT__Case_NonExp_stateList."Idle" ("Enum"), s=w1262, f=myRIO_BRig_RT__Case_NonExp_stateList."DispenseWater" ("Enum")) -> (s? t:f=w1270:T1)
              n849 = Select(t=w1261, s=w1262, f=w1269) -> (s? t:f=w1267:u16)
              n850 = Select(t=w1261, s=w1262, f=w1266) -> (s? t:f=w1265:u16)
              n851 = Replace Array Subset(array=w1303, new element #1=w1304, index #1=w1306, new element #2=w1304, index #2=w1305, new element #3=w1292, index #3=w1293, new element #4=w1281, index #4=w1282, new element #5=w1267, index #5=w1268, new element #6=w1265, index #6=w1264, new element #7=w1258, index #7=w1259, new element #8=w1256, index #8=w1257) -> (w1307:u16[])
            }
            frame "DispenseWater" {
              # "D"
              # "C"
              # "B"
              # "A"
              # "(A) Add COUNT and INCREMENT\n(B) Is (A) smaller than Tcycle?\n(C) Are we dispensing water or in the delay phase?\n(D) If (A) is smaller than Tcycle   AND   if we are dispensing water\n      then send TRUE to solenoid"
              # "delay"
              # "Tcycle"
              # "Solenoid__R"
              # "count"
              # "delay"
              # "Tcycle"
              # "Solenoid__L"
              # "count"
              n852 = To Unsigned Word Integer(number=w1334) -> (unsigned 16bit integer=w1316:u16)
              n853 = call "myRIO_BRig_RT_dataMTrig_Solenoid_delay__R.vi"() -> ("output_Solenoid_delay__R"=w1320:i32)  [unwired: 11 in]
              n854 = call "myRIO_BRig_RT_dataMTrig_Solenoid_c__R.vi"() -> ("output_Solenoid_c__R"=w1319:i32)  [unwired: 11 in]
              n855 = call "myRIO_BRig_RT_dataMTrig_Solenoid_Tcycle__R.vi"() -> ("output_Solenoid_Tcycle__R"=w1321:i32)  [unwired: 11 in]
              n856 = call "myRIO_BRig_RT_dataMTrig_Solenoid_delay__L.vi"() -> ("output_Solenoid_delay__L"=w1336:i32)  [unwired: 11 in]
              n857 = call "myRIO_BRig_RT_dataMTrig_Solenoid_c__L.vi"() -> ("output_Solenoid_c__L"=w1328:i32)  [unwired: 11 in]
              n858 = call "myRIO_BRig_RT_dataMTrig_Solenoid_Tcycle__L.vi"() -> ("output_Solenoid_Tcycle__L"=w1337:i32)  [unwired: 11 in]
              n859 = Index Array(array=w1330, index #1=w1328, index #2=w1337, index #3=w1336, index #4=w1319, index #5=w1321, index #6=w1320) -> (element #1=w1335:u16, element #2=w1325:u16, element #3=w1333:u16, element #4=w1315:u16, element #5=w1312:u16, element #6=w1311:u16)
              n860 = Add(x=w1335, y=w1316) -> (x+y=w1326:u16)
              n861 = Add(x=w1315, y=w1316) -> (x+y=w1317:u16)
              n862 = Less?(x=w1326, y=w1325) -> (x < y?=w1309:bool)
              n863 = Equal To 0?(x=w1333) -> (x = 0?=w1332:bool)
              n864 = Less?(x=w1317, y=w1312) -> (x < y?=w1310:bool)
              n865 = Equal To 0?(x=w1311) -> (x = 0?=w1318:bool)
              n866 = And(x=w1309, y=w1332) -> (x .and. y?=w1331:bool)
              n867 = Or(x=w1309, y=w1310) -> (x .or. y?=w1308:bool)
              n868 = And(x=w1310, y=w1318) -> (x .and. y?=w1313:bool)
              n869 = Select(t=w1326, s=w1309, f=w1325) -> (s? t:f=w1327:u16)
              n870 = Select(t=w1317, s=w1310, f=w1312) -> (s? t:f=w1314:u16)
              n871 = Replace Array Subset(array=w1330, new element #1=w1327, index #1=w1328, new element #2=w1314, index #2=w1319) -> (w1329:u16[])
              n872 = Select(t=w1324, s=w1308, f=myRIO_BRig_RT__Case_NonExp_stateList."DispenseWater_post" ("Enum")) -> (s? t:f=w1322:T1)
            }
            frame "DispenseWater_post" {
              # "nCycle"
              # "delay"
              # "Solenoid__R"
              # "nCycle"
              # "delay"
              # "Solenoid__L"
              n873 = call "myRIO_BRig_RT_dataMTrig_Solenoid_N__L.vi"() -> ("output_Solenoid_N__L"=w1354:i32)  [unwired: 11 in]
              n874 = call "myRIO_BRig_RT_dataMTrig_Solenoid_delay__L.vi"() -> ("output_Solenoid_delay__L"=w1353:i32)  [unwired: 11 in]
              n875 = call "myRIO_BRig_RT_dataMTrig_Solenoid_N__R.vi"() -> ("output_Solenoid_N__R"=w1350:i32)  [unwired: 11 in]
              n876 = call "myRIO_BRig_RT_dataMTrig_Solenoid_delay__R.vi"() -> ("output_Solenoid_delay__R"=w1349:i32)  [unwired: 11 in]
              n877 = Index Array(array=w1356, index #1=w1354, index #2=w1353, index #3=w1350, index #4=w1349) -> (element #1=w1358:u16, element #2=w1357:u16, element #3=w1341:u16, element #4=w1343:u16)
              n878 = Not Equal To 0?(x=w1358) -> (x != 0?=w1359:bool)
              n879 = Not Equal To 0?(x=w1341) -> (x != 0?=w1342:bool)
              n880 = case shown="True" w1342 {
                selector: w1342 -> [_ w1363]
                tunnel: w1341 -> [w1361 w1369]
                tunnel: w1343 -> [_ w1370]
                tunnel: [w1361 w1367] -> w1340
                tunnel: [u16 0 w1366] -> w1339
                tunnel: [_ w1363] -> w1338
                frame False {
                }
                frame True {
                  n881 = Equal To 0?(x=w1370) -> (x = 0?=w1362:bool)
                  n882 = Decrement(x=w1369) -> (x-1=w1368:u16)
                  n883 = Select(t=w1368, s=w1362, f=w1369) -> (s? t:f=w1367:u16)
                  n884 = Select(t=u16 1, s=w1362, f=u16 0) -> (s? t:f=w1366:u16)
                }
              }
              n885 = case shown="True" w1359 {
                selector: w1359 -> [_ w1374]
                tunnel: w1358 -> [w1372 w1380]
                tunnel: w1357 -> [_ w1381]
                tunnel: [w1372 w1378] -> w1352
                tunnel: [u16 0 w1377] -> w1351
                tunnel: [_ w1374] -> w1348
                frame False {
                }
                frame True {
                  n886 = Equal To 0?(x=w1381) -> (x = 0?=w1373:bool)
                  n887 = Decrement(x=w1380) -> (x-1=w1379:u16)
                  n888 = Select(t=w1379, s=w1373, f=w1380) -> (s? t:f=w1378:u16)
                  n889 = Select(t=u16 1, s=w1373, f=u16 0) -> (s? t:f=w1377:u16)
                }
              }
              n890 = Or(x=w1348, y=w1338) -> (x .or. y?=w1347:bool)
              n891 = Replace Array Subset(array=w1356, new element #1=w1352, index #1=w1354, new element #2=w1351, index #2=w1353, new element #3=w1340, index #3=w1350, new element #4=w1339, index #4=w1349) -> (w1355:u16[])
              n892 = Select(t=myRIO_BRig_RT__Case_NonExp_stateList."DispenseWater_pre" ("Enum"), s=w1347, f=myRIO_BRig_RT__Case_NonExp_stateList."Idle" ("Enum")) -> (s? t:f=w1344:T1)
            }
            frame "TestConnection" {
              n893 = local read "Host Password"() -> (w1387:string)
              n894 = local read "Host UserName"() -> (w1388:string)
              n895 = call "myRIO_BRig_RT_comm_webdav_testConnect.vi"("input_password"=w1387, "input_username"=w1388) -> ("output_Iconnected"=w1385:bool)  [unwired: 9 in]
              n896 = Select(t="Connection accepted!" ("message"), s=w1385, f="Error!") -> (s? t:f=w1383:string)
              n897 = One Button Dialog(message=w1383) -> ()  [unwired: 1 in, 1 out]
            }
            frame "SendData" {
              n898 = local read "Data Set Prefix"() -> (w1390:string)
              n899 = local read "Host Password"() -> (w1391:string)
              n900 = local read "Host UserName"() -> (w1392:string)
              n901 = call "myRIO_BRig_RT_comm_webdav_sendData_all.vi"("Host Filename Prefix"=w1390, "Host Password"=w1391, "Host UserName"=w1392) -> ()  [unwired: 9 in]
            }
            frame "Get_FPGA_count_per_ms" {
              # "Used to automatically determine how many FPGA cycles in 1 ms"
              n902 = case shown="False" w1405 {
                selector: w1405 -> [w1407 _]
                tunnel: w1403 -> [_ w1420]
                tunnel: [w1411 w1420] -> w1402
                tunnel: w1401 -> [w1410 w1418]
                tunnel: w1400 -> [w1409 w1417]
                tunnel: [w1408 w1415] -> w1395
                tunnel: [w1407 w1414] -> w1399
                frame False {
                  n903 = Get Date/Time In Seconds() -> (seconds since 1Jan1904=w1412:timestamp)
                  n904 = xnode "Read/Write Control"("FPGA VI Reference In"=w1410, "error in"=w1409, "timeTrial_trig"=TRUE ("timeTrial")) -> ("error out"=w1408:errorcluster)  [unwired: 1 out]
                  n905 = To Double Precision Float(number=w1412) -> (double precision float=w1411:dbl)
                  n906 = local write "get_countPerMS"(w1407) -> ()
                }
                frame True {
                  w1416 = 1.0
                  n907 = Get Date/Time In Seconds() -> (seconds since 1Jan1904=w1421:timestamp)
                  n908 = To Double Precision Float(number=w1421) -> (double precision float=w1422:dbl)
                  n909 = Subtract(x=w1422, y=w1420) -> (x-y=w1419:dbl)
                  n910 = Less Or Equal?(x=w1416, y=w1419) -> (x <= y?=w1414:bool)
                  n911 = case shown="True" w1414 {
                    tunnel: w1418 -> [_ w1435]
                    tunnel: w1417 -> [w1423 w1434]
                    tunnel: w1416 -> [_ w1425]
                    tunnel: [w1423 w1424] -> w1415
                    frame False {
                    }
                    frame True {
                      n912 = xnode "Read/Write Control"("FPGA VI Reference In"=w1435, "error in"=w1434) -> ("FPGA VI Reference Out"=w1432:refnum<k20>, "error out"=w1431:errorcluster, "timeTrial_count"=w1426:u32)
                      n913 = Multiply(x=w1425, y=1000.0) -> (x*y=w1429:dbl)
                      n914 = To Double Precision Float(number=w1426) -> (double precision float=w1428:dbl)
                      n915 = Divide(x=w1428, y=w1429) -> (x/y=w1430:dbl)
                      n916 = local write "FPGA_count2ms"(w1430) -> ()
                      n917 = xnode "Read/Write Control"("FPGA VI Reference In"=w1432, "error in"=w1431, "timeTrial_trig"=FALSE ("timeTrial")) -> ("error out"=w1424:errorcluster)  [unwired: 1 out]
                    }
                  }
                }
              }
              n918 = Select(t=myRIO_BRig_RT__Case_NonExp_stateList."Idle" ("Enum"), s=w1399, f=w1397) -> (s? t:f=w1396:T1)
              n919 = local write "error out"(w1395) -> ()
            }
            frame "End" {
            }
          }
          n920 = local read "MTrig_Audio_trig__R"() -> (w91:bool)
          n921 = local read "MTrig_Audio_trig__L"() -> (w92:bool)
          n922 = local read "MTrig_Laser_trig"() -> (w90:bool)
          n923 = local read "MTrig_CueLed"() -> (w83:bool)
          n924 = Compound Arithmetic op=OR(w92, w91, w90, w83) -> (w89:bool)
          n925 = local read "START"() -> (w115:bool)
          n926 = local read "STOP_abort"() -> (w114:bool)
          n927 = case shown="True" w89 {
            frame False {
            }
            frame True {
              w131 = FALSE
              n928 = local write "MTrig_Audio_trig__R"(w131) -> ()
              n929 = local write "MTrig_Audio_trig__L"(w131) -> ()
              n930 = local write "MTrig_Laser_trig"(w131) -> ()
              n931 = local write "MTrig_CueLed"(w131) -> ()
            }
          }
          n932 = call "myRIO_BRig_RT_dataMTrig_main__NoExp.vi"("input_dataMTrig"=w118, "input_Audio_trig_L"=w92, "input_Audio_trig_R"=w91, "input_Laser_trig"=w90, "input_CueLed"=w83) -> ("output_dataMTrig"=w117:u16[], "output_Audio_L"=w109:bool, "output_Audio_R"=w110:bool, "output_Laser"=w88:bool, "output_CueLed"=w82:bool)  [unwired: 10 in]
          n933 = Or(x=w115, y=w114) -> (x .or. y?=w113:bool)
          n934 = Select(t=myRIO_BRig_RT__Case_NonExp_stateList."End" ("Enum"), s=w113, f=w112) -> (s? t:f=w111:T1)
          n935 = Not(x="MTrig_Laser_Switch") -> (.not. x?=w85:bool)
          n936 = And(x=w88, y=w85) -> (x .and. y?=w86:bool)
          n937 = And(x=w88, y="MTrig_Laser_Switch") -> (x .and. y?=w87:bool)
          n938 = xnode "Read/Write Control"("FPGA VI Reference In"=w98, "error in"=w97, "A1_SR"=w119, "A3_SL"=w120, "audioTrigger_L"=w109, "audioTrigger_R"=w110, "LC_Laser_l1"=w86, "LC_Laser_l2"=w87, "CueLed_Event"=w82) -> ("FPGA VI Reference Out"=w125:refnum<k20>, "error out"=w124:errorcluster)
          n939 = node-c288() -> ()  [unwired: 1 in, 1 out]
          "cState_NonExp" <- w123
        }
        n940 = node-c288(w70) -> ()  [unwired: 1 out]
        n941 = flat-sequence {
          tunnel: w63 -> [w81]
          tunnel: [w81] -> w62
          tunnel: w61 -> [w80]
          tunnel: [w80] -> w60
          frame #0 {
            w79 = FALSE
            n942 = local write "STOP_endBlock"(w79) -> ()
            n943 = local write "STOP_endTrial"(w79) -> ()
          }
        }
      }
      frame True {
        w1449 = u16 0
        w1466 = u16 0 ("idxDataBlock")
        w1468 = u16 100 ("new element/subarray")
        w1469 = u16 100 ("new element/subarray")
        w1489 = T6 refnum items=["Session NI_WebDAV"] ("output_hSession")
        w1498 = FALSE
        # "dummyState counter"
        # "audio__L\naudio__R"
        # "Audio params"
        # "nRewards"
        # "idxDataBlock"
        # "Solenoid_Tdelay_R"
        # "Solenoid_Tdelay_L"
        # "RewCalib_N__R"
        # "RewCalib_N__L"
        # "Save dataLick to file\nSend file to Host\nSave dataMTrig\nSend file to Host\nDisconnect"
        # "dataTrial"
        # "dataTrial"
        # "Solenoid_Tcycle_R"
        # "Solenoid_Tcycle_L"
        # "Laser_Tcycle"
        # "Audio_Tcycle_R"
        # "Audio_Tcycle_L"
        # "dataLick"
        # "dataLC"
        # "dataLC"
        # "dataBlock"
        # "dataBlock"
        # "dataMTrig"
        # "dataMTrig"
        # "dataExp"
        # "dataCurrent"
        # "dataExp"
        # "dataCurrent"
        # "spout"
        # "state"
        n944 = call "myRIO_BRig_RT_dataMTrig_Solenoid_Tcycle__L.vi"() -> ("output_Solenoid_Tcycle__L"=w1495:i32)  [unwired: 11 in]
        n945 = call "myRIO_BRig_RT_dataMTrig_Solenoid_Tcycle__R.vi"() -> ("output_Solenoid_Tcycle__R"=w1494:i32)  [unwired: 11 in]
        n946 = call "myRIO_BRig_RT_dataMTrig_Audio_Tcycle__L.vi"() -> ("output_Audio_Tcycle__L"=w1493:i32)  [unwired: 11 in]
        n947 = call "myRIO_BRig_RT_dataMTrig_Audio_Tcycle__R.vi"() -> ("output_Audio_Tcycle__R"=w1492:i32)  [unwired: 11 in]
        n948 = call "myRIO_BRig_RT_dataMTrig_Laser_Tcycle.vi"() -> ("output_Laser_Tcycle"=w1491:i32)  [unwired: 11 in]
        n949 = local read "Tcycle_Reward_min_L"() -> (w1470:u16)
        n950 = local read "Tcycle_Reward_min_R"() -> (w1471:u16)
        n951 = local read "MTrig_Solenoid_Tcycle__L"() -> (w1474:u16)
        n952 = local read "MTrig_Solenoid_Tcycle__R"() -> (w1473:u16)
        n953 = local read "MTrig_Laser_Tcycle"() -> (w1472:u16)
        n954 = call "myRIO_BRig_RT_dataMTrig_Solenoid_RewCalib_nCycle__L.vi"() -> ("output_Solenoid_RewCalib_nCycle__L"=w1477:i32)  [unwired: 11 in]
        n955 = call "myRIO_BRig_RT_dataMTrig_Solenoid_Tdelay__L.vi"() -> ("output_Solenoid_Tdelay__L"=w1479:i32)  [unwired: 11 in]
        n956 = call "myRIO_BRig_RT_dataMTrig_Solenoid_RewCalib_nCycle__R.vi"() -> ("output_Solenoid_RewCalib_nCycle__R"=w1478:i32)  [unwired: 11 in]
        n957 = call "myRIO_BRig_RT_dataMTrig_Solenoid_Tdelay__R.vi"() -> ("output_Solenoid_Tdelay__R"=w1480:i32)  [unwired: 11 in]
        n958 = case shown="False" w1459 {
          selector: w1459 -> [_ w1520]
          tunnel: w1458 -> [w1517 w1522]
          tunnel: [w1518 w1522] -> w1454
          tunnel: w1457 -> [_ w1521]
          tunnel: [w1519 w1521] -> w1455
          tunnel: [w1516 w1520] -> w1453
          frame False {
            n959 = call "myRIO__TCP_connect_forWriting.vi"("input_error"=w1517) -> ("output_error"=w1518:errorcluster, "output_connected"=w1516:bool, "output_hTCP"=w1519:refnum<k5>)  [unwired: 8 in]
          }
          frame True {
          }
        }
        n960 = call "myRIO_BRig_RT_dataLick_init.vi"() -> ("output_dataLick"=w1500:u16[][])  [unwired: 11 in]
        n961 = call "myRIO_BRig_RT_dataCurrent_init.vi"() -> ("output_dataCurrent"=w1507:u16[])  [unwired: 11 in]
        n962 = call "myRIO_BRig_RT_dataExp_init.vi"() -> ("output_dataExp"=w1506:u16[])  [unwired: 11 in]
        n963 = call "myRIO_BRig_RT_dataMTrig_init.vi"() -> ("output_dataMTrig"=w1497:u16[])  [unwired: 5 in]
        n964 = call "myRIO_BRig_RT_dataLC_init.vi"() -> ("output_dataLC"=w1504:u16[])  [unwired: 11 in]
        n965 = call "myRIO_BRig_RT_dataBlock_init.vi"() -> ("output_dataBlock"=w1505:u16[][])  [unwired: 11 in]
        n966 = call "myRIO_BRig_RT_dataTrial_init.vi"() -> ("output_dataTrial"=w1490:u16[][])  [unwired: 11 in]
        n967 = local write "Threshold"(FALSE ("Threshold")) -> ()
        n968 = local write "I_connect_TCP"(w1453) -> ()
        n969 = Replace Array Subset(array=w1497, new element #1=w1469, index #1=w1477, new element #2=w1469, index #2=w1478, new element #3=w1468, index #3=w1479, new element #4=w1468, index #4=w1480, new element #5=w1474, index #5=w1495, new element #6=w1473, index #6=w1494, new element #7=w1470, index #7=w1493, new element #8=w1471, index #8=w1492, new element #9=w1472, index #9=w1491) -> (w1496:u16[])
        n970 = call "myRIO_BRig_RT_dataAnalog_init.vi"() -> ("output_dataAnalog"=w1464:u16[][])  [unwired: 11 in]
        n971 = call "myRIO_BRig_RT_TCP__start_exp.vi"("input_hTCP"=w1455, "input_I_connected_TCP"=w1453, "input_error"=w1454) -> ("output_hTCP"=w1452:refnum<k5>, "output_error"=w1451:errorcluster)  [unwired: 11 in]
        n972 = Get Date/Time In Seconds() -> (seconds since 1Jan1904=w1476:timestamp)
        n973 = call "myRIO_BRig_RT_arrTrig_init.vi"() -> ("output_arrTrig"=w1448:bool[])  [unwired: 11 in]
        n974 = To Double Precision Float(number=w1476) -> (double precision float=w1475:dbl)
        n975 = node-c288() -> (w1515:T3)  [unwired: 4 in]
        n976 = timed-loop {
          timing: w1515 -> [_]
          timing-out: [_] -> w1514
          shift-right: [w1649] -> _
          shift-left: myRIO_BRig_RT__Case_Exp_stateList."Start1" ("Enum") -> [w1573]
          shift-right: [w1607] -> _
          shift-left: enum16{"Left", "Right"}."Left" -> [w1689]
          tunnel: w1447 -> [w1687]
          tunnel: w1446 -> [w1579]
          shift-right: [w1682] -> _
          shift-left: w1512 -> [w1686]
          shift-right: [w1681] -> _
          shift-left: w1511 -> [w1685]
          tunnel: [w1665] -> w1509
          tunnel: [w1666] -> w1510
          shift-right: [w1667] -> w1481
          shift-left: w1507 -> [w1568]
          shift-right: [w1680] -> _
          shift-left: w1506 -> [w1640]
          shift-right: [w1661] -> w1485
          shift-left: w1496 -> [w1662]
          shift-right: [w1678] -> _
          shift-left: w1505 -> [w1679]
          shift-right: [w1676] -> _
          shift-left: w1504 -> [w1677]
          shift-right: [w1668] -> w1487
          shift-left: w1500 -> [w1669]
          shift-right: [w1638] -> _
          shift-left: w1498 -> [w1663]
          shift-right: [w1639] -> _
          shift-left: w1498 -> [w1664]
          shift-right: [w1647] -> _
          shift-left: w1490 -> [w1648]
          shift-right: [w1646] -> w1483
          shift-left: w1489 -> [w1644]
          shift-right: [w1645] -> w1484
          shift-left: FALSE ("output_Iconnected") -> [w1643]
          tunnel: "Data Set Prefix" -> [w1642]
          tunnel: [w1642] -> w1482
          tunnel: w1475 -> [w1641]
          shift-right: [w1636] -> _
          shift-left: 0 ("idxDataBlock") -> [w1637]
          shift-right: [w1633] -> _
          shift-left: w1466 -> [w1635]
          shift-right: [w1632] -> _
          shift-left: w1466 -> [w1634]
          shift-right: [w1626] -> w1462
          shift-left: 0 -> [w1612]
          shift-right: [w1608] -> _
          shift-left: w1449 -> [w1621]
          shift-right: [w1609] -> _
          shift-left: w1449 -> [w1618]
          shift-right: [w1617] -> _
          shift-left: w1449 -> [w1624]
          shift-right: [w1627] -> w1463
          shift-left: w1464 -> [w1628]
          tunnel: w1452 -> [w1616]
          tunnel: [w1615] -> w1461
          tunnel: w1453 -> [w1613]
          tunnel: [w1613] -> w1460
          tunnel: w1451 -> [w1614]
          tunnel: [w1576] -> w1456
          shift-right: [w1605] -> _
          shift-left: u16 0 -> [w1606]
          shift-right: [w1603] -> _
          shift-left: w1449 -> [w1604]
          shift-right: [w1600] -> _
          shift-left: w1448 -> [w1601]
          shift-right: [w1571] -> _
          shift-left: FALSE -> [w1574]
          stop <- w1675 stop-if-true
          # "arrTrig"
          # "arrTrig"
          # "LC_Laser_l2"
          # "LC_Event_l2"
          # "LC_Laser_l1"
          # "LC_Event_l1"
          # "CueLed"
          # "LC_Laser_l2"
          # "LC_Event_l2"
          # "LC_Laser_l1"
          # "LC_Event_l1"
          # "solenoid__R"
          # "solenoid__L"
          # "spout"
          # "iState"
          # "dataAnalog"
          # "index"
          # "iEvent"
          # "iBlock"
          # "iTrial"
          # "Laser"
          # "Audio R"
          # "Audio L"
          # "Solenoid R"
          # "Solenoid L"
          # "manual triggering"
          # "dataTrial"
          # "dataBlock"
          # "nRewards"
          # "dataExp"
          # "dataCurrent"
          # "audio__L\naudio__R"
          # "time stamp"
          # "nRewards"
          # "idxDataBlock"
          # "idxDataBlock"
          # "audio__L\naudio__R"
          # "dataLC"
          # "solenoid__R"
          # "solenoid__L"
          # "Did a lick occur?"
          # "Update lick counter"
          # "spout"
          # "spout"
          # "state"
          # "state"
          n977 = node-c288() -> ()  [unwired: 1 in, 1 out]
          n978 = flat-sequence {
            tunnel: w1579 -> [w1690]
            tunnel: [w1690] -> _
            tunnel: [w1691] -> w1575
            tunnel: [w1690] -> w1578
            frame #0 {
              n979 = Get Date/Time In Seconds() -> (seconds since 1Jan1904=w1691:timestamp)
            }
          }
          n980 = xnode "Read/Write Control"("FPGA VI Reference In"=w1687, "error in"=w1578) -> ("FPGA VI Reference Out"=w1631:refnum<k20>, "error out"=w1630:errorcluster, "A2_LickL"=w1682:u32, "A4_LickR"=w1681:u32)
          "A2" <- w1682
          "A4" <- w1681
          n981 = Greater?(x=w1682, y=w1686) -> (0:w1684:bool)
          n982 = Greater?(x=w1681, y=w1685) -> (0:w1683:bool)
          n983 = call "myRIO_BRig_RT_dataCurrent_IallReward_L.vi"() -> ("output_IallReward_L"=w1569:i32)  [unwired: 11 in]
          n984 = call "myRIO_BRig_RT_dataCurrent_IallReward_R.vi"() -> ("output_IallReward_R"=w1570:i32)  [unwired: 11 in]
          n985 = Or(x=w1684, y=w1683) -> (x .or. y?=w1688:bool)
          n986 = local read "MTrig_Solenoid_trig__L"() -> (w1659:bool)
          n987 = local read "MTrig_Solenoid_trig__R"() -> (w1658:bool)
          n988 = local read "MTrig_Audio_trig__L"() -> (w1657:bool)
          n989 = local read "MTrig_Audio_trig__R"() -> (w1656:bool)
          n990 = local read "MTrig_Laser_trig"() -> (w1655:bool)
          n991 = Index Array(array=w1568, index #1=w1569, index #2=w1570) -> (element #1=w1566:u16, element #2=w1567:u16)
          n992 = Not Equal To 0?(x=w1566) -> (x != 0?=→"allReward_L":bool)
          n993 = Not Equal To 0?(x=w1567) -> (x != 0?=→"allReward_R":bool)
          n994 = case shown="\"SelectReward\"" w1573 {
            selector: w1573 -> [_ _ _ _ _ _ _ _ _ _ _ _ _ _ _ _ _ _ _ _ _ _ _ _ _ w2656 _ w2699 _ _ _ _ _ w2796 _ w2856 _ _ _ _ _ w2959 _ w3011 _ w3066 _ w3106 _ _ w3164 _ _ _ _ _ w3311 _ _ _ _ _ _ _ _ _ _ _ _ w3544 w3573]
            tunnel: [myRIO_BRig_RT__Case_Exp_stateList."Start2" ("Enum") myRIO_BRig_RT__Case_Exp_stateList."Start3" ("Enum") myRIO_BRig_RT__Case_Exp_stateList."saveSettings1" ("Enum") myRIO_BRig_RT__Case_Exp_stateList."saveSettings2" ("Enum") myRIO_BRig_RT__Case_Exp_stateList."saveSettings3" ("Enum") myRIO_BRig_RT__Case_Exp_stateList."saveSettings4" ("Enum") myRIO_BRig_RT__Case_Exp_stateList."saveSettings_LC_ENL_l1" ("Enum") myRIO_BRig_RT__Case_Exp_stateList."saveSettings_LC_ENL_l2" ("Enum") myRIO_BRig_RT__Case_Exp_stateList."saveSettings_LC_Cue_l1" ("Enum") myRIO_BRig_RT__Case_Exp_stateList."saveSettings_LC_Cue_l2" ("Enum") myRIO_BRig_RT__Case_Exp_stateList."saveSettings6_LC_l1_Other" ("Enum") myRIO_BRig_RT__Case_Exp_stateList."SaveSettings6_LC_l2_Other" ("Enum") myRIO_BRig_RT__Case_Exp_stateList."setSettings_Audio" ("Enum") myRIO_BRig_RT__Case_Exp_stateList."setSettings_Laser" ("Enum") myRIO_BRig_RT__Case_Exp_stateList."commConnect" ("Enum") w2413 myRIO_BRig_RT__Case_Exp_stateList."initTrial" ("Enum") w2467 myRIO_BRig_RT__Case_Exp_stateList."initTrial3" ("Enum") myRIO_BRig_RT__Case_Exp_stateList."initTrial_LC_ENL1" ("Enum") myRIO_BRig_RT__Case_Exp_stateList."ENL1_pre" ("Enum") myRIO_BRig_RT__Case_Exp_stateList."initTrial_LC_Cue1" ("Enum") myRIO_BRig_RT__Case_Exp_stateList."initTrial_LC_Sel" ("Enum") myRIO_BRig_RT__Case_Exp_stateList."initTrial4" ("Enum") w2631 w2653 myRIO_BRig_RT__Case_Exp_stateList."ENL1Penalty" ("Enum") w2700 myRIO_BRig_RT__Case_Exp_stateList."endExp" ("Enum") myRIO_BRig_RT__Case_Exp_stateList."endExp" ("Enum") myRIO_BRig_RT__Case_Exp_stateList."endExp" ("Enum") myRIO_BRig_RT__Case_Exp_stateList."endExp" ("Enum") w2773 w2790 myRIO_BRig_RT__Case_Exp_stateList."Cue1Penalty" ("Enum") w2854 myRIO_BRig_RT__Case_Exp_stateList."endExp" ("Enum") myRIO_BRig_RT__Case_Exp_stateList."endExp" ("Enum") myRIO_BRig_RT__Case_Exp_stateList."endExp" ("Enum") myRIO_BRig_RT__Case_Exp_stateList."endExp" ("Enum") w2932 w2958 myRIO_BRig_RT__Case_Exp_stateList."SelectReward" ("Enum") w3012 myRIO_BRig_RT__Case_Exp_stateList."SelectRewardPost" ("Enum") w3067 myRIO_BRig_RT__Case_Exp_stateList."SelectWrong" ("Enum") w3102 myRIO_BRig_RT__Case_Exp_stateList."endTrial1" ("Enum") myRIO_BRig_RT__Case_Exp_stateList."SelectTimeout" ("Enum") w3166 myRIO_BRig_RT__Case_Exp_stateList."endTrial1" ("Enum") myRIO_BRig_RT__Case_Exp_stateList."endTrial2" ("Enum") myRIO_BRig_RT__Case_Exp_stateList."endTrial3" ("Enum") w3236 w3294 w3311 myRIO_BRig_RT__Case_Exp_stateList."initBlock" ("Enum") w3334 myRIO_BRig_RT__Case_Exp_stateList."commUpload_dataExp" ("Enum") myRIO_BRig_RT__Case_Exp_stateList."endBlock" ("Enum") myRIO_BRig_RT__Case_Exp_stateList."commUpload_dataLC" ("Enum") myRIO_BRig_RT__Case_Exp_stateList."commUpload_dataTrial" ("Enum") myRIO_BRig_RT__Case_Exp_stateList."commUpload_dataCurrent" ("Enum") myRIO_BRig_RT__Case_Exp_stateList."saveData_dataCurrent" ("Enum") myRIO_BRig_RT__Case_Exp_stateList."saveData_dataExp" ("Enum") myRIO_BRig_RT__Case_Exp_stateList."saveData_dataLC" ("Enum") myRIO_BRig_RT__Case_Exp_stateList."saveData_dataTrial" ("Enum") myRIO_BRig_RT__Case_Exp_stateList."commUpload_pre" ("Enum") w3543 w3572] -> w1649
            tunnel: [w1718 w1733 w1751 w1814 w1872 w1934 w1993 w2053 w2113 w2173 w2233 w2272 w2312 w2341 w2404 w2412 w2437 w2454 w2484 w2526 w2554 w2575 w2594 w2617 w2641 w2665 w2686 w2704 w2716 w2734 w2749 w2764 w2772 w2812 w2836 w2853 w2870 w2887 w2902 w2917 w2941 w2973 w2994 w3009 w3022 w3064 w3084 w3112 w3129 w3145 w3172 w3191 w3203 w3219 w3256 w3271 w3310 w3323 w3337 w3363 w3380 w3397 w3414 w3431 w3455 w3471 w3494 w3510 w3530 w3560 w3589] -> w1607
            tunnel: w1689 -> [w1718 w1733 w1751 w1814 w1872 w1934 w1993 w2053 w2113 w2173 w2233 w2272 w2312 w2341 w2404 w2414 w2437 w2454 w2484 w2526 w2554 w2575 w2594 w2617 w2641 w2665 w2686 w2704 w2716 w2734 w2749 w2764 w2772 w2812 w2836 w2853 w2870 w2887 w2902 w2917 w2941 w2973 w2994 w3009 w3022 w3064 w3084 w3112 w3129 w3145 w3172 w3191 w3203 w3219 w3256 w3271 w3310 w3323 w3337 w3363 w3380 w3397 w3414 w3431 w3455 w3471 w3494 w3510 w3530 w3560 w3589]
            tunnel: w1688 -> [w1721 w1736 w1748 w1817 w1875 w1937 w1996 w2056 w2116 w2176 w2236 w2275 w2315 w2344 w2407 w2429 w2444 w2468 w2503 w2537 w2564 w2583 w2603 w2626 w2632 w2652 w2689 w2707 w2722 w2737 w2752 w2767 w2776 w2795 w2842 w2860 w2875 w2890 w2905 w2920 w2940 w2972 w2999 w3018 w3049 w3072 w3095 w3115 w3128 w3157 w3177 w3188 w3207 w3218 w3263 w3293 w3314 w3320 w3342 w3366 w3383 w3400 w3417 w3434 w3458 w3474 w3497 w3513 w3533 w3563 w3592]
            tunnel: w1684 -> [w1720 w1735 w1749 w1816 w1874 w1936 w1995 w2055 w2115 w2175 w2235 w2274 w2314 w2343 w2406 w2428 w2443 w2469 w2502 w2538 w2565 w2584 w2604 w2627 w2645 w2667 w2688 w2706 w2721 w2736 w2751 w2766 w2786 w2813 w2841 w2859 w2874 w2889 w2904 w2919 w2922 w2948 w2998 w3017 w3048 w3071 w3094 w3114 w3127 w3156 w3176 w3189 w3208 w3217 w3262 w3292 w3313 w3321 w3343 w3365 w3382 w3399 w3416 w3433 w3457 w3473 w3496 w3512 w3532 w3562 w3591]
            tunnel: w1683 -> [w1719 w1734 w1750 w1815 w1873 w1935 w1994 w2054 w2114 w2174 w2234 w2273 w2313 w2342 w2405 w2427 w2442 w2470 w2501 w2539 w2566 w2585 w2605 w2628 w2644 w2666 w2687 w2705 w2720 w2735 w2750 w2765 w2785 w2814 w2840 w2858 w2873 w2888 w2903 w2918 w2921 w2947 w2997 w3016 w3047 w3070 w3093 w3113 w3126 w3155 w3175 w3190 w3209 w3216 w3261 w3291 w3312 w3322 w3344 w3364 w3381 w3398 w3415 w3432 w3456 w3472 w3495 w3511 w3531 w3561 w3590]
            tunnel: [w1721 w1736 w1748 w1817 w1875 w1937 w1996 w2056 w2116 w2176 w2236 w2275 w2315 w2344 w2407 w2429 w2444 w2468 w2503 w2537 w2564 w2583 w2603 w2626 w2632 w2652 w2689 w2707 w2722 w2737 w2752 w2767 w2776 w2795 w2842 w2860 w2875 w2890 w2905 w2920 w2940 w2972 w2999 w3018 w3049 w3072 w3095 w3115 w3128 w3157 w3177 w3188 w3207 w3218 w3263 w3293 w3314 w3320 w3342 w3366 w3383 w3400 w3417 w3434 w3458 w3474 w3497 w3513 w3533 w3563 w3592] -> w1672
            tunnel: [w1720 w1735 w1749 w1816 w1874 w1936 w1995 w2055 w2115 w2175 w2235 w2274 w2314 w2343 w2406 w2428 w2443 w2469 w2502 w2538 w2565 w2584 w2604 w2627 w2645 w2667 w2688 w2706 w2721 w2736 w2751 w2766 w2786 w2813 w2841 w2859 w2874 w2889 w2904 w2919 w2922 w2948 w2998 w3017 w3048 w3071 w3094 w3114 w3127 w3156 w3176 w3189 w3208 w3217 w3262 w3292 w3313 w3321 w3343 w3365 w3382 w3399 w3416 w3433 w3457 w3473 w3496 w3512 w3532 w3562 w3591] -> w1671
            tunnel: [w1719 w1734 w1750 w1815 w1873 w1935 w1994 w2054 w2114 w2174 w2234 w2273 w2313 w2342 w2405 w2427 w2442 w2470 w2501 w2539 w2566 w2585 w2605 w2628 w2644 w2666 w2687 w2705 w2720 w2735 w2750 w2765 w2785 w2814 w2840 w2858 w2873 w2888 w2903 w2918 w2921 w2947 w2997 w3016 w3047 w3070 w3093 w3113 w3126 w3155 w3175 w3190 w3209 w3216 w3261 w3291 w3312 w3322 w3344 w3364 w3381 w3398 w3415 w3432 w3456 w3472 w3495 w3511 w3531 w3561 w3590] -> w1670
            tunnel: w1568 -> [w1717 w1732 w1747 w1781 w1857 w1876 w1938 w2052 w2112 w2172 w2232 w2271 w2311 w2339 w2358 w2420 w2436 w2466 w2473 w2513 w2553 w2574 w2593 w2616 w2633 w2655 w2680 w2703 w2717 w2733 w2748 w2763 w2775 w2797 w2835 w2857 w2871 w2886 w2901 w2916 w2934 w2961 w2974 w3014 w3024 w3069 w3085 w3111 w3125 w3146 w3174 w3187 w3200 w3221 w3238 w3269 w3309 w3324 w3345 w3360 w3377 w3394 w3411 w3422 w3448 w3463 w3483 w3507 w3523 w3542 w3571]
            tunnel: w1640 -> [w1716 w1731 w1746 w1812 w1870 w1931 w1990 w2050 w2110 w2170 w2230 w2269 w2309 w2332 w2350 w2417 w2441 w2465 w2471 w2508 w2556 w2567 w2597 w2620 w2643 w2664 w2679 w2701 w2719 w2732 w2747 w2762 w2771 w2811 w2833 w2852 w2872 w2885 w2900 w2915 w2924 w2949 w2995 w3001 w3041 w3065 w3086 w3109 w3124 w3148 w3171 w3186 w3206 w3210 w3237 w3284 w3308 w3325 w3346 w3359 w3376 w3393 w3410 w3423 w3452 w3468 w3479 w3506 w3527 w3557 w3586]
            tunnel: [w1717 w1732 w1747 w1781 w1857 w1876 w1938 w2052 w2112 w2172 w2232 w2271 w2311 w2339 w2357 w2419 w2436 w2459 w2472 w2512 w2553 w2573 w2592 w2615 w2630 w2654 w2681 w2702 w2717 w2733 w2748 w2763 w2774 w2791 w2834 w2855 w2871 w2886 w2901 w2916 w2933 w2960 w2996 w3013 w3042 w3068 w3087 w3110 w3125 w3149 w3173 w3187 w3199 w3220 w3238 w3267 w3309 w3324 w3345 w3360 w3377 w3394 w3411 w3422 w3448 w3463 w3483 w3507 w3523 w3542 w3571] -> w1581
            tunnel: [w1716 w1731 w1746 w1811 w1869 w1926 w1989 w2050 w2110 w2170 w2230 w2269 w2309 w2332 w2349 w2418 w2441 w2464 w2471 w2508 w2556 w2567 w2597 w2620 w2643 w2664 w2679 w2701 w2719 w2732 w2747 w2762 w2771 w2811 w2833 w2852 w2872 w2885 w2900 w2915 w2924 w2949 w2995 w3001 w3041 w3065 w3086 w3109 w3124 w3148 w3171 w3186 w3206 w3210 w3237 w3284 w3308 w3325 w3346 w3359 w3376 w3393 w3410 w3423 w3452 w3468 w3482 w3506 w3527 w3557 w3586] -> w1680
            tunnel: [_ _ _ _ _ _ _ _ _ _ _ _ _ _ _ _ _ _ _ _ _ _ _ _ _ _ _ _ _ _ _ _ _ _ _ _ _ _ _ _ _ _ _ w3007 _ _ _ _ _ _ _ _ _ _ _ _ _ _ _ _ _ _ _ _ _ _ _ _ _ _ _] -> w1598
            tunnel: [_ _ _ _ _ _ _ _ _ _ _ _ _ _ _ _ _ _ _ _ _ _ _ _ _ _ _ _ _ _ _ _ _ _ _ _ _ _ _ _ _ _ _ w3008 _ _ _ _ _ _ _ _ _ _ _ _ _ _ _ _ _ _ _ _ _ _ _ _ _ _ _] -> w1652
            tunnel: w1679 -> [w1714 w1729 w1744 w1783 w1859 w1932 w1991 w2051 w2111 w2171 w2231 w2270 w2310 w2337 w2401 w2409 w2438 w2449 w2494 w2535 w2562 w2570 w2589 w2612 w2642 w2663 w2676 w2697 w2718 w2730 w2745 w2760 w2784 w2810 w2832 w2850 w2868 w2883 w2898 w2913 w2946 w2970 w2992 w3015 w3026 w3062 w3083 w3107 w3122 w3147 w3170 w3184 w3202 w3225 w3259 w3280 w3306 w3327 w3348 w3357 w3374 w3391 w3408 w3428 w3442 w3465 w3489 w3504 w3525 w3555 w3584]
            tunnel: [w1714 w1729 w1744 w1783 w1859 w1932 w1991 w2051 w2111 w2171 w2231 w2270 w2310 w2337 w2401 w2408 w2435 w2449 w2494 w2535 w2562 w2570 w2589 w2612 w2642 w2663 w2676 w2697 w2718 w2730 w2745 w2760 w2784 w2810 w2832 w2850 w2868 w2883 w2898 w2913 w2946 w2970 w2992 w3015 w3025 w3062 w3083 w3107 w3122 w3147 w3170 w3184 w3201 w3225 w3259 w3280 w3306 w3327 w3348 w3357 w3374 w3391 w3408 w3428 w3442 w3465 w3489 w3504 w3525 w3555 w3584] -> w1678
            tunnel: w1677 -> [w1715 w1730 w1745 w1782 w1858 w1933 w1992 w2048 w2108 w2168 w2228 w2267 w2307 w2338 w2402 w2430 w2440 w2463 w2483 w2536 w2563 w2576 w2595 w2618 w2640 w2651 w2677 w2698 w2715 w2731 w2746 w2761 w2783 w2799 w2831 w2851 w2869 w2884 w2899 w2914 w2945 w2971 w2993 w3010 w3039 w3063 w3082 w3108 w3123 w3144 w3169 w3185 w3205 w3224 w3260 w3283 w3307 w3326 w3347 w3358 w3375 w3392 w3409 w3429 w3451 w3467 w3491 w3502 w3526 w3556 w3585]
            tunnel: [w1715 w1730 w1745 w1782 w1858 w1933 w1992 w2049 w2109 w2169 w2229 w2268 w2308 w2338 w2402 w2430 w2440 w2463 w2483 w2536 w2563 w2576 w2595 w2618 w2640 w2651 w2677 w2698 w2715 w2731 w2746 w2761 w2783 w2799 w2831 w2851 w2869 w2884 w2899 w2914 w2945 w2971 w2993 w3010 w3039 w3063 w3082 w3108 w3123 w3144 w3169 w3185 w3205 w3224 w3260 w3283 w3307 w3326 w3347 w3358 w3375 w3392 w3409 w3429 w3451 w3467 w3491 w3502 w3526 w3556 w3585] -> w1676
            tunnel: [_ _ _ _ _ _ _ _ _ _ _ _ _ _ _ _ _ _ _ _ _ _ _ _ _ _ _ _ _ _ _ _ _ _ _ _ _ _ _ _ _ _ _ _ _ _ _ _ _ _ _ _ _ _ _ _ TRUE _ _ _ _ _ _ _ _ _ _ _ _ _ _] -> w1673
            tunnel: w1664 -> [_ _ _ _ _ _ _ _ _ _ _ _ _ _ _ _ _ _ _ _ _ _ _ _ _ _ _ _ _ _ _ _ _ w2809 _ _ _ _ _ _ _ _ _ _ _ _ _ _ _ _ _ _ _ _ _ _ _ _ _ _ _ _ _ _ _ _ _ _ _ _ _]
            tunnel: w1663 -> [_ _ _ _ _ _ _ _ _ _ _ _ _ _ _ _ _ _ _ _ _ _ _ _ _ _ _ _ _ _ _ _ _ w2808 _ _ _ _ _ _ _ _ _ _ _ _ _ _ _ _ _ _ _ _ _ _ _ _ _ _ _ _ _ _ _ _ _ _ _ _ _]
            tunnel: [_ _ _ _ _ _ _ _ _ _ _ _ _ _ _ _ _ _ _ _ _ _ _ _ _ _ _ _ _ _ _ _ w2770 w2809 _ _ _ _ _ _ _ _ _ _ _ _ _ _ _ _ _ _ _ _ _ _ _ _ _ _ _ _ _ _ _ _ _ _ _ _ _] -> w1639
            tunnel: [_ _ _ _ _ _ _ _ _ _ _ _ _ _ _ _ _ _ _ _ _ _ _ _ _ _ _ _ _ _ _ _ w2769 w2808 _ _ _ _ _ _ _ _ _ _ _ _ _ _ _ _ _ _ _ _ _ _ _ _ _ _ _ _ _ _ _ _ _ _ _ _ _] -> w1638
            tunnel: w1648 -> [w1712 w1727 w1742 w1773 w1855 w1921 w1988 w2035 w2100 w2155 w2215 w2242 w2292 w2331 w2400 w2426 w2439 w2462 w2486 w2528 w2552 w2572 w2591 w2614 w2639 w2662 w2674 w2696 w2713 w2728 w2743 w2758 w2782 w2807 w2829 w2849 w2866 w2881 w2896 w2911 w2944 w2969 w2982 w3000 w3037 w3061 w3078 w3101 w3121 w3140 w3163 w3183 w3198 w3223 w3252 w3279 w3304 w3328 w3349 w3356 w3373 w3390 w3407 w3427 w3450 w3466 w3490 w3505 w3520 w3554 w3583]
            tunnel: [w1712 w1727 w1742 w1773 w1855 w1921 w1988 w2035 w2100 w2155 w2215 w2242 w2292 w2331 w2400 w2426 w2439 w2462 w2485 w2527 w2545 w2571 w2590 w2613 w2639 w2662 w2674 w2696 w2713 w2728 w2743 w2758 w2782 w2807 w2829 w2849 w2866 w2881 w2896 w2911 w2944 w2969 w2982 w3000 w3037 w3061 w3078 w3101 w3121 w3140 w3163 w3183 w3198 w3222 w3252 w3279 w3304 w3328 w3349 w3356 w3373 w3390 w3407 w3427 w3450 w3466 w3490 w3505 w3520 w3554 w3583] -> w1647
            tunnel: [w1711 w1726 w1741 w1772 w1854 w1920 w1987 w2034 w2099 w2154 w2214 w2241 w2291 w2330 w2399 w2425 w2446 w2461 w2496 w2534 w2561 w2582 w2602 w2625 w2638 w2661 w2673 w2695 w2712 w2727 w2742 w2757 w2781 w2806 w2828 w2848 w2865 w2880 w2895 w2910 w2943 w2968 w2981 w3006 w3036 w3060 w3077 w3100 w3120 w3139 w3162 w3182 w3197 w3215 w3258 w3278 w3302 w3329 w3339 w3355 w3372 w3389 w3406 w3426 w3454 w3470 w3493 w3509 w3529 w3559 w3588] -> w1646
            tunnel: [w1710 w1725 w1740 w1771 w1853 w1919 w1986 w2033 w2098 w2153 w2213 w2240 w2290 w2329 w2398 w2424 w2445 w2460 w2495 w2533 w2560 w2581 w2601 w2624 w2637 w2660 w2672 w2694 w2711 w2726 w2741 w2756 w2780 w2805 w2827 w2847 w2864 w2879 w2894 w2909 w2942 w2967 w2980 w3005 w3035 w3059 w3076 w3099 w3119 w3138 w3161 w3181 w3196 w3214 w3257 w3277 w3303 w3315 w3336 w3361 w3378 w3395 w3412 w3430 w3453 w3469 w3492 w3508 w3528 w3558 w3587] -> w1645
            tunnel: w1644 -> [w1711 w1726 w1741 w1772 w1854 w1920 w1987 w2034 w2099 w2154 w2214 w2241 w2291 w2330 w2399 w2425 w2446 w2461 w2496 w2534 w2561 w2582 w2602 w2625 w2638 w2661 w2673 w2695 w2712 w2727 w2742 w2757 w2781 w2806 w2828 w2848 w2865 w2880 w2895 w2910 w2943 w2968 w2981 w3006 w3036 w3060 w3077 w3100 w3120 w3139 w3162 w3182 w3197 w3215 w3258 w3278 w3302 _ w3339 w3355 w3372 w3389 w3406 w3426 w3454 w3470 w3493 w3509 w3529 w3559 w3588]
            tunnel: w1643 -> [w1710 w1725 w1740 w1771 w1853 w1919 w1986 w2033 w2098 w2153 w2213 w2240 w2290 w2329 w2398 w2424 w2445 w2460 w2495 w2533 w2560 w2581 w2601 w2624 w2637 w2660 w2672 w2694 w2711 w2726 w2741 w2756 w2780 w2805 w2827 w2847 w2864 w2879 w2894 w2909 w2942 w2967 w2980 w3005 w3035 w3059 w3076 w3099 w3119 w3138 w3161 w3181 w3196 w3214 w3257 w3277 w3303 _ w3336 w3361 w3378 w3395 w3412 w3430 w3453 w3469 w3492 w3508 w3528 w3558 w3587]
            tunnel: w1642 -> [_ _ _ _ _ _ _ _ _ _ _ _ _ _ _ _ _ _ _ _ _ _ _ _ _ _ _ _ _ _ _ _ _ _ _ _ _ _ _ _ _ _ _ _ _ _ _ _ _ _ _ _ _ _ _ _ _ _ _ w3353 w3370 w3387 w3404 w3424 _ _ _ _ _ _ _]
            tunnel: w1641 -> [_ _ _ _ _ _ _ _ _ _ _ _ _ _ _ _ _ _ _ _ _ _ _ _ _ _ _ _ _ _ _ _ _ _ _ _ _ _ _ _ _ _ _ _ _ _ _ _ _ _ _ _ _ _ _ _ _ _ _ _ _ _ _ _ _ _ w3484 _ _ _ _]
            tunnel: [w1709 w1724 w1739 w1770 w1852 w1918 w1985 w2032 w2097 w2152 w2212 w2239 w2289 w2328 w2397 w2415 w2433 w2458 w2497 w2532 w2559 w2580 w2600 w2623 w2636 w2659 w2671 w2693 w2710 w2725 w2740 w2755 w2779 w2804 w2826 w2846 w2863 w2878 w2893 w2908 w2939 w2966 w2979 w3004 w3020 w3058 w3075 w3098 w3118 w3137 w3160 w3180 w3195 w3213 w3255 w3264 w3301 w3318 w3338 w3352 w3369 w3386 w3403 w3421 w3437 w3462 w3478 w3501 w3518 w3553 w3582] -> w1636
            tunnel: w1637 -> [w1709 w1724 w1739 w1770 w1852 w1918 w1985 w2032 w2097 w2152 w2212 w2239 w2289 w2328 w2397 _ _ w2458 w2497 w2532 w2559 w2580 w2600 w2623 w2636 w2659 w2671 w2693 w2710 w2725 w2740 w2755 w2779 w2804 w2826 w2846 w2863 w2878 w2893 w2908 w2939 w2966 w2979 w3004 w3020 w3058 w3075 w3098 w3118 w3137 w3160 w3180 w3195 w3213 w3255 w3265 w3301 w3318 w3338 w3352 w3369 w3386 w3403 w3421 w3437 w3462 w3478 w3501 w3518 w3553 w3582]
            tunnel: w1635 -> [w1708 w1723 w1738 w1769 w1851 w1917 w1984 w2031 w2096 w2151 w2211 w2238 w2288 w2327 w2396 w2423 w2432 w2457 w2493 w2531 w2558 w2579 w2599 w2622 w2635 w2658 w2670 w2692 w2709 w2724 w2739 w2754 w2778 w2803 w2825 w2845 w2862 w2877 w2892 w2907 w2938 w2965 w2978 w3003 w3034 w3057 w3074 w3097 w3117 w3136 w3159 w3179 w3194 w3212 w3254 w3276 w3300 w3317 w3341 w3351 w3368 w3385 w3402 w3420 w3436 w3461 w3477 w3500 w3517 w3552 w3581]
            tunnel: w1634 -> [w1707 w1722 w1737 w1768 w1850 w1916 w1983 w2030 w2095 w2150 w2210 w2237 w2287 w2326 w2395 w2422 w2431 w2456 w2492 w2530 w2557 w2578 w2598 w2621 w2634 w2657 w2669 w2691 w2708 w2723 w2738 w2753 w2777 w2802 w2824 w2844 w2861 w2876 w2891 w2906 w2937 w2964 w2977 w3002 w3031 w3056 w3073 w3096 w3116 w3135 w3158 w3178 w3193 w3211 w3253 w3275 w3299 w3316 w3340 w3350 w3367 w3384 w3401 w3419 w3435 w3460 w3476 w3499 w3516 w3551 w3580]
            tunnel: [w1708 w1723 w1738 w1769 w1851 w1917 w1984 w2031 w2096 w2151 w2211 w2238 w2288 w2327 w2396 w2423 w2432 w2457 w2493 w2531 w2558 w2579 w2599 w2622 w2635 w2658 w2670 w2692 w2709 w2724 w2739 w2754 w2778 w2803 w2825 w2845 w2862 w2877 w2892 w2907 w2938 w2965 w2978 w3003 w3033 w3057 w3074 w3097 w3117 w3136 w3159 w3179 w3194 w3212 w3254 w3276 w3300 w3317 w3341 w3351 w3368 w3385 w3402 w3420 w3436 w3461 w3477 w3500 w3517 w3552 w3581] -> w1633
            tunnel: [w1707 w1722 w1737 w1768 w1850 w1916 w1983 w2030 w2095 w2150 w2210 w2237 w2287 w2326 w2395 w2422 w2431 w2456 w2492 w2530 w2557 w2578 w2598 w2621 w2634 w2657 w2669 w2691 w2708 w2723 w2738 w2753 w2777 w2802 w2824 w2844 w2861 w2876 w2891 w2906 w2937 w2964 w2977 w3002 w3032 w3056 w3073 w3096 w3116 w3135 w3158 w3178 w3193 w3211 w3253 w3275 w3299 w3316 w3340 w3350 w3367 w3384 w3401 w3419 w3435 w3460 w3476 w3499 w3516 w3551 w3580] -> w1632
            tunnel: w1631 -> [w1706 _ _ _ _ _ _ _ _ _ _ _ _ w2323 w2392 _ _ w2453 w2500 w2522 w2543 _ _ w2608 _ _ _ _ _ _ _ _ _ w2801 _ _ _ _ _ _ w2935 w2963 _ _ _ _ _ _ _ w3134 _ _ _ _ w3234 _ w3297 _ _ _ _ _ _ _ _ _ _ _ _ _ _]
            tunnel: w1630 -> [w1705 _ _ _ _ _ _ _ _ _ _ _ _ w2322 w2393 _ _ w2452 w2499 w2521 w2542 _ _ w2607 _ _ _ _ _ _ _ _ _ w2800 _ _ _ _ _ _ w2936 w2962 _ _ _ _ _ _ _ w3133 _ _ _ _ w3233 _ w3296 _ _ _ _ _ _ _ _ _ _ _ _ _ _]
            tunnel: [_ _ _ _ _ _ _ _ _ _ _ _ _ _ _ _ _ _ _ _ _ _ _ _ _ w2649 _ _ _ _ _ _ _ w2787 _ _ _ _ _ _ w2928 w2954 _ _ _ _ _ _ _ _ _ _ _ _ _ _ _ _ _ _ _ _ _ _ _ _ _ _ _ _ _] -> w1589
            tunnel: [_ _ _ _ _ _ _ _ _ _ _ _ _ _ _ _ _ _ _ _ _ _ _ _ _ w2648 _ _ _ _ _ _ _ w2788 _ _ _ _ _ _ w2927 w2953 _ _ _ _ _ _ _ _ _ _ _ _ _ _ _ _ _ _ _ _ _ _ _ _ _ _ _ _ _] -> w1588
            tunnel: [_ _ _ _ _ _ _ _ _ _ _ _ _ _ _ _ _ _ _ _ _ _ TRUE ("Recording") _ _ _ _ _ _ _ _ _ _ _ _ _ _ _ _ _ _ _ _ _ _ _ _ _ _ _ _ _ _ _ _ _ _ _ _ _ _ _ _ _ _ _ _ _ _ _ _] -> w1625
            tunnel: [_ _ _ _ _ _ _ _ _ _ _ _ _ _ _ TRUE _ _ _ _ _ _ _ _ _ _ _ _ _ _ _ _ _ _ _ _ _ _ _ _ _ _ _ _ _ _ _ _ _ _ _ _ _ _ _ _ _ _ _ _ _ _ _ _ _ _ _ _ _ _ _] -> w1622
            tunnel: [_ _ _ _ _ _ _ _ _ _ _ _ _ _ _ _ _ TRUE _ _ _ _ _ _ _ _ _ _ _ _ _ _ _ _ _ _ _ _ _ _ _ _ _ _ _ _ _ _ _ _ _ _ _ _ _ _ _ _ _ _ _ _ _ _ _ _ _ _ _ _ _] -> w1620
            tunnel: [_ _ _ _ _ _ _ _ _ _ _ _ _ _ _ _ _ w2448 _ _ _ _ _ _ _ _ _ _ _ _ _ _ _ _ _ _ _ _ _ _ _ _ _ _ _ _ _ _ _ _ _ _ _ _ _ _ _ _ _ _ _ _ _ _ _ _ _ _ _ _ _] -> w1619
            tunnel: w1606 -> [_ _ _ _ _ _ _ _ _ _ _ _ _ _ _ _ _ _ _ _ _ _ _ _ _ _ _ _ _ _ _ _ _ _ _ _ _ _ _ _ _ _ _ _ _ _ _ _ _ _ _ _ _ _ _ _ _ _ _ _ _ _ _ _ _ _ _ _ _ w3549 w3578]
            tunnel: [_ _ _ _ _ _ _ _ _ _ _ _ _ _ _ _ _ _ _ _ _ _ _ _ _ _ _ _ _ _ _ _ _ _ _ _ _ _ _ _ _ _ _ _ _ _ _ _ _ _ _ _ _ _ _ _ _ _ _ _ _ _ _ _ _ _ _ _ _ w3547 w3576] -> w1605
            tunnel: w1601 -> [_ _ _ _ _ _ _ _ _ _ _ _ _ _ _ _ _ _ _ _ w2544 w2569 w2588 w2611 w2629 w2650 w2668 w2690 _ _ _ _ w2768 w2798 w2823 w2843 _ _ _ _ w2929 w2955 _ _ _ _ _ _ _ _ _ _ _ _ _ _ _ _ _ _ _ _ _ _ _ _ _ _ _ _ _]
            tunnel: [_ _ _ _ _ _ _ _ _ _ _ _ _ _ _ _ _ _ _ w2510 w2544 w2568 w2587 w2610 w2629 w2650 w2668 w2690 _ _ _ _ w2768 w2798 w2823 w2843 _ _ _ _ w2929 w2955 _ _ _ _ _ _ _ _ _ _ _ _ _ _ _ _ _ _ _ _ _ _ _ _ _ _ _ _ _] -> w1600
            tunnel: [_ _ _ _ _ _ _ _ _ _ _ _ _ _ _ _ _ _ _ _ _ _ _ _ _ w2647 _ _ _ _ _ _ _ w2792 _ _ _ _ _ _ w2926 w2952 _ _ _ _ _ _ _ _ _ _ _ _ _ _ _ _ _ _ _ _ _ _ _ _ _ _ _ _ _] -> w1593
            tunnel: [_ _ _ _ _ _ _ _ _ _ _ _ _ _ _ _ _ _ _ _ _ _ _ _ _ w2646 _ _ _ _ _ _ _ w2793 _ _ _ _ _ _ w2925 w2951 _ _ _ _ _ _ _ _ _ _ _ _ _ _ _ _ _ _ _ _ _ _ _ _ _ _ _ _ _] -> w1591
            tunnel: [_ _ _ _ _ _ _ _ _ _ _ _ _ _ _ _ _ _ _ _ _ _ _ _ _ _ _ _ _ _ _ _ _ w2794 _ _ _ _ _ _ _ _ _ _ _ _ _ _ _ _ _ _ _ _ _ _ _ _ _ _ _ _ _ _ _ _ _ _ _ _ _] -> w1597
            tunnel: [_ _ _ _ _ _ _ _ _ _ _ _ _ _ _ w2410 _ _ _ _ _ _ _ _ _ _ _ _ _ _ _ _ _ _ _ _ _ _ _ _ _ _ _ _ _ _ _ _ _ _ _ _ _ _ _ _ _ _ _ _ _ _ _ _ _ _ _ _ _ _ _] -> w1580
            frame "Start1", Default {
              w1704 = FALSE ("SelectionState")
              n995 = local read "CueLed_baseline"() -> (w1703:bool)
              n996 = xnode "Read/Write Control"("FPGA VI Reference In"=w1706, "error in"=w1705, "SelectionState"=w1704, "LR_reward_Laser_l1"=w1704, "LR_wrong_Laser_l1"=w1704, "LR_reward_Event_l1"=w1704, "LR_wrong_Event_l1"=w1704, "Left(F)_or_Right(T)"=w1704, "ignoreWrong"=w1704, "SelectionState"=w1704, "LR_reward_Laser_l2"=w1704, "LR_wrong_laser_l2"=w1704, "LR_reward_Event_l2"=w1704, "LR_wrong_Event_l2"=w1704, "LC_Event_l1"=w1704, "LC_Laser_l1"=w1704, "LC_Laser_l2"=w1704, "LC_Event_l2"=w1704, "CueLed_Event"=w1704, "I_allReward"=w1704, "CueLed_Baseline"=w1703) -> ()  [unwired: 2 out]
            }
            frame "Start2" {
            }
            frame "Start3" {
            }
            frame "saveSettings1" {
              n997 = call "myRIO_BRig_RT_dataExp_Tcycle_Reward_min_L.vi"() -> ("output_Tcycle_Reward_min_L"=w1757:i32)  [unwired: 11 in]
              n998 = local read "Tcycle_Reward_min_L"() -> (w1756:u16)
              n999 = call "myRIO_BRig_RT_dataExp_Audio_freq__L.vi"() -> ("output_Audio_freq__L"=w1789:i32)  [unwired: 11 in]
              n1000 = call "myRIO_BRig_RT_dataExp_Audio_freq__R.vi"() -> ("output_Audio_freq__R"=w1788:i32)  [unwired: 11 in]
              n1001 = call "myRIO_BRig_RT_dataExp_Audio_amp__L.vi"() -> ("output_Audio_amp__L"=w1787:i32)  [unwired: 11 in]
              n1002 = call "myRIO_BRig_RT_dataExp_Audio_amp__R.vi"() -> ("output_Audio_amp__R"=w1785:i32)  [unwired: 11 in]
              n1003 = call "myRIO_BRig_RT_dataExp_TPB_min__L.vi"() -> ("output_TPB_min__L"=w1797:i32)  [unwired: 11 in]
              n1004 = call "myRIO_BRig_RT_dataExp_TPB_min__R.vi"() -> ("output_TPB_min__R"=w1795:i32)  [unwired: 11 in]
              n1005 = call "myRIO_BRig_RT_dataExp_TPB_max__L.vi"() -> ("output_TPB_max__L"=w1793:i32)  [unwired: 11 in]
              n1006 = call "myRIO_BRig_RT_dataExp_TPB_max__R.vi"() -> ("output_TPB_max__R"=w1791:i32)  [unwired: 11 in]
              n1007 = call "myRIO_BRig_RT_dataExp_Cue1Param_AudioLed_Count_Switch.vi"() -> ("output_Cue1Param_AudioLed_Count_Switch"=w1763:i32)  [unwired: 11 in]
              n1008 = call "myRIO_BRig_RT_dataExp_Cue1Param_AudioLed_Probability_Switch.vi"() -> ("output_Cue1Param_AudioLed_Probability_Switch"=w1761:i32)  [unwired: 11 in]
              n1009 = call "myRIO_BRig_RT_dataExp_Cue1Param_CueType_Switch.vi"() -> ("output_Cue1Param_CueType_Switch"=w1759:i32)  [unwired: 11 in]
              n1010 = call "myRIO_BRig_RT_dataExp_ItrialUntilReward.vi"() -> ("output_I_trialUntilReward"=w1810:i32)  [unwired: 11 in]
              n1011 = call "myRIO_BRig_RT_dataExp_IblockUntilReward.vi"() -> ("output_I_blockUntilReward"=w1806:i32)  [unwired: 11 in]
              n1012 = call "myRIO_BRig_RT_dataExp_CueCycles.vi"() -> ("output_CueCycles"=w1805:i32)  [unwired: 11 in]
              n1013 = call "myRIO_BRig_RT_dataExp_ENL_min.vi"() -> ("output_ENL_min"=w1803:i32)  [unwired: 11 in]
              n1014 = call "myRIO_BRig_RT_dataExp_ENL_max.vi"() -> ("output_ENL_max"=w1801:i32)  [unwired: 11 in]
              n1015 = call "myRIO_BRig_RT_dataExp_ENL_penalty.vi"() -> ("output_ENL_penalty"=w1799:i32)  [unwired: 11 in]
              n1016 = local read "Audio_Freq__L"() -> (w1767:u8)
              n1017 = local read "Audio_Freq__R"() -> (w1765:u8)
              n1018 = local read "Audio_Amp__L"() -> (w1786:u16)
              n1019 = local read "TpB_Min_L"() -> (w1796:u16)
              n1020 = local read "TpB_Min_R"() -> (w1794:u16)
              n1021 = local read "TpB_Max_L"() -> (w1792:u16)
              n1022 = local read "TpB_Max_R"() -> (w1790:u16)
              n1023 = local read "Audio_Amp__R"() -> (w1784:u16)
              n1024 = local read "TrialUntilReward"() -> (w1809:bool)
              n1025 = local read "CueCycles"() -> (w1804:u16)
              n1026 = local read "Tcycle_ENL_min"() -> (w1802:u16)
              n1027 = local read "Tcycle_ENL_max"() -> (w1800:u16)
              n1028 = local read "Tcycle_ENLPenalty"() -> (w1798:u16)
              n1029 = local read "Cue1Param_AudioLed_Count_Switch"() -> (w1762:u16)
              n1030 = local read "Cue1Param_AudioLed_Probability_Switch"() -> (w1760:u16)
              n1031 = local read "Cue1Param_CueType_Switch"() -> (w1758:u16)
              n1032 = local read "Tcycle_Reward_max_L"() -> (w1754:u16)
              n1033 = call "myRIO_BRig_RT_dataExp_Tcycle_Reward_max_L.vi"() -> ("output_Tcycle_Reward_max_L"=w1755:i32)  [unwired: 11 in]
              n1034 = To Unsigned Word Integer(number=w1765) -> (unsigned 16bit integer=w1764:u16)
              n1035 = To Unsigned Word Integer(number=w1767) -> (unsigned 16bit integer=w1766:u16)
              n1036 = Boolean To (0,1)(Boolean=w1809) -> (0, 1=w1808:i16)
              n1037 = To Unsigned Word Integer(number=w1808) -> (unsigned 16bit integer=w1807:u16)
              n1038 = call "myRIO_BRig_RT_dataExp_Tcycle_Reward_step_L.vi"() -> ("output_Tcycle_Reward_step_L"=w1753:i32)  [unwired: 11 in]
              n1039 = local read "Tcycle_Reward_step_L"() -> (w1752:u16)
              n1040 = local read "BUR_min"() -> (w1778:u16)
              n1041 = local read "BUR_max"() -> (w1779:u16)
              n1042 = Not Equal To 0?(x=w1778) -> (x != 0?=w1777:bool)
              n1043 = Not Equal To 0?(x=w1779) -> (x != 0?=w1776:bool)
              n1044 = And(x=w1777, y=w1776) -> (x .and. y?=w1775:bool)
              n1045 = Boolean To (0,1)(Boolean=w1775) -> (0, 1=w1780:i16)
              n1046 = To Unsigned Word Integer(number=w1780) -> (unsigned 16bit integer=w1774:u16)
              n1047 = Replace Array Subset(array=w1812, new element #1=w1807, index #1=w1810, new element #2=w1774, index #2=w1806, new element #3=w1804, index #3=w1805, new element #4=w1802, index #4=w1803, new element #5=w1800, index #5=w1801, new element #6=w1798, index #6=w1799, new element #7=w1796, index #7=w1797, new element #8=w1794, index #8=w1795, new element #9=w1792, index #9=w1793, new element #10=w1790, index #10=w1791, new element #11=w1766, index #11=w1789, new element #12=w1764, index #12=w1788, new element #13=w1786, index #13=w1787, new element #14=w1784, index #14=w1785, new element #15=w1762, index #15=w1763, new element #16=w1760, index #16=w1761, new element #17=w1758, index #17=w1759, new element #18=w1756, index #18=w1757, new element #19=w1754, index #19=w1755, new element #20=w1752, index #20=w1753) -> (w1811:u16[])
            }
            frame "saveSettings2" {
              n1048 = call "myRIO_BRig_RT_dataExp_Tcycle_Reward_min_R.vi"() -> ("output_Tcycle_Reward_min_R"=w1831:i32)  [unwired: 11 in]
              n1049 = local read "Tcycle_Reward_min_R"() -> (w1830:u16)
              n1050 = call "myRIO_BRig_RT_dataExp_Tcycle_Cue1_Audio_min.vi"() -> ("output_Tcycle_Cue1_Audio_min"=w1862:i32)  [unwired: 11 in]
              n1051 = call "myRIO_BRig_RT_dataExp_Tcycle_Cue1_Audio_max.vi"() -> ("output_Tcycle_Cue1_Audio_max"=w1861:i32)  [unwired: 11 in]
              n1052 = call "myRIO_BRig_RT_dataExp_Tcycle_Cue1Penalty_Audio.vi"() -> ("output_Tcycle_Cue1Penalty_Audio"=w1860:i32)  [unwired: 11 in]
              n1053 = call "myRIO_BRig_RT_dataExp_Tcycle_RewardPost.vi"() -> ("output_Tcycle_RewardPost"=w1868:i32)  [unwired: 11 in]
              n1054 = call "myRIO_BRig_RT_dataExp_Tcycle_Wrong.vi"() -> ("output_Tcycle_Wrong"=w1866:i32)  [unwired: 11 in]
              n1055 = call "myRIO_BRig_RT_dataExp_Tcycle_Timeout.vi"() -> ("output_Tcycle_Timeout"=w1864:i32)  [unwired: 11 in]
              n1056 = call "myRIO_BRig_RT_dataExp_Tcycle_Cue1_LED_min.vi"() -> ("output_Tcycle_Cue1_LED_min"=w1837:i32)  [unwired: 11 in]
              n1057 = call "myRIO_BRig_RT_dataExp_Tcycle_Cue1_LED_max.vi"() -> ("output_Tcycle_Cue1_LED_max"=w1836:i32)  [unwired: 11 in]
              n1058 = call "myRIO_BRig_RT_dataExp_Tcycle_Cue1Penalty_LED.vi"() -> ("output_Tcycle_Cue1Penalty_LED"=w1835:i32)  [unwired: 11 in]
              n1059 = call "myRIO_BRig_RT_dataExp_SolenoidProbability_L.vi"() -> ("output_SolenoidProbability_L"=w1847:i32)  [unwired: 11 in]
              n1060 = call "myRIO_BRig_RT_dataExp_SolenoidProbability_R.vi"() -> ("output_SolenoidProbability_R"=w1846:i32)  [unwired: 11 in]
              n1061 = call "myRIO_BRig_RT_dataExp_Cue1Param_AudioLed_Count_NS.vi"() -> ("output_Cue1Param_AudioLed_Count_NS"=w1843:i32)  [unwired: 11 in]
              n1062 = call "myRIO_BRig_RT_dataExp_Cue1Param_AudioLed_Probability_NS.vi"() -> ("output_Cue1Param_AudioLed_Probability_NS"=w1841:i32)  [unwired: 11 in]
              n1063 = call "myRIO_BRig_RT_dataExp_Cue1Param_CueType_NS.vi"() -> ("output_Cue1Param_CueType_NS"=w1839:i32)  [unwired: 11 in]
              n1064 = call "myRIO_BRig_RT_dataExp_nBlock.vi"() -> ("output_nBlock"=w1818:i32)  [unwired: 11 in]
              n1065 = call "myRIO_BRig_RT_dataExp_nTrial.vi"() -> ("output_nTrial"=w1820:i32)  [unwired: 11 in]
              n1066 = call "myRIO_BRig_RT_dataExp_runTime_seconds.vi"() -> ("output_RunTime_minutes"=w1823:i32)  [unwired: 11 in]
              n1067 = call "myRIO_BRig_RT_dataExp_Tcycle_Selection.vi"() -> ("output_Tcycle_Selection"=w1825:i32)  [unwired: 11 in]
              n1068 = local read "Tcycle_CuePenalty_Audio"() -> (w1856:u16)
              n1069 = local read "Tcycle_Cue_Audio_max"() -> (w1848:u16)
              n1070 = local read "Tcycle_Cue_Audio_min"() -> (w1849:u16)
              n1071 = local read "Tcycle_RewardPost"() -> (w1867:u16)
              n1072 = local read "Tcycle_Wrong"() -> (w1865:u16)
              n1073 = local read "Tcycle_Timeout"() -> (w1863:u16)
              n1074 = local read "Tcycle_Selection"() -> (w1824:u16)
              n1075 = local read "Cue1Param_AudioLed_Count_NS"() -> (w1842:u16)
              n1076 = local read "Cue1Param_AudioLed_Probability_NS"() -> (w1840:u16)
              n1077 = local read "Cue1Param_CueType_NS"() -> (w1838:u16)
              n1078 = local read "Tcycle_CuePenalty_LED"() -> (w1832:u16)
              n1079 = local read "SolenoidProbability_R"() -> (w1844:u16)
              n1080 = local read "SolenoidProbability_L"() -> (w1845:u16)
              n1081 = local read "Tcycle_Cue_LED_min"() -> (w1834:u16)
              n1082 = local read "Tcycle_Cue_LED_max"() -> (w1833:u16)
              n1083 = local read "Tcycle_Reward_max_R"() -> (w1828:u16)
              n1084 = call "myRIO_BRig_RT_dataExp_Tcycle_Reward_max_R.vi"() -> ("output_Tcycle_Reward_max_R"=w1829:i32)  [unwired: 11 in]
              n1085 = call "myRIO_BRig_RT_dataExp_Tcycle_Reward_step_R.vi"() -> ("output_Tcycle_Reward_step_R"=w1827:i32)  [unwired: 11 in]
              n1086 = local read "Tcycle_Reward_step_R"() -> (w1826:u16)
              n1087 = Replace Array Subset(array=w1870, new element #1=u16 0, index #1=w1818, new element #2=u16 0, index #2=w1820, new element #3=u16 0, index #3=w1823, new element #4=w1824, index #4=w1825, new element #5=w1867, index #5=w1868, new element #6=w1865, index #6=w1866, new element #7=w1863, index #7=w1864, new element #8=w1849, index #8=w1862, new element #9=w1848, index #9=w1861, new element #10=w1856, index #10=w1860, new element #11=w1845, index #11=w1847, new element #12=w1844, index #12=w1846, new element #13=w1842, index #13=w1843, new element #14=w1840, index #14=w1841, new element #15=w1838, index #15=w1839, new element #16=w1834, index #16=w1837, new element #17=w1833, index #17=w1836, new element #18=w1832, index #18=w1835, new element #19=w1830, index #19=w1831, new element #20=w1828, index #20=w1829, new element #21=w1826, index #21=w1827) -> (w1869:u16[])
            }
            frame "saveSettings3" {
              w1882 = 100.0 ("y")
              n1088 = call "myRIO_BRig_RT_dataExp_laser1_Freq.vi"() -> ("output_laser1_Freq"=w1915:i32)  [unwired: 11 in]
              n1089 = call "myRIO_BRig_RT_dataExp_laser1_Tpeak.vi"() -> ("output_laser1_Tpeak"=w1910:i32)  [unwired: 11 in]
              n1090 = call "myRIO_BRig_RT_dataExp_laser1_Tshutter.vi"() -> ("output_laser1_Tshutter"=w1905:i32)  [unwired: 11 in]
              n1091 = call "myRIO_BRig_RT_dataExp_FPGA_f_count2ms.vi"() -> ("output_FPGA_f_count2ms"=w1900:i32)  [unwired: 11 in]
              n1092 = call "myRIO_BRig_RT_dataExp_laser1_Power_min.vi"() -> ("output_laser1_Power_min"=w1895:i32)  [unwired: 11 in]
              n1093 = call "myRIO_BRig_RT_dataExp_laser1_Power_max.vi"() -> ("output_laser1_Power_max"=w1888:i32)  [unwired: 11 in]
              n1094 = call "myRIO_BRig_RT_dataExp_laser1_Power_step.vi"() -> ("output_laser1_Power_step"=w1887:i32)  [unwired: 11 in]
              n1095 = call "myRIO_BRig_RT_dataExp_laser1_duration.vi"() -> ("output_laser1_duration"=w1890:i32)  [unwired: 11 in]
              n1096 = local read "Laser_Tshutter_l1"() -> (w1902:dbl)
              n1097 = local read "Laser_Tpeak_l1"() -> (w1907:dbl)
              n1098 = local read "Laser_power_max_l1"() -> (w1881:dbl)
              n1099 = local read "Laser_power_step_l1"() -> (w1880:dbl)
              n1100 = local read "Laser_power_min_l1"() -> (w1892:dbl)
              n1101 = local read "Laser_Freq_l1"() -> (w1914:dbl)
              n1102 = call "myRIO_BRig_RT_dataExp_BUR_min.vi"() -> ("output_BUR_min"=w1930:i32)  [unwired: 11 in]
              n1103 = call "myRIO_BRig_RT_dataExp_BUR_max.vi"() -> ("output_BUR_max"=w1928:i32)  [unwired: 11 in]
              n1104 = call "myRIO_BRig_RT_dataExp_Audio_sp__L.vi"() -> ("output_Audio_sp__L"=w1925:i32)  [unwired: 11 in]
              n1105 = call "myRIO_BRig_RT_dataExp_Audio_sp__R.vi"() -> ("output_Audio_sp__R"=w1924:i32)  [unwired: 11 in]
              n1106 = local read "FPGA_count2ms"() -> (w1897:dbl)
              n1107 = local read "sp_LeftSpout"() -> (w1923:u16)
              n1108 = local read "BUR_max"() -> (w1927:u16)
              n1109 = local read "sp_RightSpout"() -> (w1922:u16)
              n1110 = local read "BUR_min"() -> (w1929:u16)
              n1111 = Multiply(x=w1914, y=w1882) -> (x*y=w1913:dbl)
              n1112 = Multiply(x=w1907, y=w1882) -> (x*y=w1909:dbl)
              n1113 = Multiply(x=w1902, y=w1882) -> (x*y=w1904:dbl)
              n1114 = Multiply(x=w1897, y=w1882) -> (x*y=w1899:dbl)
              n1115 = Multiply(x=w1892, y=w1882) -> (x*y=w1894:dbl)
              n1116 = Multiply(x=w1881, y=w1882) -> (x*y=w1886:dbl)
              n1117 = Multiply(x=w1880, y=w1882) -> (x*y=w1884:dbl)
              n1118 = Round To Nearest(number=w1913) -> (nearest integer value=w1912:dbl)
              n1119 = Round To Nearest(number=w1909) -> (nearest integer value=w1908:dbl)
              n1120 = Round To Nearest(number=w1904) -> (nearest integer value=w1903:dbl)
              n1121 = Round To Nearest(number=w1899) -> (nearest integer value=w1898:dbl)
              n1122 = Round To Nearest(number=w1894) -> (nearest integer value=w1893:dbl)
              n1123 = Round To Nearest(number=w1886) -> (nearest integer value=w1885:dbl)
              n1124 = Round To Nearest(number=w1884) -> (nearest integer value=w1883:dbl)
              n1125 = To Unsigned Word Integer(number=w1912) -> (unsigned 16bit integer=w1911:u16)
              n1126 = To Unsigned Word Integer(number=w1908) -> (unsigned 16bit integer=w1906:u16)
              n1127 = To Unsigned Word Integer(number=w1903) -> (unsigned 16bit integer=w1901:u16)
              n1128 = To Unsigned Word Integer(number=w1898) -> (unsigned 16bit integer=w1896:u16)
              n1129 = To Unsigned Word Integer(number=w1893) -> (unsigned 16bit integer=w1891:u16)
              n1130 = To Unsigned Word Integer(number=w1885) -> (unsigned 16bit integer=w1879:u16)
              n1131 = To Unsigned Word Integer(number=w1883) -> (unsigned 16bit integer=w1878:u16)
              n1132 = local read "Laser_duration_l1"() -> (w1889:u16)
              n1133 = Replace Array Subset(array=w1931, new element #1=w1929, index #1=w1930, new element #2=w1927, index #2=w1928, new element #3=w1923, index #3=w1925, new element #4=w1922, index #4=w1924, new element #5=w1911, index #5=w1915, new element #6=w1906, index #6=w1910, new element #7=w1901, index #7=w1905, new element #8=w1896, index #8=w1900, new element #9=w1891, index #9=w1895, new element #10=w1879, index #10=w1888, new element #11=w1878, index #11=w1887, new element #12=w1889, index #12=w1890) -> (w1926:u16[])
            }
            frame "saveSettings4" {
              w1951 = 100.0 ("y")
              n1134 = call "myRIO_BRig_RT_dataExp_laser2_Freq.vi"() -> ("output_laser2_Freq"=w1940:i32)  [unwired: 11 in]
              n1135 = call "myRIO_BRig_RT_dataExp_laser2_Tpeak.vi"() -> ("output_laser2_Tpeak"=w1942:i32)  [unwired: 11 in]
              n1136 = call "myRIO_BRig_RT_dataExp_laser2_Tshutter.vi"() -> ("output_laser2_Tshutter"=w1944:i32)  [unwired: 11 in]
              n1137 = call "myRIO_BRig_RT_dataExp_laser2_Power_min.vi"() -> ("output_laser2_Power_min"=w1959:i32)  [unwired: 11 in]
              n1138 = call "myRIO_BRig_RT_dataExp_laser2_Power_max.vi"() -> ("output_laser2_Power_max"=w1958:i32)  [unwired: 11 in]
              n1139 = call "myRIO_BRig_RT_dataExp_laser2_Power_step.vi"() -> ("output_laser2_Power_step"=w1957:i32)  [unwired: 11 in]
              n1140 = call "myRIO_BRig_RT_dataExp_laser2_duration.vi"() -> ("output_laser2_duration"=w1956:i32)  [unwired: 11 in]
              n1141 = call "myRIO_BRig_RT_dataExp_CueLed_Freq.vi"() -> ("output_CueLed_Freq"=w1948:i32)  [unwired: 11 in]
              n1142 = call "myRIO_BRig_RT_dataExp_CueLed_Tpeak.vi"() -> ("output_CueLed_Tpeak"=w1947:i32)  [unwired: 11 in]
              n1143 = local read "Laser_Tshutter_l2"() -> (w1974:dbl)
              n1144 = local read "Laser_Tpeak_l2"() -> (w1977:dbl)
              n1145 = local read "Laser_power_max_l2"() -> (w1964:dbl)
              n1146 = local read "Laser_power_step_l2"() -> (w1963:dbl)
              n1147 = local read "Laser_power_min_l2"() -> (w1971:dbl)
              n1148 = local read "Laser_Freq_l2"() -> (w1982:dbl)
              n1149 = local read "CueLed_Tpeak"() -> (w1949:dbl)
              n1150 = local read "CueLed_Freq"() -> (w1950:dbl)
              n1151 = Multiply(x=w1982, y=w1951) -> (x*y=w1981:dbl)
              n1152 = Multiply(x=w1977, y=w1951) -> (x*y=w1979:dbl)
              n1153 = Multiply(x=w1974, y=w1951) -> (x*y=w1976:dbl)
              n1154 = Multiply(x=w1971, y=w1951) -> (x*y=w1973:dbl)
              n1155 = Multiply(x=w1964, y=w1951) -> (x*y=w1968:dbl)
              n1156 = Multiply(x=w1963, y=w1951) -> (x*y=w1966:dbl)
              n1157 = Multiply(x=w1950, y=w1951) -> (x*y=w1952:dbl)
              n1158 = Multiply(x=w1949, y=w1951) -> (x*y=w1953:dbl)
              n1159 = Round To Nearest(number=w1981) -> (nearest integer value=w1980:dbl)
              n1160 = Round To Nearest(number=w1979) -> (nearest integer value=w1978:dbl)
              n1161 = Round To Nearest(number=w1976) -> (nearest integer value=w1975:dbl)
              n1162 = Round To Nearest(number=w1973) -> (nearest integer value=w1972:dbl)
              n1163 = Round To Nearest(number=w1968) -> (nearest integer value=w1967:dbl)
              n1164 = Round To Nearest(number=w1966) -> (nearest integer value=w1965:dbl)
              n1165 = Round To Nearest(number=w1952) -> (nearest integer value=w1955:dbl)
              n1166 = Round To Nearest(number=w1953) -> (nearest integer value=w1954:dbl)
              n1167 = To Unsigned Word Integer(number=w1980) -> (unsigned 16bit integer=w1939:u16)
              n1168 = To Unsigned Word Integer(number=w1978) -> (unsigned 16bit integer=w1941:u16)
              n1169 = To Unsigned Word Integer(number=w1975) -> (unsigned 16bit integer=w1943:u16)
              n1170 = To Unsigned Word Integer(number=w1972) -> (unsigned 16bit integer=w1970:u16)
              n1171 = To Unsigned Word Integer(number=w1967) -> (unsigned 16bit integer=w1962:u16)
              n1172 = To Unsigned Word Integer(number=w1965) -> (unsigned 16bit integer=w1961:u16)
              n1173 = To Unsigned Word Integer(number=w1955) -> (unsigned 16bit integer=w1946:u16)
              n1174 = To Unsigned Word Integer(number=w1954) -> (unsigned 16bit integer=w1945:u16)
              n1175 = local read "Laser_duration_l2"() -> (w1969:u16)
              n1176 = Replace Array Subset(array=w1990, new element #1=w1939, index #1=w1940, new element #2=w1941, index #2=w1942, new element #3=w1943, index #3=w1944, new element #4=w1970, index #4=w1959, new element #5=w1962, index #5=w1958, new element #6=w1961, index #6=w1957, new element #7=w1969, index #7=w1956, new element #8=w1946, index #8=w1948, new element #9=w1945, index #9=w1947) -> (w1989:u16[])
            }
            frame "saveSettings_LC_ENL_l1" {
              # "Selection First"
              # "Count"
              # "Tdelay"
              # "Probability"
              # "OnOff"
              # "Block"
              # "delayOpt"
              # "Count"
              # "Tdelay"
              # "Probability"
              # "OnOff"
              # "Block"
              # "ENL1 All"
              # "delayOpt"
              # "Count"
              # "Tdelay"
              # "Probability"
              # "OnOff"
              # "Block"
              # "ENL1 First"
              n1177 = local read "LC_ENL1_delayOpt_Switch_l1"() -> (w2028:bool)
              n1178 = call "myRIO_BRig_RT_dataLC_ENL1_Block_NS_l1.vi"() -> ("output_ENL1_All_Block"=w2025:i32)  [unwired: 11 in]
              n1179 = call "myRIO_BRig_RT_dataLC_ENL1_OnOff_NS_l1.vi"() -> ("output_ENL1_OnOff_NS_l1"=w2015:i32)  [unwired: 11 in]
              n1180 = call "myRIO_BRig_RT_dataLC_ENL1_Probability_NS_l1.vi"() -> ("output_ENL1_Probability_NS_l1"=w2014:i32)  [unwired: 11 in]
              n1181 = call "myRIO_BRig_RT_dataLC_ENL1_Tdelay_NS_l1.vi"() -> ("output_ENL1_Tdelay_NS_l1"=w2013:i32)  [unwired: 11 in]
              n1182 = call "myRIO_BRig_RT_dataLC_ENL1_Count_NS_l1.vi"() -> ("output_ENL1_Count_NS_l1"=w2012:i32)  [unwired: 11 in]
              n1183 = call "myRIO_BRig_RT_dataLC_ENL1_delayOpt_NS_l1.vi"() -> ("output_ENL1_delayOpt_NS_l1"=w2011:i32)  [unwired: 11 in]
              n1184 = call "myRIO_BRig_RT_dataLC_ENL1_Block_Switch_l1.vi"() -> ("output_ENL1_Block_Switch_l1"=w2047:i32)  [unwired: 11 in]
              n1185 = call "myRIO_BRig_RT_dataLC_ENL1_OnOff_Switch_l1.vi"() -> ("output_ENL1_OnOff_Switch_l1"=w2045:i32)  [unwired: 11 in]
              n1186 = call "myRIO_BRig_RT_dataLC_ENL1_Probability_Switch_l1.vi"() -> ("output_ENL1_Probability_Switch_l1"=w2041:i32)  [unwired: 11 in]
              n1187 = call "myRIO_BRig_RT_dataLC_ENL1_Tdelay_Switch_l1.vi"() -> ("output_ENL1_Tdelay_Switch_l1"=w2039:i32)  [unwired: 11 in]
              n1188 = call "myRIO_BRig_RT_dataLC_ENL1_Count_Switch_l1.vi"() -> ("output_ENL1_Count_Switch_l1"=w2037:i32)  [unwired: 11 in]
              n1189 = call "myRIO_BRig_RT_dataLC_ENL1_delayOpt_Switch_l1.vi"() -> ("output_ENL1_delayOpt_Switch_l1"=w2027:i32)  [unwired: 11 in]
              n1190 = local read "LC_ENL1_Count_Switch_l1"() -> (w2036:u16)
              n1191 = local read "LC_ENL1_Probability_Switch_l1"() -> (w2040:u16)
              n1192 = local read "LC_ENL1_Block_Switch_l1"() -> (w2046:u16)
              n1193 = local read "LC_ENL1_Tdelay_Switch_l1"() -> (w2038:u16)
              n1194 = local read "LC_ENL1_OnOff_Switch_l1"() -> (w2044:bool)
              n1195 = call "myRIO_BRig_RT_dataLC_Selection_Block_Switch_l1.vi"() -> ("output_Selection_Block_Switch_l1"=w2009:i32)  [unwired: 11 in]
              n1196 = call "myRIO_BRig_RT_dataLC_Selection_OnOff_Switch_l1.vi"() -> ("output_Selection_OnOff_Switch_l1"=w2008:i32)  [unwired: 11 in]
              n1197 = call "myRIO_BRig_RT_dataLC_Selection_Probability_Switch_l1.vi"() -> ("output_Selection_Probability_Switch_l1"=w2007:i32)  [unwired: 11 in]
              n1198 = call "myRIO_BRig_RT_dataLC_Selection_Tdelay_Switch_l1.vi"() -> ("output_Selection_Tdelay_Switch_l1"=w2006:i32)  [unwired: 11 in]
              n1199 = call "myRIO_BRig_RT_dataLC_Selection_Count_Switch_l1.vi"() -> ("output_Selection_Count_Switch_l1"=w2005:i32)  [unwired: 11 in]
              n1200 = local read "LC_ENL1_OnOff_NS_l1"() -> (w2021:bool)
              n1201 = local read "LC_ENL1_Probability_NS_l1"() -> (w2019:u16)
              n1202 = local read "LC_ENL1_delayOpt_NS_l1"() -> (w2017:bool)
              n1203 = local read "LC_Sel_Probability_Switch_l1"() -> (w2000:u16)
              n1204 = local read "LC_ENL1_Tdelay_NS_l1"() -> (w2010:u16)
              n1205 = local read "LC_ENL1_Block_NS_l1"() -> (w2022:u16)
              n1206 = local read "LC_ENL1_Count_NS_l1"() -> (w2018:u16)
              n1207 = local read "LC_Sel_Tdelay_Switch_l1"() -> (w1999:u16)
              n1208 = local read "LC_Sel_OnOff_Switch_l1"() -> (w2003:bool)
              n1209 = local read "LC_Sel_Count_Switch_l1"() -> (w1998:u16)
              n1210 = local read "LC_Sel_Block_Switch_l1"() -> (w2002:u16)
              n1211 = Boolean To (0,1)(Boolean=w2028) -> (0, 1=w2029:i16)
              n1212 = Boolean To (0,1)(Boolean=w2044) -> (0, 1=w2043:i16)
              n1213 = Boolean To (0,1)(Boolean=w2021) -> (0, 1=w2024:i16)
              n1214 = To Unsigned Word Integer(number=w2029) -> (unsigned 16bit integer=w2026:u16)
              n1215 = To Unsigned Word Integer(number=w2043) -> (unsigned 16bit integer=w2042:u16)
              n1216 = Boolean To (0,1)(Boolean=w2017) -> (0, 1=w2023:i16)
              n1217 = To Unsigned Word Integer(number=w2024) -> (unsigned 16bit integer=w2020:u16)
              n1218 = Boolean To (0,1)(Boolean=w2003) -> (0, 1=w2004:i16)
              n1219 = To Unsigned Word Integer(number=w2023) -> (unsigned 16bit integer=w2016:u16)
              n1220 = To Unsigned Word Integer(number=w2004) -> (unsigned 16bit integer=w2001:u16)
              n1221 = Replace Array Subset(array=w2048, new element #1=w2046, index #1=w2047, new element #2=w2042, index #2=w2045, new element #3=w2040, index #3=w2041, new element #4=w2038, index #4=w2039, new element #5=w2036, index #5=w2037, new element #6=w2026, index #6=w2027, new element #7=w2022, index #7=w2025, new element #8=w2020, index #8=w2015, new element #9=w2019, index #9=w2014, new element #10=w2010, index #10=w2013, new element #11=w2018, index #11=w2012, new element #12=w2016, index #12=w2011, new element #13=w2002, index #13=w2009, new element #14=w2001, index #14=w2008, new element #15=w2000, index #15=w2007, new element #16=w1999, index #16=w2006, new element #17=w1998, index #17=w2005) -> (w2049:u16[])
            }
            frame "saveSettings_LC_ENL_l2" {
              # "Selection First"
              # "Count"
              # "Tdelay"
              # "Probability"
              # "OnOff"
              # "Block"
              # "delayOpt"
              # "Count"
              # "Tdelay"
              # "Probability"
              # "OnOff"
              # "Block"
              # "ENL1 All"
              # "delayOpt"
              # "Count"
              # "Tdelay"
              # "Probability"
              # "OnOff"
              # "Block"
              # "ENL1 First"
              n1222 = call "myRIO_BRig_RT_dataLC_ENL1_Block_Switch_l2.vi"() -> ("output_ENL1_Block_Switch_l2"=w2068:i32)  [unwired: 11 in]
              n1223 = call "myRIO_BRig_RT_dataLC_ENL1_OnOff_Switch_l2.vi"() -> ("output_ENL1_OnOff_Switch_l2"=w2069:i32)  [unwired: 11 in]
              n1224 = call "myRIO_BRig_RT_dataLC_ENL1_Probability_Switch_l2.vi"() -> ("output_ENL1_Probability_Switch_l2"=w2070:i32)  [unwired: 11 in]
              n1225 = call "myRIO_BRig_RT_dataLC_ENL1_Tdelay_Switch_l2.vi"() -> ("output_ENL1_Tdelay_Switch_l2"=w2071:i32)  [unwired: 11 in]
              n1226 = call "myRIO_BRig_RT_dataLC_ENL1_Count_Switch_l2.vi"() -> ("output_ENL1_Count_Switch_l2"=w2072:i32)  [unwired: 11 in]
              n1227 = call "myRIO_BRig_RT_dataLC_ENL1_delayOpt_Switch_l2.vi"() -> ("output_ENL1_delayOpt_Switch_l2"=w2073:i32)  [unwired: 11 in]
              n1228 = local read "LC_ENL1_delayOpt_Switch_l2"() -> (w2093:bool)
              n1229 = call "myRIO_BRig_RT_dataLC_ENL1_Block_NS_l2.vi"() -> ("output_ENL1_Block_NS_l2"=w2062:i32)  [unwired: 11 in]
              n1230 = call "myRIO_BRig_RT_dataLC_ENL1_OnOff_NS_l2.vi"() -> ("output_ENL1_OnOff_NS_l2"=w2063:i32)  [unwired: 11 in]
              n1231 = call "myRIO_BRig_RT_dataLC_ENL1_Probability_NS_l2.vi"() -> ("output_ENL1_Probability_NS_l2"=w2064:i32)  [unwired: 11 in]
              n1232 = call "myRIO_BRig_RT_dataLC_ENL1_Tdelay_NS_l2.vi"() -> ("output_ENL1_Tdelay_NS_l2"=w2065:i32)  [unwired: 11 in]
              n1233 = call "myRIO_BRig_RT_dataLC_ENL1_Count_NS_l2.vi"() -> ("output_ENL1_Count_NS_l2"=w2066:i32)  [unwired: 11 in]
              n1234 = call "myRIO_BRig_RT_dataLC_ENL1_delayOpt_NS_l2.vi"() -> ("output_ENL1_delayOpt_NS_l2"=w2067:i32)  [unwired: 11 in]
              n1235 = local read "LC_ENL1_Count_Switch_l2"() -> (w2101:u16)
              n1236 = local read "LC_ENL1_Probability_Switch_l2"() -> (w2103:u16)
              n1237 = local read "LC_ENL1_Block_Switch_l2"() -> (w2107:u16)
              n1238 = local read "LC_ENL1_Tdelay_Switch_l2"() -> (w2102:u16)
              n1239 = local read "LC_ENL1_OnOff_Switch_l2"() -> (w2106:bool)
              n1240 = call "myRIO_BRig_RT_dataLC_Selection_Block_Switch_l2.vi"() -> ("output_Selection_Block_Switch_l2"=w2061:i32)  [unwired: 11 in]
              n1241 = call "myRIO_BRig_RT_dataLC_Selection_OnOff_Switch_l2.vi"() -> ("output_Selection_OnOff_Switch_l2"=w2060:i32)  [unwired: 11 in]
              n1242 = call "myRIO_BRig_RT_dataLC_Selection_Probability_Switch_l2.vi"() -> ("output_Selection_Probability_Switch_l1"=w2059:i32)  [unwired: 11 in]
              n1243 = call "myRIO_BRig_RT_dataLC_Selection_Tdelay_Switch_l2.vi"() -> ("output_Selection_Tdelay_Switch_l2"=w2058:i32)  [unwired: 11 in]
              n1244 = call "myRIO_BRig_RT_dataLC_Selection_Count_Switch_l2.vi"() -> ("output_Selection_Count_Switch_l2"=w2057:i32)  [unwired: 11 in]
              n1245 = local read "LC_ENL1_OnOff_NS_l2"() -> (w2088:bool)
              n1246 = local read "LC_ENL1_Probability_NS_l2"() -> (w2086:u16)
              n1247 = local read "LC_ENL1_delayOpt_NS_l2"() -> (w2084:bool)
              n1248 = local read "LC_Sel_Probability_Switch_l2"() -> (w2077:u16)
              n1249 = local read "LC_ENL1_Tdelay_NS_l2"() -> (w2082:u16)
              n1250 = local read "LC_ENL1_Block_NS_l2"() -> (w2089:u16)
              n1251 = local read "LC_ENL1_Count_NS_l2"() -> (w2085:u16)
              n1252 = local read "LC_Sel_Tdelay_Switch_l2"() -> (w2076:u16)
              n1253 = local read "LC_Sel_OnOff_Switch_l2"() -> (w2080:bool)
              n1254 = local read "LC_Sel_Count_Switch_l2"() -> (w2075:u16)
              n1255 = local read "LC_Sel_Block_Switch_l2"() -> (w2079:u16)
              n1256 = Boolean To (0,1)(Boolean=w2093) -> (0, 1=w2094:i16)
              n1257 = Boolean To (0,1)(Boolean=w2106) -> (0, 1=w2105:i16)
              n1258 = Boolean To (0,1)(Boolean=w2088) -> (0, 1=w2091:i16)
              n1259 = To Unsigned Word Integer(number=w2094) -> (unsigned 16bit integer=w2092:u16)
              n1260 = To Unsigned Word Integer(number=w2105) -> (unsigned 16bit integer=w2104:u16)
              n1261 = Boolean To (0,1)(Boolean=w2084) -> (0, 1=w2090:i16)
              n1262 = To Unsigned Word Integer(number=w2091) -> (unsigned 16bit integer=w2087:u16)
              n1263 = Boolean To (0,1)(Boolean=w2080) -> (0, 1=w2081:i16)
              n1264 = To Unsigned Word Integer(number=w2090) -> (unsigned 16bit integer=w2083:u16)
              n1265 = To Unsigned Word Integer(number=w2081) -> (unsigned 16bit integer=w2078:u16)
              n1266 = Replace Array Subset(array=w2108, new element #1=w2107, index #1=w2068, new element #2=w2104, index #2=w2069, new element #3=w2103, index #3=w2070, new element #4=w2102, index #4=w2071, new element #5=w2101, index #5=w2072, new element #6=w2092, index #6=w2073, new element #7=w2089, index #7=w2062, new element #8=w2087, index #8=w2063, new element #9=w2086, index #9=w2064, new element #10=w2082, index #10=w2065, new element #11=w2085, index #11=w2066, new element #12=w2083, index #12=w2067, new element #13=w2079, index #13=w2061, new element #14=w2078, index #14=w2060, new element #15=w2077, index #15=w2059, new element #16=w2076, index #16=w2058, new element #17=w2075, index #17=w2057) -> (w2109:u16[])
            }
            frame "saveSettings_LC_Cue_l1" {
              # "Selection All"
              # "Count"
              # "Tdelay"
              # "Probability"
              # "OnOff"
              # "Block"
              # "delayOpt"
              # "Count"
              # "Tdelay"
              # "Probability"
              # "OnOff"
              # "Block"
              # "Cue1 All"
              # "delayOpt"
              # "Count"
              # "Tdelay"
              # "Probability"
              # "OnOff"
              # "Block"
              # "Cue1 First"
              n1267 = call "myRIO_BRig_RT_dataLC_Cue1_delayOpt_Switch_l1.vi"() -> ("output_Cue1_delayOpt_Switch_l1"=w2148:i32)  [unwired: 11 in]
              n1268 = call "myRIO_BRig_RT_dataLC_Cue1_Block_Switch_l1.vi"() -> ("output_Cue1_Block_Switch_l1"=w2167:i32)  [unwired: 11 in]
              n1269 = call "myRIO_BRig_RT_dataLC_Cue1_OnOff_Switch_l1.vi"() -> ("output_Cue1_OnOff_Switch_l1"=w2165:i32)  [unwired: 11 in]
              n1270 = call "myRIO_BRig_RT_dataLC_Cue1_Probability_Switch_l1.vi"() -> ("output_Cue1_Probability_Switch_l1"=w2161:i32)  [unwired: 11 in]
              n1271 = call "myRIO_BRig_RT_dataLC_Cue1_Tdelay_Switch_l1.vi"() -> ("output_Cue1_Tdelay_Switch_l1"=w2159:i32)  [unwired: 11 in]
              n1272 = call "myRIO_BRig_RT_dataLC_Cue1_Count_Switch_l1.vi"() -> ("output_Cue1_Count_Switch_l1"=w2157:i32)  [unwired: 11 in]
              n1273 = local read "LC_Cue1_delayOpt_Switch_l1"() -> (w2147:bool)
              n1274 = call "myRIO_BRig_RT_dataLC_Cue1_Block_NS_l1.vi"() -> ("output_Cue1_Block_NS_l1"=w2145:i32)  [unwired: 11 in]
              n1275 = call "myRIO_BRig_RT_dataLC_Cue1_OnOff_NS_l1.vi"() -> ("output_Cue1_OnOff_NS_l1"=w2144:i32)  [unwired: 11 in]
              n1276 = call "myRIO_BRig_RT_dataLC_Cue1_Probability_NS_l1.vi"() -> ("output_Cue1_l1_All_Probability"=w2143:i32)  [unwired: 11 in]
              n1277 = call "myRIO_BRig_RT_dataLC_Cue1_Tdelay_NS_l1.vi"() -> ("output_Cue1_Tdelay_NS_l1"=w2142:i32)  [unwired: 11 in]
              n1278 = call "myRIO_BRig_RT_dataLC_Cue1_Count_NS_l1.vi"() -> ("output_Cue1_Count_NS_l1"=w2141:i32)  [unwired: 11 in]
              n1279 = call "myRIO_BRig_RT_dataLC_Cue1_delayOpt_NS_l1.vi"() -> ("output_Cue1_delayOpt_NS_l1"=w2140:i32)  [unwired: 11 in]
              n1280 = local read "LC_Cue1_Count_Switch_l1"() -> (w2156:u16)
              n1281 = local read "LC_Cue1_Probability_Switch_l1"() -> (w2160:u16)
              n1282 = local read "LC_Cue1_Block_Switch_l1"() -> (w2166:u16)
              n1283 = local read "LC_Cue1_Tdelay_Switch_l1"() -> (w2158:u16)
              n1284 = local read "LC_Cue1_OnOff_Switch_l1"() -> (w2164:bool)
              n1285 = local read "LC_Cue1_OnOff_NS_l1"() -> (w2136:bool)
              n1286 = call "myRIO_BRig_RT_dataLC_Selection_Block_NS_l1.vi"() -> ("output_Selection_Block_NS_l1"=w2129:i32)  [unwired: 11 in]
              n1287 = call "myRIO_BRig_RT_dataLC_Selection_OnOff_NS_l1.vi"() -> ("output_Selection_OnOff_NS_l1"=w2128:i32)  [unwired: 11 in]
              n1288 = call "myRIO_BRig_RT_dataLC_Selection_Probability_NS_l1.vi"() -> ("output_Selection_Probability_NS_l1"=w2127:i32)  [unwired: 11 in]
              n1289 = call "myRIO_BRig_RT_dataLC_Selection_Tdelay_NS_l1.vi"() -> ("output_Selection_Tdelay_NS_l1"=w2126:i32)  [unwired: 11 in]
              n1290 = call "myRIO_BRig_RT_dataLC_Selection_Count_NS_l1.vi"() -> ("output_Selection_Count_NS_l1"=w2119:i32)  [unwired: 11 in]
              n1291 = local read "LC_Cue1_delayOpt_NS_l1"() -> (w2137:bool)
              n1292 = local read "LC_Cue1_Probability_NS_l1"() -> (w2133:u16)
              n1293 = local read "LC_Cue1_Tdelay_NS_l1"() -> (w2132:u16)
              n1294 = local read "LC_Cue1_Count_NS_l1"() -> (w2131:u16)
              n1295 = local read "LC_Cue1_Block_NS_l1"() -> (w2135:u16)
              n1296 = local read "LC_Sel_Probability_NS_l1"() -> (w2121:u16)
              n1297 = local read "LC_Sel_Tdelay_NS_l1"() -> (w2120:u16)
              n1298 = local read "LC_Sel_OnOff_NS_l1"() -> (w2123:bool)
              n1299 = local read "LC_Sel_Count_NS_l1"() -> (w2118:u16)
              n1300 = local read "LC_Sel_Block_NS_l1"() -> (w2125:u16)
              n1301 = Boolean To (0,1)(Boolean=w2147) -> (0, 1=w2149:i16)
              n1302 = Boolean To (0,1)(Boolean=w2164) -> (0, 1=w2163:i16)
              n1303 = Boolean To (0,1)(Boolean=w2136) -> (0, 1=w2139:i16)
              n1304 = To Unsigned Word Integer(number=w2149) -> (unsigned 16bit integer=w2146:u16)
              n1305 = To Unsigned Word Integer(number=w2163) -> (unsigned 16bit integer=w2162:u16)
              n1306 = To Unsigned Word Integer(number=w2139) -> (unsigned 16bit integer=w2134:u16)
              n1307 = Boolean To (0,1)(Boolean=w2137) -> (0, 1=w2138:i16)
              n1308 = Boolean To (0,1)(Boolean=w2123) -> (0, 1=w2124:i16)
              n1309 = To Unsigned Word Integer(number=w2138) -> (unsigned 16bit integer=w2130:u16)
              n1310 = To Unsigned Word Integer(number=w2124) -> (unsigned 16bit integer=w2122:u16)
              n1311 = Replace Array Subset(array=w2168, new element #1=w2166, index #1=w2167, new element #2=w2162, index #2=w2165, new element #3=w2160, index #3=w2161, new element #4=w2158, index #4=w2159, new element #5=w2156, index #5=w2157, new element #6=w2146, index #6=w2148, new element #7=w2135, index #7=w2145, new element #8=w2134, index #8=w2144, new element #9=w2133, index #9=w2143, new element #10=w2132, index #10=w2142, new element #11=w2131, index #11=w2141, new element #12=w2130, index #12=w2140, new element #13=w2125, index #13=w2129, new element #14=w2122, index #14=w2128, new element #15=w2121, index #15=w2127, new element #16=w2120, index #16=w2126, new element #17=w2118, index #17=w2119) -> (w2169:u16[])
            }
            frame "saveSettings_LC_Cue_l2" {
              # "Selection All"
              # "Count"
              # "Tdelay"
              # "Probability"
              # "OnOff"
              # "Block"
              # "delayOpt"
              # "Count"
              # "Tdelay"
              # "Probability"
              # "OnOff"
              # "Block"
              # "Cue1 All"
              # "delayOpt"
              # "Count"
              # "Tdelay"
              # "Probability"
              # "OnOff"
              # "Block"
              # "Cue1 First"
              n1312 = call "myRIO_BRig_RT_dataLC_Cue1_delayOpt_Switch_l2.vi"() -> ("output_Cue1_delayOpt_Switch_l2"=w2208:i32)  [unwired: 11 in]
              n1313 = call "myRIO_BRig_RT_dataLC_Cue1_Block_Switch_l2.vi"() -> ("output_Cue1_Block_Switch_l2"=w2227:i32)  [unwired: 11 in]
              n1314 = call "myRIO_BRig_RT_dataLC_Cue1_OnOff_Switch_l2.vi"() -> ("output_Cue1_OnOff_Switch_l2"=w2225:i32)  [unwired: 11 in]
              n1315 = call "myRIO_BRig_RT_dataLC_Cue1_Probability_Switch_l2.vi"() -> ("output_Cue1_l2_First_Probability"=w2221:i32)  [unwired: 11 in]
              n1316 = call "myRIO_BRig_RT_dataLC_Cue1_Tdelay_Switch_l2.vi"() -> ("output_Cue1_Tdelay_Switch_l2"=w2219:i32)  [unwired: 11 in]
              n1317 = call "myRIO_BRig_RT_dataLC_Cue1_Count_Switch_l2.vi"() -> ("output_Cue1_Count_Switch_l2"=w2217:i32)  [unwired: 11 in]
              n1318 = local read "LC_Cue1_delayOpt_Switch_l2"() -> (w2207:bool)
              n1319 = call "myRIO_BRig_RT_dataLC_Cue1_Block_NS_l2.vi"() -> ("output_Cue1_Block_NS_l2"=w2205:i32)  [unwired: 11 in]
              n1320 = call "myRIO_BRig_RT_dataLC_Cue1_OnOff_NS_l2.vi"() -> ("output_Cue1_OnOff_NS_l2"=w2204:i32)  [unwired: 11 in]
              n1321 = call "myRIO_BRig_RT_dataLC_Cue1_Probability_NS_l2.vi"() -> ("output_Cue1_l2_All_Probability"=w2203:i32)  [unwired: 11 in]
              n1322 = call "myRIO_BRig_RT_dataLC_Cue1_Tdelay_NS_l2.vi"() -> ("output_Cue1_Tdelay_NS_l2"=w2202:i32)  [unwired: 11 in]
              n1323 = call "myRIO_BRig_RT_dataLC_Cue1_Count_NS_l2.vi"() -> ("output_Cue1_Count_NS_l2"=w2201:i32)  [unwired: 11 in]
              n1324 = call "myRIO_BRig_RT_dataLC_Cue1_delayOpt_NS_l2.vi"() -> ("output_Cue1_delayOpt_NS_l2"=w2200:i32)  [unwired: 11 in]
              n1325 = local read "LC_Cue1_Count_Switch_l2"() -> (w2216:u16)
              n1326 = local read "LC_Cue1_Probability_Switch_l2"() -> (w2220:u16)
              n1327 = local read "LC_Cue1_Block_Switch_l2"() -> (w2226:u16)
              n1328 = local read "LC_Cue1_Tdelay_Switch_l2"() -> (w2218:u16)
              n1329 = local read "LC_Cue1_OnOff_Switch_l2"() -> (w2224:bool)
              n1330 = local read "LC_Cue1_OnOff_NS_l2"() -> (w2196:bool)
              n1331 = call "myRIO_BRig_RT_dataLC_Selection_Block_NS_l2.vi"() -> ("output_Selection_Block_NS_l2"=w2181:i32)  [unwired: 11 in]
              n1332 = call "myRIO_BRig_RT_dataLC_Selection_OnOff_NS_l2.vi"() -> ("output_Selection_OnOff_NS_l2"=w2180:i32)  [unwired: 11 in]
              n1333 = call "myRIO_BRig_RT_dataLC_Selection_Probability_NS_l2.vi"() -> ("output_Selection_Probability_NS_l2"=w2179:i32)  [unwired: 11 in]
              n1334 = call "myRIO_BRig_RT_dataLC_Selection_Tdelay_NS_l2.vi"() -> ("output_Selection_Tdelay_NS_l2"=w2178:i32)  [unwired: 11 in]
              n1335 = call "myRIO_BRig_RT_dataLC_Selection_Count_NS_l2.vi"() -> ("output_Selection_Count_NS_l2"=w2177:i32)  [unwired: 11 in]
              n1336 = local read "LC_Cue1_delayOpt_NS_l2"() -> (w2197:bool)
              n1337 = local read "LC_Cue1_Probability_NS_l2"() -> (w2193:u16)
              n1338 = local read "LC_Cue1_Tdelay_NS_l2"() -> (w2192:u16)
              n1339 = local read "LC_Cue1_Count_NS_l2"() -> (w2191:u16)
              n1340 = local read "LC_Cue1_Block_NS_l2"() -> (w2195:u16)
              n1341 = local read "LC_Sel_Probability_NS_l2"() -> (w2185:u16)
              n1342 = local read "LC_Sel_Tdelay_NS_l2"() -> (w2184:u16)
              n1343 = local read "LC_Sel_OnOff_NS_l2"() -> (w2187:bool)
              n1344 = local read "LC_Sel_Count_NS_l2"() -> (w2183:u16)
              n1345 = local read "LC_Sel_Block_NS_l2"() -> (w2189:u16)
              n1346 = Boolean To (0,1)(Boolean=w2207) -> (0, 1=w2209:i16)
              n1347 = Boolean To (0,1)(Boolean=w2224) -> (0, 1=w2223:i16)
              n1348 = Boolean To (0,1)(Boolean=w2196) -> (0, 1=w2199:i16)
              n1349 = To Unsigned Word Integer(number=w2209) -> (unsigned 16bit integer=w2206:u16)
              n1350 = To Unsigned Word Integer(number=w2223) -> (unsigned 16bit integer=w2222:u16)
              n1351 = To Unsigned Word Integer(number=w2199) -> (unsigned 16bit integer=w2194:u16)
              n1352 = Boolean To (0,1)(Boolean=w2197) -> (0, 1=w2198:i16)
              n1353 = Boolean To (0,1)(Boolean=w2187) -> (0, 1=w2188:i16)
              n1354 = To Unsigned Word Integer(number=w2198) -> (unsigned 16bit integer=w2190:u16)
              n1355 = To Unsigned Word Integer(number=w2188) -> (unsigned 16bit integer=w2186:u16)
              n1356 = Replace Array Subset(array=w2228, new element #1=w2226, index #1=w2227, new element #2=w2222, index #2=w2225, new element #3=w2220, index #3=w2221, new element #4=w2218, index #4=w2219, new element #5=w2216, index #5=w2217, new element #6=w2206, index #6=w2208, new element #7=w2195, index #7=w2205, new element #8=w2194, index #8=w2204, new element #9=w2193, index #9=w2203, new element #10=w2192, index #10=w2202, new element #11=w2191, index #11=w2201, new element #12=w2190, index #12=w2200, new element #13=w2189, index #13=w2181, new element #14=w2186, index #14=w2180, new element #15=w2185, index #15=w2179, new element #16=w2184, index #16=w2178, new element #17=w2183, index #17=w2177) -> (w2229:u16[])
            }
            frame "saveSettings6_LC_l1_Other" {
              # "Trial"
              # "Tdelay"
              # "Probability"
              # "OnOff"
              # "Block"
              # "Wrong"
              # "Trial"
              # "Tdelay"
              # "Probability"
              # "OnOff"
              # "Block"
              # "Reward"
              n1357 = call "myRIO_BRig_RT_dataLC_Wrong_Block_l1.vi"() -> ("output_Wrong_Block_l1"=w2254:i32)  [unwired: 11 in]
              n1358 = call "myRIO_BRig_RT_dataLC_Wrong_OnOff_l1.vi"() -> ("output_Wrong_OnOff_l1"=w2253:i32)  [unwired: 11 in]
              n1359 = call "myRIO_BRig_RT_dataLC_Wrong_Probability_l1.vi"() -> ("output_Wrong_Probability_l1"=w2252:i32)  [unwired: 11 in]
              n1360 = call "myRIO_BRig_RT_dataLC_Wrong_Tdelay_l1.vi"() -> ("output_Wrong_Tdelay_l1"=w2251:i32)  [unwired: 11 in]
              n1361 = call "myRIO_BRig_RT_dataLC_Wrong_Trial_l1.vi"() -> ("output_Wrong_Trial_l1"=w2250:i32)  [unwired: 11 in]
              n1362 = call "myRIO_BRig_RT_dataLC_Reward_Block_l1.vi"() -> ("output_Reward_Block_l1"=w2266:i32)  [unwired: 11 in]
              n1363 = call "myRIO_BRig_RT_dataLC_Reward_OnOff_l1.vi"() -> ("output_Reward_OnOff_l1"=w2264:i32)  [unwired: 11 in]
              n1364 = call "myRIO_BRig_RT_dataLC_Reward_Probability_l1.vi"() -> ("output_Reward_Probability_l1"=w2260:i32)  [unwired: 11 in]
              n1365 = call "myRIO_BRig_RT_dataLC_Reward_Tdelay_l1.vi"() -> ("output_Reward_Tdelay_l1"=w2258:i32)  [unwired: 11 in]
              n1366 = call "myRIO_BRig_RT_dataLC_Reward_Trial_l1.vi"() -> ("output_Reward_Trial_l1"=w2256:i32)  [unwired: 11 in]
              n1367 = local read "LC_Wrong_OnOff_l1"() -> (w2248:bool)
              n1368 = local read "LC_Wrong_Probability_l1"() -> (w2245:u16)
              n1369 = local read "LC_Wrong_Block_l1"() -> (w2247:u16)
              n1370 = local read "LC_Wrong_Tdelay_l1"() -> (w2244:u16)
              n1371 = local read "LC_Wrong_Trial_l1"() -> (w2243:u16)
              n1372 = local read "LC_Reward_Probability_l1"() -> (w2259:u16)
              n1373 = local read "LC_Reward_Block_l1"() -> (w2265:u16)
              n1374 = local read "LC_Reward_Tdelay_l1"() -> (w2257:u16)
              n1375 = local read "LC_Reward_OnOff_l1"() -> (w2263:bool)
              n1376 = local read "LC_Reward_Trial_l1"() -> (w2255:u16)
              n1377 = Boolean To (0,1)(Boolean=w2248) -> (0, 1=w2249:i16)
              n1378 = Boolean To (0,1)(Boolean=w2263) -> (0, 1=w2262:i16)
              n1379 = To Unsigned Word Integer(number=w2249) -> (unsigned 16bit integer=w2246:u16)
              n1380 = To Unsigned Word Integer(number=w2262) -> (unsigned 16bit integer=w2261:u16)
              n1381 = Replace Array Subset(array=w2267, new element #1=w2265, index #1=w2266, new element #2=w2261, index #2=w2264, new element #3=w2259, index #3=w2260, new element #4=w2257, index #4=w2258, new element #5=w2255, index #5=w2256, new element #6=w2247, index #6=w2254, new element #7=w2246, index #7=w2253, new element #8=w2245, index #8=w2252, new element #9=w2244, index #9=w2251, new element #10=w2243, index #10=w2250) -> (w2268:u16[])
            }
            frame "SaveSettings6_LC_l2_Other" {
              # "Trial"
              # "Tdelay"
              # "Probability"
              # "OnOff"
              # "Block"
              # "Wrong"
              # "Trial"
              # "Tdelay"
              # "Probability"
              # "OnOff"
              # "Block"
              # "Reward"
              n1382 = call "myRIO_BRig_RT_dataLC_Wrong_Block_l2.vi"() -> ("output_Wrong_Block_l2"=w2277:i32)  [unwired: 11 in]
              n1383 = call "myRIO_BRig_RT_dataLC_Wrong_OnOff_l2.vi"() -> ("output_Wrong_OnOff_l2"=w2278:i32)  [unwired: 11 in]
              n1384 = call "myRIO_BRig_RT_dataLC_Wrong_Probability_l2.vi"() -> ("output_Wrong_Probability_l2"=w2279:i32)  [unwired: 11 in]
              n1385 = call "myRIO_BRig_RT_dataLC_Wrong_Tdelay_l2.vi"() -> ("output_Wrong_Tdelay_l2"=w2280:i32)  [unwired: 11 in]
              n1386 = call "myRIO_BRig_RT_dataLC_Wrong_Trial_l2.vi"() -> ("output_Wrong_Trial_l2"=w2281:i32)  [unwired: 11 in]
              n1387 = call "myRIO_BRig_RT_dataLC_Reward_Block_l2.vi"() -> ("output_Reward_Block_l2"=w2282:i32)  [unwired: 11 in]
              n1388 = call "myRIO_BRig_RT_dataLC_Reward_OnOff_l2.vi"() -> ("output_Reward_OnOff_l2"=w2283:i32)  [unwired: 11 in]
              n1389 = call "myRIO_BRig_RT_dataLC_Reward_Probability_l2.vi"() -> ("output_Reward_Probability_l2"=w2284:i32)  [unwired: 11 in]
              n1390 = call "myRIO_BRig_RT_dataLC_Reward_Tdelay_l2.vi"() -> ("output_Reward_Tdelay_l2"=w2285:i32)  [unwired: 11 in]
              n1391 = call "myRIO_BRig_RT_dataLC_Reward_Trial_l2.vi"() -> ("output_Reward_Trial_l2"=w2286:i32)  [unwired: 11 in]
              n1392 = local read "LC_Wrong_OnOff_l2"() -> (w2298:bool)
              n1393 = local read "LC_Wrong_Probability_l2"() -> (w2295:u16)
              n1394 = local read "LC_Wrong_Block_l2"() -> (w2297:u16)
              n1395 = local read "LC_Wrong_Tdelay_l2"() -> (w2294:u16)
              n1396 = local read "LC_Wrong_Trial_l2"() -> (w2293:u16)
              n1397 = local read "LC_Reward_Probability_l2"() -> (w2302:u16)
              n1398 = local read "LC_Reward_Block_l2"() -> (w2306:u16)
              n1399 = local read "LC_Reward_Tdelay_l2"() -> (w2301:u16)
              n1400 = local read "LC_Reward_OnOff_l2"() -> (w2305:bool)
              n1401 = local read "LC_Reward_Trial_l2"() -> (w2300:u16)
              n1402 = Boolean To (0,1)(Boolean=w2298) -> (0, 1=w2299:i16)
              n1403 = Boolean To (0,1)(Boolean=w2305) -> (0, 1=w2304:i16)
              n1404 = To Unsigned Word Integer(number=w2299) -> (unsigned 16bit integer=w2296:u16)
              n1405 = To Unsigned Word Integer(number=w2304) -> (unsigned 16bit integer=w2303:u16)
              n1406 = Replace Array Subset(array=w2307, new element #1=w2306, index #1=w2282, new element #2=w2303, index #2=w2283, new element #3=w2302, index #3=w2284, new element #4=w2301, index #4=w2285, new element #5=w2300, index #5=w2286, new element #6=w2297, index #6=w2277, new element #7=w2296, index #7=w2278, new element #8=w2295, index #8=w2279, new element #9=w2294, index #9=w2280, new element #10=w2293, index #10=w2281) -> (w2308:u16[])
            }
            frame "setSettings_Audio" {
              # "amp_L"
              # "amp_R"
              # "freq_L"
              # "freq_R"
              n1407 = call "myRIO_BRig_RT_dataExp_Audio_amp__L.vi"() -> ("output_Audio_amp__L"=w2336:i32)  [unwired: 11 in]
              n1408 = call "myRIO_BRig_RT_dataExp_Audio_amp__R.vi"() -> ("output_Audio_amp__R"=w2335:i32)  [unwired: 11 in]
              n1409 = call "myRIO_BRig_RT_dataExp_Audio_freq__L.vi"() -> ("output_Audio_freq__L"=w2334:i32)  [unwired: 11 in]
              n1410 = call "myRIO_BRig_RT_dataExp_Audio_freq__R.vi"() -> ("output_Audio_freq__R"=w2333:i32)  [unwired: 11 in]
              n1411 = Index Array(array=w2332, index #1=w2336, index #2=w2335, index #3=w2334, index #4=w2333) -> (element #1=w2321:u16, element #2=w2320:u16, element #3=w2325:u16, element #4=w2324:u16)
              n1412 = To Unsigned Byte Integer(number=w2325) -> (unsigned 8bit integer=w2319:u8)
              n1413 = To Unsigned Byte Integer(number=w2324) -> (unsigned 8bit integer=w2318:u8)
              n1414 = xnode "Read/Write Control"("FPGA VI Reference In"=w2323, "error in"=w2322, "audioAmp_L"=w2321, "audioAmp_R"=w2320, "audioFreq_L_kHz"=w2319, "audioFreq_R_kHz"=w2318) -> ("error out"=w2317:errorcluster)  [unwired: 1 out]
              n1415 = local write "error out"(w2317) -> ()
            }
            frame "setSettings_Laser" {
              w2367 = u32 0 ("laser2_selRew_Ndelay")
              # "tDelay"
              # "Wrong l1"
              # "Reward l1"
              n1416 = call "myRIO_BRig_RT_dataExp_IallReward.vi"() -> ("output_I_allReward"=w2348:i32)  [unwired: 11 in]
              n1417 = local read "Laser_Tpeak_l1"() -> (w2378:dbl)
              n1418 = local read "Laser_Tshutter_l1"() -> (w2376:dbl)
              n1419 = local read "Laser_Freq_l1"() -> (w2377:dbl)
              n1420 = local read "Laser_duration_l1"() -> (w2352:u16)
              n1421 = local read "Laser_Tpeak_l2"() -> (w2374:dbl)
              n1422 = local read "Laser_Tshutter_l2"() -> (w2372:dbl)
              n1423 = local read "Laser_Freq_l2"() -> (w2373:dbl)
              n1424 = local read "Laser_duration_l2"() -> (w2351:u16)
              n1425 = local read "CueLed_Freq"() -> (w2361:dbl)
              n1426 = local read "CueLed_Tpeak"() -> (w2362:dbl)
              n1427 = local read "I_allReward"() -> (w2347:bool)
              n1428 = call "myRIO_BRig_RT_dataLC_Reward_Tdelay_l1.vi"() -> ("output_Reward_Tdelay_l1"=w2390:i32)  [unwired: 11 in]
              n1429 = call "myRIO_BRig_RT_dataLC_Wrong_Tdelay_l1.vi"() -> ("output_Wrong_Tdelay_l1"=w2391:i32)  [unwired: 11 in]
              n1430 = local read "FPGA_count2ms"() -> (w2363:dbl)
              n1431 = Index Array(array=w2358, index #1=w2390, index #2=w2391) -> (element #1=w2389:u16, element #2=w2388:u16)
              n1432 = To Double Precision Float(number=w2389) -> (double precision float=w2385:dbl)
              n1433 = To Double Precision Float(number=w2388) -> (double precision float=w2382:dbl)
              n1434 = Boolean To (0,1)(Boolean=w2347) -> (0, 1=w2346:i16)
              n1435 = To Unsigned Word Integer(number=w2346) -> (unsigned 16bit integer=w2345:u16)
              n1436 = Replace Array Subset(array=w2350, new element=w2345, index=w2348) -> (w2349:u16[])
              n1437 = To Unsigned Word Integer(number=w2363) -> (unsigned 16bit integer=w2379:u16)
              n1438 = call "myRIO_BRig_RT__calc_laser_FPGA_N.vi"("input_FPGA_ms2count"=w2363, "input_Tpeak"=w2378, "input_Freq"=w2377, "input_Tshutter"=w2376, "input_duration"=w2352) -> ("output_laser_Npeak"=w2366:u32, "output_laser_Nvalley"=w2365:u32, "output_laser_Nshutter"=w2364:u32, "output_laser_Nduration"=w2375:u32, "output_laser_Tduration"=w2356:u16)  [unwired: 6 in]
              n1439 = Multiply(x=w2363, y=w2385) -> (x*y=w2386:dbl)
              n1440 = Multiply(x=w2363, y=w2382) -> (x*y=w2383:dbl)
              n1441 = call "myRIO_BRig_RT__calc_laser_FPGA_N__CueLed.vi"("input_FPGA_ms2count"=w2363, "input_Tpeak"=w2362, "input_Freq"=w2361) -> ("output_laser_Npeak"=w2360:u32, "output_laser_Nvalley"=w2359:u32)  [unwired: 11 in]
              n1442 = call "myRIO_BRig_RT__calc_laser_FPGA_N.vi"("input_FPGA_ms2count"=w2363, "input_Tpeak"=w2374, "input_Freq"=w2373, "input_Tshutter"=w2372, "input_duration"=w2351) -> ("output_laser_Npeak"=w2371:u32, "output_laser_Nvalley"=w2370:u32, "output_laser_Nshutter"=w2369:u32, "output_laser_Nduration"=w2368:u32, "output_laser_Tduration"=w2355:u16)  [unwired: 6 in]
              n1443 = Round Toward +Infinity(x=w2386) -> (ceil(x): smallest int >= x=w2387:dbl)
              n1444 = Round Toward +Infinity(x=w2383) -> (ceil(x): smallest int >= x=w2384:dbl)
              n1445 = To Unsigned Long Integer(number=w2387) -> (unsigned 32bit integer=w2381:u32)
              n1446 = To Unsigned Long Integer(number=w2384) -> (unsigned 32bit integer=w2380:u32)
              n1447 = xnode "Read/Write Control"("FPGA VI Reference In"=w2392, "error in"=w2393, "I_allReward"=w2347, "LC_nPeak_l1"=w2366, "LC_nValley_l1"=w2365, "LC_nShutter_l1"=w2364, "LR_reward_nDelay_l1"=w2381, "LR_wrong_nDelay_l1"=w2380, "LR_reward_nTotal_l1"=w2375, "LR_wrong_nTotal_l1"=w2375, "k1__counter_per_ms"=w2379, "LC_nPeak_l2"=w2371, "LC_nValley_l2"=w2370, "LC_nShutter_l2"=w2369, "LR_reward_nDelay_l2"=w2367, "LR_wrong_nDelay_l2"=w2367, "LR_reward_nTotal_l2"=w2368, "LR_wrong_nTotal_l2"=w2368, "CueLed_nPeak"=w2360, "CueLed_nValley"=w2359) -> ("error out"=→"error out":errorcluster)  [unwired: 1 out]
              n1448 = call "myRIO_BRig_RT_dataCurrent_laser1_pulse_duration.vi"() -> ("output_laser1_pulse_duration"=w2354:i32)  [unwired: 11 in]
              n1449 = call "myRIO_BRig_RT_dataCurrent_laser2_pulse_duration.vi"() -> ("output_laser2_pulse_duration"=w2353:i32)  [unwired: 11 in]
              n1450 = Replace Array Subset(array=w2358, new element #1=w2356, index #1=w2354, new element #2=w2355, index #2=w2353) -> (w2357:u16[])
            }
            frame "initBlock" {
              n1451 = local write "nRewards_cur"(u16 0 ("nRewards_cur")) -> ()
              n1452 = call "myRIO_Brig_RT__Case_Exp_State_initBlock__v2.vi"("input_spout"=w2414, "input_dataCurrent"=w2420, "input_dataExp"=w2417, "input_dataBlock"=w2409) -> ("output_state"=w2413:T2, "output_spout"=w2412:enum16{"Left", "Right"}, "idxDataBlock"=w2415:i32, "output_dataCurrent"=w2419:u16[], "output_dataExp"=w2418:u16[], "output_TpB_target"=→"TpB_target":u16, "output_iBlock"=w2410:u16, "output_dataBlock"=w2408:u16[][])  [unwired: 4 in]
              "iBlock" <- w2410
              "cSpout" <- w2412
            }
            frame "initBlock2" {
              n1453 = call "myRIO_BRig_RT__Case_Exp_State_initBlock2.vi"("input_spout"=w2437, "input_dataBlock"=w2438, "input_dataCurrent"=w2436) -> ("idxDataBlock"=w2433:i32, "output_dataBlock"=w2435:u16[][])  [unwired: 7 in]
            }
            frame "initTrial" {
              n1454 = xnode "Read/Write Control"("FPGA VI Reference In"=w2453, "error in"=w2452, "SelectionState"=FALSE) -> ("error out"=w2451:errorcluster)  [unwired: 1 out]
              n1455 = call "myRIO_Brig_RT__Case_Exp_State_initTrial__v2.vi"("input_spout"=w2454, "input_dataBlock"=w2449, "input_dataExp"=w2465, "input_dataCurrent"=w2466) -> ("output_state"=w2467:T2, "output_dataExp"=w2464:u16[], "output_dataCurrent"=w2459:u16[], "output_iTrial"=w2448:u16, "output_SolenoidReward"=→"SolenoidReward":bool)  [unwired: 3 in]
              "iTrial" <- w2448
              n1456 = local write "error out"(w2451) -> ()
            }
            frame "initTrial2" {
              # "trialUntilReward"
              n1457 = call "myRIO_BRig_RT__Case_Exp_subState_LC__initTrial__v4.vi"("input_dataCurrent"=w2473, "input_dataExp"=w2471, "input_dataLC"=w2483, "input_spout"=w2484, "input_dataTrial"=w2486) -> ("output_dataTrial"=w2485:u16[][], "output_LR_Wrong_Laser_l2"=w2475:bool, "output_dataCurrent"=w2472:u16[], "output_LR_Reward_Laser_l2"=w2476:bool, "output_LR_Reward_Event_l1"=w2482:bool, "output_LR_Wrong_Event_l1"=w2481:bool, "output_LR_Reward_Laser_l1"=w2480:bool, "output_LR_Wrong_Laser_l1"=w2479:bool, "output_LR_Reward_Event_l2"=w2478:bool, "output_LR_Wrong_Event_l2"=w2477:bool)  [unwired: 5 in]
              n1458 = call "myRIO_BRig_RT_dataExp_ItrialUntilReward.vi"() -> ("output_I_trialUntilReward"=w2490:i32)  [unwired: 11 in]
              n1459 = Index Array(array=w2471, index=w2490) -> (element=w2489:u16)
              n1460 = Equal?(x=w2484, y=enum16{"Left", "Right"}."Right") -> (x = y?=w2488:bool)
              n1461 = Not Equal To 0?(x=w2489) -> (x != 0?=w2487:bool)
              n1462 = xnode "Read/Write Control"("FPGA VI Reference In"=w2500, "error in"=w2499, "Left(F)_or_Right(T)"=w2488, "ignoreWrong"=w2487, "LR_reward_Event_l1"=w2482, "LR_wrong_Event_l1"=w2481, "LR_reward_Laser_l1"=w2480, "LR_wrong_Laser_l1"=w2479, "LR_reward_Event_l2"=w2478, "LR_wrong_Event_l2"=w2477, "LR_reward_Laser_l2"=w2476, "LR_wrong_laser_l2"=w2475) -> ("error out"=w2474:errorcluster)  [unwired: 1 out]
              n1463 = local write "error out"(w2474) -> ()
            }
            frame "initTrial3" {
              # "Cue1_CueType"
              n1464 = call "myRIO_BRig_RT_dataExp_CueLed.vi"() -> ("output_CueLed"=w2507:i32)  [unwired: 11 in]
              n1465 = call "myRIO_BRig_RT_arrTrig_init.vi"() -> ("output_arrTrig"=w2511:bool[])  [unwired: 11 in]
              n1466 = Index Array(array=w2508, index=w2507) -> (element=w2506:u16)
              n1467 = call "myRIO_BRig_RT_arrTrig_Cue1_CueType_AudioLed.vi"() -> ("output_arrTrig_Cue1_CueType_AudioLed"=w2509:i32)  [unwired: 11 in]
              n1468 = Not Equal To 0?(x=w2506) -> (x != 0?=w2505:bool)
              n1469 = call "myRIO_BRig_RT__Case_Exp_State_initTrial_dataTrial.vi"("input_spout"=w2526, "input_dataCurrent"=w2513, "input_dataExp"=w2508, "input_dataTrial"=w2528) -> ("output_laserPower_l2"=w2515:u16, "output_dataCurrent"=w2512:u16[], "output_dataTrial"=w2527:u16[][], "output_laserPower_l1"=w2523:u16)  [unwired: 4 in]
              n1470 = To Double Precision Float(number=w2523) -> (double precision float=w2525:dbl)
              n1471 = To Double Precision Float(number=w2515) -> (double precision float=w2518:dbl)
              n1472 = Replace Array Subset(array=w2511, new element=w2505, index=w2509) -> (w2510:bool[])
              n1473 = Divide(x=w2525, y=100.0 ("x")) -> (x/y=w2520:dbl)
              "power_l1" <- w2520
              n1474 = Divide(x=w2518, y=100.0 ("x")) -> (x/y=w2516:dbl)
              "power_l2" <- w2516
              n1475 = call "myRIO__convert__Voltage_to_FPGAvalue.vi"("input_voltage"=w2520) -> ("output_PortC"=w2519:i16)  [unwired: 9 in, 1 out]
              n1476 = call "myRIO__convert__Voltage_to_FPGAvalue.vi"("input_voltage"=w2516) -> ("output_PortC"=w2514:i16)  [unwired: 9 in, 1 out]
              n1477 = xnode "Read/Write Control"("FPGA VI Reference In"=w2522, "error in"=w2521, "AnaOut_0"=w2519, "AnaOut_1"=w2514) -> ("error out"=w2504:errorcluster)  [unwired: 1 out]
              n1478 = local write "error out"(w2504) -> ()
            }
            frame "initTrial4" {
              n1479 = call "myRIO_BRig_RT_dataTrial_activeRecording.vi"() -> ("output_activeRecording"=w2548:i32)  [unwired: 11 in]
              n1480 = call "myRIO_BRig_RT_dataCurrent_idxDataTrial.vi"() -> ("output_idxDataTrial"=w2551:i32)  [unwired: 11 in]
              n1481 = Index Array(array=w2553, index=w2551) -> (element=w2550:u16)
              n1482 = xnode "Read/Write Control"("FPGA VI Reference In"=w2543, "error in"=w2542, "A6_Act"="Recording") -> ("error out"=w2540:errorcluster)  [unwired: 1 out]
              n1483 = Boolean To (0,1)(Boolean="Recording") -> (0, 1=w2547:i16)
              n1484 = To Long Integer(number=w2550) -> (32bit integer=w2549:i32)
              n1485 = To Unsigned Word Integer(number=w2547) -> (unsigned 16bit integer=w2546:u16)
              n1486 = local write "error out"(w2540) -> ()
              n1487 = Replace Array Subset(array=w2552, new element=w2546, index (row)=w2549, index (col)=w2548) -> (w2545:u16[][])
            }
            frame "initTrial_LC_ENL1" {
              n1488 = call "myRIO_BRig_RT__Case_Exp_State_initTrial_LC_ENL1__v4.vi"("input_dataTrial"=w2572, "input_spout"=w2575, "input_arrTrig"=w2569, "input_dataBlock"=w2570, "input_dataLC"=w2576, "input_dataCurrent"=w2574) -> ("output_arrTrig"=w2568:bool[], "output_dataTrial"=w2571:u16[][], "output_dataCurrent"=w2573:u16[])  [unwired: 3 in]
            }
            frame "initTrial_LC_Cue1" {
              n1489 = call "myRIO_BRig_RT__Case_Exp_State_initTrial_LC_Cue1__v4.vi"("input_dataTrial"=w2591, "input_spout"=w2594, "input_arrTrig"=w2588, "input_dataBlock"=w2589, "input_dataLC"=w2595, "input_dataCurrent"=w2593) -> ("output_arrTrig"=w2587:bool[], "output_dataTrial"=w2590:u16[][], "output_dataCurrent"=w2592:u16[])  [unwired: 3 in]
            }
            frame "initTrial_LC_Sel" {
              n1490 = xnode "Read/Write Control"("FPGA VI Reference In"=w2608, "error in"=w2607, "A6_Act"=FALSE) -> ("error out"=w2609:errorcluster)  [unwired: 1 out]
              n1491 = local write "error out"(w2609) -> ()
              n1492 = call "myRIO_BRig_RT__Case_Exp_State_initTrial_LC_Sel__v4.vi"("input_dataTrial"=w2614, "input_spout"=w2617, "input_arrTrig"=w2611, "input_dataBlock"=w2612, "input_dataLC"=w2618, "input_dataCurrent"=w2616) -> ("output_arrTrig"=w2610:bool[], "output_dataTrial"=w2613:u16[][], "output_dataCurrent"=w2615:u16[])  [unwired: 3 in]
            }
            frame "ENL1_pre" {
              n1493 = call "myRIO_BRig_RT__Case_Exp_State_Enl1Pre__v3.vi"("input_I_lick"=w2632, "input_arrTrig"=w2629, "input_dataCurrent"=w2633) -> ("output_dataCurrent"=w2630:u16[], "output_state"=w2631:T2)  [unwired: 3 in, 4 out]
            }
            frame "ENL1" {
              n1494 = call "myRIO_BRig_RT__Case_Exp_State_ENL1__v3.vi"("I_lick"=w2652, "input_arrTrig"=w2650, "input_state"=w2656, "input_dataCurrent"=w2655) -> ("output_l1_laserOn"=w2648:bool, "output_l1_laserEvent"=w2649:bool, "output_state"=w2653:T2, "output_dataCurrent"=w2654:u16[], "output_l2_laserEvent"=w2647:bool, "output_l2_laserOn"=w2646:bool)  [unwired: 2 in]
            }
            frame "ENL1Penalty_pre" {
              # "Tcycle"
              # "counter"
              n1495 = call "myRIO_BRig_RT_dataCurrent_Tcycle_generic.vi"() -> ("output_Tcycle_generic"=w2683:i32)  [unwired: 11 in]
              n1496 = call "myRIO_BRig_RT_dataCurrent_count_generic.vi"() -> ("output_count_generic"=w2685:i32)  [unwired: 11 in]
              n1497 = call "myRIO_BRig_RT_dataExp_ENL_penalty.vi"() -> ("output_ENL_penalty"=w2678:i32)  [unwired: 11 in]
              n1498 = Index Array(array=w2679, index=w2678) -> (element=w2682:u16)
              n1499 = Replace Array Subset(array=w2680, new element #1=u16 0 ("new element/subarray"), index #1=w2685, new element #2=w2682, index #2=w2683) -> (w2681:u16[])
            }
            frame "ENL1Penalty" {
              n1500 = call "myRIO_BRig_RT__Case_Exp_State_ENL1Penalty.vi"("input_state"=w2699, "input_dataCurrent"=w2703) -> ("output_state"=w2700:T2, "output_dataCurrent"=w2702:u16[])  [unwired: 8 in]
            }
            frame "ENL2_pre" {
            }
            frame "ENL2" {
            }
            frame "ENL2Penalty_pre" {
            }
            frame "ENL2Penalty" {
            }
            frame "Cue1_pre" {
              n1501 = call "myRIO_BRig_RT__Case_Exp_State_Cue1Pre__v3.vi"("input_dataCurrent"=w2775, "input_dataExp"=w2771, "input_arrTrig"=w2768, "input_spout"=w2772) -> ("output_audioR"=w2769:bool, "output_audioL"=w2770:bool, "output_state"=w2773:T2, "output_dataCurrent"=w2774:u16[])  [unwired: 7 in, 5 out]
            }
            frame "Cue1" {
              n1502 = call "myRIO_BRig_RT__Case_Exp_State_Cue1__v4.vi"("input_state"=w2796, "input_dataCurrent"=w2797, "I_lick"=w2795, "input_arrTrig"=w2798) -> ("output_SelectionState"=w2789:bool, "output_CueLed_Event"=w2794:bool, "output_state"=w2790:T2, "output_dataCurrent"=w2791:u16[], "output_l1_laserEvent"=w2787:bool, "output_l1_laserOn"=w2788:bool, "output_l2_laserEvent"=w2792:bool, "output_l2_laserOn"=w2793:bool)  [unwired: 8 in]
              n1503 = xnode "Read/Write Control"("FPGA VI Reference In"=w2801, "error in"=w2800, "SelectionState"=w2789) -> ()  [unwired: 2 out]
            }
            frame "Cue1Penalty_pre" {
              # "Tcycle"
              # "counter"
              n1504 = call "myRIO_BRig_RT_dataCurrent_Tcycle_generic.vi"() -> ("output_Tcycle_generic"=w2837:i32)  [unwired: 11 in]
              n1505 = call "myRIO_BRig_RT_dataCurrent_count_generic.vi"() -> ("output_count_generic"=w2839:i32)  [unwired: 11 in]
              n1506 = call "myRIO_BRig_RT_dataExp_CueLed.vi"() -> ("output_CueLed"=w2821:i32)  [unwired: 11 in]
              n1507 = call "myRIO_BRig_RT_dataExp_Tcycle_Cue1Penalty_Audio.vi"() -> ("output_Tcycle_Cue1Penalty_Audio"=w2822:i32)  [unwired: 11 in]
              n1508 = call "myRIO_BRig_RT_dataExp_Tcycle_Cue1Penalty_LED.vi"() -> ("output_Tcycle_Cue1Penalty_LED"=w2820:i32)  [unwired: 11 in]
              n1509 = Index Array(array=w2833, index #1=w2821, index #2=w2822, index #3=w2820) -> (element #1=w2819:u16, element #2=w2817:u16, element #3=w2816:u16)
              n1510 = Equal To 0?(x=w2819) -> (x = 0?=w2818:bool)
              n1511 = Select(t=w2817, s=w2818, f=w2816) -> (s? t:f=w2815:u16)
              n1512 = Replace Array Subset(array=w2835, new element #1=u16 0 ("new element/subarray"), index #1=w2839, new element #2=w2815, index #2=w2837) -> (w2834:u16[])
            }
            frame "Cue1Penalty" {
              n1513 = call "myRIO_BRig_RT__Case_Exp_State_Cue1Penalty.vi"("input_state"=w2856, "input_dataCurrent"=w2857) -> ("output_state"=w2854:T2, "output_dataCurrent"=w2855:u16[])  [unwired: 8 in]
            }
            frame "Cue2_pre" {
            }
            frame "Cue2" {
            }
            frame "Cue2Penalty_pre" {
            }
            frame "Cue2Penalty" {
            }
            frame "Selection_pre" {
              n1514 = xnode "Read/Write Control"("FPGA VI Reference In"=w2935, "error in"=w2936) -> ("error out"=w2923:errorcluster, "SelectReward"=w2930:bool, "SelectWrong"=w2931:bool)  [unwired: 1 out]
              n1515 = local write "error out"(w2923) -> ()
              n1516 = call "myRIO_BRig_RT__Case_Exp_State_SelectPre__v5.vi"("input_dataCurrent"=w2934, "input_SelectWrong"=w2931, "input_SelectReward"=w2930, "input_dataExp"=w2924, "input_LickL"=w2922, "input_LickR"=w2921, "input_arrTrig"=w2929) -> ("output_state"=w2932:T2, "output_dataCurrent"=w2933:u16[], "output_l1_laserEvent"=w2928:bool, "output_l1_laserOn"=w2927:bool, "output_l2_laserOn"=w2925:bool, "output_l2_laserEvent"=w2926:bool)  [unwired: 3 in]
            }
            frame "Selection" {
              n1517 = xnode "Read/Write Control"("FPGA VI Reference In"=w2963, "error in"=w2962) -> ("error out"=w2950:errorcluster, "SelectReward"=w2957:bool, "SelectWrong"=w2956:bool)  [unwired: 1 out]
              n1518 = local write "error out"(w2950) -> ()
              n1519 = call "myRIO_BRig_RT__Case_Exp_State_Selection__v5.vi"("input_dataCurrent"=w2961, "input_state"=w2959, "input_dataExp"=w2949, "input_LickL"=w2948, "input_FPGA_SelectReward"=w2957, "input_FPGA_SelectWrong"=w2956, "input_LickR"=w2947, "input_arrTrig"=w2955) -> ("output_state"=w2958:T2, "output_dataCurrent"=w2960:u16[], "output_LC_Event_l1"=w2954:bool, "output_LC_Laser_l2"=w2951:bool, "output_LC_Event_l2"=w2952:bool, "output_LC_Laser_l1"=w2953:bool)  [unwired: 2 in]
            }
            frame "SelectReward_pre" {
              # "iState"
              # "nRewTrials"
              # "Tcycle\nGeneric"
              # "counter"
              n1520 = call "myRIO_BRig_RT_dataCurrent_nRewTrials.vi"() -> ("output_nRewTrials"=w2987:i32)  [unwired: 11 in]
              n1521 = call "myRIO_BRig_RT_dataCurrent_Tcycle_reward.vi"() -> ("output_Tcycle_reward"=w2976:i32)  [unwired: 11 in]
              n1522 = Index Array(array=w2974, index #1=w2987, index #2=w2976) -> (element #1=w2986:u16, element #2=w2975:u16)
              n1523 = Increment(x=w2986) -> (x+1=w2985:u16)
              n1524 = call "myRIO_BRig_RT__Case_Exp_subState_LC__Reward.vi"("input_spout"=w2994, "input_dataCurrent"=w2974, "input_dataLC"=w2993) -> ()  [unwired: 6 in, 2 out]
              n1525 = call "myRIO_BRig_RT_dataCurrent_count_generic.vi"() -> ("output_count_generic"=w2989:i32)  [unwired: 11 in]
              n1526 = call "myRIO_BRig_RT_dataCurrent_Tcycle_generic.vi"() -> ("output_Tcycle_generic"=w2990:i32)  [unwired: 11 in]
              n1527 = call "myRIO_BRig_RT_dataCurrent_iState.vi"() -> ("output_iState"=w2984:i32)  [unwired: 11 in]
              n1528 = Replace Array Subset(array=w2974, new element #1=w2985, index #1=w2987, new element #2=u16 0 ("new element/subarray"), index #2=w2989, new element #3=w2975, index #3=w2990, new element #4=u16 1 ("new element/subarray"), index #4=w2984) -> (w2996:u16[])
            }
            frame "SelectReward" {
              n1529 = call "myRIO_BRig_RT__Case_Exp_State_Reward__v2.vi"("input_dataCurrent"=w3014, "input_state"=w3011, "input_spout"=w3009, "input_dataExp"=w3001, "input_dataTrial"=w3000) -> ("output_dataCurrent"=w3013:u16[], "output_state"=w3012:T2, "output__L"=w3007:bool, "output__R"=w3008:bool)  [unwired: 7 in]
            }
            frame "SelectRewardPost_pre" {
              # "nRewards"
              # "nRewTrials"
              # "Tcycle"
              # "counter"
              n1530 = call "myRIO_BRig_RT_dataBlock_nRewards__L.vi"() -> ("output_nRewards__L"=w3029:i32)  [unwired: 11 in]
              n1531 = call "myRIO_BRig_RT_dataBlock_nRewards__R.vi"() -> ("output_nRewards__R"=w3028:i32)  [unwired: 11 in]
              n1532 = call "myRIO_BRig_RT_dataCurrent_Tcycle_generic.vi"() -> ("output_Tcycle_generic"=w3044:i32)  [unwired: 11 in]
              n1533 = call "myRIO_BRig_RT_dataCurrent_count_generic.vi"() -> ("output_count_generic"=w3046:i32)  [unwired: 11 in]
              n1534 = case shown="\"Left\", Default" w3022 {
                tunnel: w3034 -> [w3051 w3055]
                tunnel: [w3050 w3055] -> w3033
                tunnel: [w3052 w3053] -> w3032
                tunnel: w3031 -> [w3052 w3054]
                frame "Left", Default {
                  n1535 = Increment(x=w3051) -> (x+1=w3050:u16)
                }
                frame "Right" {
                  n1536 = Increment(x=w3054) -> (x+1=w3053:u16)
                }
              }
              "nRewards_Left" <- w3033
              "nRewards_Right" <- w3032
              n1537 = Equal?(x=w3022, y=enum16{"Left", "Right"}."Left") -> (x = y?=w3021:bool)
              n1538 = Select(t=w3029, s=w3021, f=w3028) -> (s? t:f=w3027:i32)
              n1539 = call "myRIO_BRig_RT_dataExp_Tcycle_RewardPost.vi"() -> ("output_Tcycle_RewardPost"=w3040:i32)  [unwired: 11 in]
              n1540 = call "myRIO_BRig_RT_dataCurrent_nRewTrials.vi"() -> ("output_nRewTrials"=w3030:i32)  [unwired: 11 in]
              n1541 = Index Array(array=w3041, index=w3040) -> (element=w3043:u16)
              n1542 = Index Array(array=w3024, index=w3030) -> (element=w3019:u16)
              n1543 = Replace Array Subset(array=w3024, new element #1=u16 0 ("new element/subarray"), index #1=w3046, new element #2=w3043, index #2=w3044) -> (w3042:u16[])
              n1544 = Replace Array Subset(array=w3026, new element=w3019, index (row)=w3020, index (col)=w3027) -> (w3025:u16[][])
              n1545 = local write "nRewards_cur"(w3019) -> ()
            }
            frame "SelectRewardPost" {
              n1546 = call "myRIO_BRig_RT__Case_Exp_State_RewardPost.vi"("input_state"=w3066, "input_dataCurrent"=w3069) -> ("output_state"=w3067:T2, "output_dataCurrent"=w3068:u16[])  [unwired: 8 in]
            }
            frame "SelectWrong_pre" {
              # "iState"
              # "Tcycle"
              # "counter"
              n1547 = call "myRIO_BRig_RT_dataCurrent_Tcycle_generic.vi"() -> ("output_Tcycle_generic"=w3090:i32)  [unwired: 11 in]
              n1548 = call "myRIO_BRig_RT_dataCurrent_count_generic.vi"() -> ("output_count_generic"=w3092:i32)  [unwired: 11 in]
              n1549 = call "myRIO_BRig_RT_dataExp_Tcycle_Wrong.vi"() -> ("output_Tcycle_Wrong"=w3088:i32)  [unwired: 11 in]
              n1550 = call "myRIO_BRig_RT__Case_Exp_subState_LC__Wrong.vi"("input_spout"=w3084, "input_dataCurrent"=w3085, "input_dataLC"=w3082) -> ()  [unwired: 6 in, 2 out]
              n1551 = Index Array(array=w3086, index=w3088) -> (element=w3089:u16)
              n1552 = call "myRIO_BRig_RT_dataCurrent_iState.vi"() -> ("output_iState"=w3080:i32)  [unwired: 11 in]
              n1553 = Replace Array Subset(array=w3085, new element #1=u16 0 ("new element/subarray"), index #1=w3092, new element #2=w3089, index #2=w3090, new element #3=u16 2 ("new element/subarray"), index #3=w3080) -> (w3087:u16[])
            }
            frame "SelectWrong" {
              n1554 = call "myRIO_BRig_RT__Case_Exp_State_Wrong.vi"("input_state"=w3106, "input_dataCurrent"=w3111) -> ("output_state"=w3103:T2, "output_dataCurrent"=w3110:u16[])  [unwired: 8 in]
              n1555 = Not Equal?(x=w3106, y=w3103) -> (x != y?=w3105:bool)
              n1556 = Select(t=myRIO_BRig_RT__Case_Exp_stateList."SelectWrong_post" ("Enum"), s=w3105, f=w3103) -> (s? t:f=w3102:T2)
            }
            frame "SelectWrong_post" {
            }
            frame "SelectTimeout_pre" {
              # "iState"
              # "Tcycle"
              # "counter"
              n1557 = xnode "Read/Write Control"("FPGA VI Reference In"=w3134, "error in"=w3133, "SelectionState"=FALSE) -> ("error out"=w3131:errorcluster)  [unwired: 1 out]
              n1558 = call "myRIO_BRig_RT_dataCurrent_Tcycle_generic.vi"() -> ("output_Tcycle_generic"=w3152:i32)  [unwired: 11 in]
              n1559 = call "myRIO_BRig_RT_dataCurrent_count_generic.vi"() -> ("output_count_generic"=w3150:i32)  [unwired: 11 in]
              n1560 = call "myRIO_BRig_RT_dataExp_Tcycle_Timeout.vi"() -> ("output_Tcycle_Timeout"=w3154:i32)  [unwired: 11 in]
              n1561 = local write "error out"(w3131) -> ()
              n1562 = call "myRIO_BRig_RT__Case_Exp_subState_LC__Timeout.vi"("input_spout"=w3145, "input_dataCurrent"=w3146, "input_dataLC"=w3144) -> ()  [unwired: 6 in, 2 out]
              n1563 = Index Array(array=w3148, index=w3154) -> (element=w3153:u16)
              n1564 = call "myRIO_BRig_RT_dataCurrent_iState.vi"() -> ("output_iState"=w3142:i32)  [unwired: 11 in]
              n1565 = Replace Array Subset(array=w3146, new element #1=u16 0 ("new element/subarray"), index #1=w3150, new element #2=w3153, index #2=w3152, new element #3=u16 3 ("new element/subarray"), index #3=w3142) -> (w3149:u16[])
            }
            frame "SelectTimeout" {
              n1566 = call "myRIO_BRig_RT__Case_Exp_State_Timeout.vi"("input_dataLC"=w3169, "input_state"=w3164, "input_dataCurrent"=w3174) -> ("output_state"=w3165:T2, "output_dataCurrent"=w3173:u16[])  [unwired: 6 in, 1 out]
              n1567 = Not Equal?(x=w3164, y=w3165) -> (x != y?=w3168:bool)
              n1568 = Select(t=myRIO_BRig_RT__Case_Exp_stateList."SelectTimeout_post" ("Enum"), s=w3168, f=w3165) -> (s? t:f=w3166:T2)
            }
            frame "SelectTimeout_post" {
            }
            frame "endTrial1" {
              # "Update dataBlock"
              n1569 = call "myRIO_BRig_RT__Case_Exp_State_endTrial1.vi"("input_spout"=w3203, "input_dataBlock"=w3202, "input_dataCurrent"=w3200) -> ("output_dataBlock"=w3201:u16[][], "output_dataCurrent"=w3199:u16[])  [unwired: 7 in]
            }
            frame "endTrial2" {
              # "update dataTrial"
              n1570 = call "myRIO_BRig_RT__Case_Exp_State_endTrial2.vi"("input_dataExp"=w3210, "input_spout"=w3219, "input_dataTrial"=w3223, "input_dataCurrent"=w3221) -> ("output_dataTrial"=w3222:u16[][], "output_dataCurrent"=w3220:u16[])  [unwired: 6 in]
            }
            frame "endTrial3" {
              # "nRewTrials"
              # "iTrial"
              # "I_blockUntilReward"
              # "TPB"
              # "end block?"
              n1571 = local read "STOP_endTrial"() -> (w3244:bool)
              n1572 = local read "STOP_abort"() -> (w3243:bool)
              n1573 = xnode "Read/Write Control"("FPGA VI Reference In"=w3234, "error in"=w3233, "SelectionState"=FALSE) -> ("error out"=w3227:errorcluster)  [unwired: 1 out]
              n1574 = local read "START"() -> (w3241:bool)
              n1575 = call "myRIO_BRig_RT_dataExp_IblockUntilReward.vi"() -> ("output_I_blockUntilReward"=w3251:i32)  [unwired: 11 in]
              n1576 = Index Array(array=w3237, index=w3251) -> (element=w3235:u16)
              n1577 = Not(x=w3241) -> (.not. x?=w3242:bool)
              n1578 = local write "error out"(w3227) -> ()
              n1579 = Not Equal To 0?(x=w3235) -> (x != 0?=w3249:bool)
              n1580 = Compound Arithmetic op=OR(w3244, w3242, w3243) -> (w3230:bool)
              n1581 = call "myRIO_BRig_RT_dataCurrent_nRewTrials.vi"() -> ("output_nRewTrials"=w3247:i32)  [unwired: 11 in]
              n1582 = call "myRIO_BRig_RT_dataCurrent_iTrial.vi"() -> ("output_iTrial"=w3248:i32)  [unwired: 11 in]
              n1583 = Select(t=w3247, s=w3249, f=w3248) -> (s? t:f=w3246:i32)
              n1584 = call "myRIO_BRig_RT_dataCurrent_TpB.vi"() -> ("output_TpB"=w3250:i32)  [unwired: 11 in]
              n1585 = Index Array(array=w3238, index #1=w3250, index #2=w3246) -> (element #1=w3239:u16, element #2=w3240:u16)
              n1586 = Less Or Equal?(x=w3239, y=w3240) -> (x <= y?=w3231:bool)
              n1587 = Or(x=w3230, y=w3231) -> (x .or. y?=w3228:bool)
              n1588 = Select(t=myRIO_BRig_RT__Case_Exp_stateList."saveData_dataBlock" ("Enum"), s=w3228, f=myRIO_BRig_RT__Case_Exp_stateList."dummyState" ("Enum")) -> (s? t:f=w3236:T2)
            }
            frame "endBlock" {
              # "R"
              # "L"
              # "idxDataBlock"
              n1589 = Equal?(x=w3271, y=enum16{"Left", "Right"}."Left") -> (x = y?=w3270:bool)
              n1590 = call "myRIO_BRig_RT_dataCurrent_idxDataBlockL.vi"() -> ("output_idxDataBlock__L"=w3274:i32)  [unwired: 11 in]
              n1591 = call "myRIO_BRig_RT_dataCurrent_idxDataBlockR.vi"() -> ("output_idxDataBlock__R"=w3273:i32)  [unwired: 11 in]
              n1592 = Increment(x=w3265) -> (x+1=w3264:i32)
              n1593 = local read "START"() -> (w3290:bool)
              n1594 = local read "STOP_endBlock"() -> (w3285:bool)
              n1595 = local read "STOP_endTrial"() -> (w3288:bool)
              n1596 = local read "STOP_abort"() -> (w3287:bool)
              n1597 = Select(t=w3274, s=w3270, f=w3273) -> (s? t:f=w3268:i32)
              n1598 = To Unsigned Word Integer(number=w3264) -> (unsigned 16bit integer=w3266:u16)
              n1599 = Not(x=w3290) -> (.not. x?=w3289:bool)
              n1600 = Replace Array Subset(array=w3269, new element=w3266, index=w3268) -> (w3267:u16[])
              n1601 = Compound Arithmetic op=OR(w3289, w3285, w3288, w3287) -> (w3286:bool)
              n1602 = Select(t=myRIO_BRig_RT__Case_Exp_stateList."endExp" ("Enum"), s=w3286, f=myRIO_BRig_RT__Case_Exp_stateList."dummyState_endBlock" ("Enum")) -> (s? t:f=w3294:T2)
            }
            frame "endExp" {
              n1603 = xnode "Read/Write Control"("FPGA VI Reference In"=w3297, "error in"=w3296, "A6_Act"=FALSE) -> ("error out"=w3298:errorcluster)  [unwired: 1 out]
              n1604 = local write "error out"(w3298) -> ()
            }
            frame "commConnect" {
              n1605 = call "myRIO_BRig_RT_comm_webdav_connect.vi"("input_password"="Host Password", "input_username"="Host UserName") -> ("output_Iconnected"=w3315:bool, "output_hSession"=w3329:T6)  [unwired: 7 in, 1 out]
              "Connected To Host?" <- w3315
              n1606 = case shown="False" w3315 {
                frame False {
                  n1607 = One Button Dialog(message="Connection Failed!\nData not being saved!") -> ()  [unwired: 1 in, 1 out]
                }
                frame True {
                }
              }
            }
            frame "commUpload_pre" {
              n1608 = Select(t=myRIO_BRig_RT__Case_Exp_stateList."commUpload_dataBlock" ("Enum"), s=w3336, f=myRIO_BRig_RT__Case_Exp_stateList."endBlock") -> (s? t:f=w3334:T2)
            }
            frame "commUpload_dataBlock" {
              n1609 = call "myRIO_BRig_RT_comm_webdav_uploadFile__data.vi"("input_fileName_prefix"=w3353, "input_fileName"="dataBlock" ("input_filename"), "input_hSession"=w3355) -> ()  [unwired: 8 in, 1 out]
            }
            frame "commUpload_dataCurrent" {
              n1610 = call "myRIO_BRig_RT_comm_webdav_uploadFile__data.vi"("input_fileName_prefix"=w3370, "input_fileName"="dataCurrent" ("input_filename"), "input_hSession"=w3372) -> ()  [unwired: 8 in, 1 out]
            }
            frame "commUpload_dataExp" {
              n1611 = call "myRIO_BRig_RT_comm_webdav_uploadFile__data.vi"("input_fileName_prefix"=w3387, "input_fileName"="dataExp" ("input_filename"), "input_hSession"=w3389) -> ()  [unwired: 8 in, 1 out]
            }
            frame "commUpload_dataLC" {
              n1612 = call "myRIO_BRig_RT_comm_webdav_uploadFile__data.vi"("input_fileName_prefix"=w3404, "input_fileName"="dataLC" ("input_filename"), "input_hSession"=w3406) -> ()  [unwired: 8 in, 1 out]
            }
            frame "commUpload_dataTrial" {
              n1613 = call "myRIO_BRig_RT_comm_webdav_uploadFile__data.vi"("input_fileName_prefix"=w3424, "input_fileName"="dataTrial" ("input_filename"), "input_hSession"=w3426) -> ()  [unwired: 8 in, 1 out]
            }
            frame "saveData_dataBlock" {
              # "idxDataBlockR"
              # "idxDataBlockL"
              n1614 = call "myRIO_BRig_RT_dataCurrent_idxDataBlockL.vi"() -> ("output_idxDataBlock__L"=w3446:i32)  [unwired: 11 in]
              n1615 = call "myRIO_BRig_RT_dataCurrent_idxDataBlockR.vi"() -> ("output_idxDataBlock__R"=w3447:i32)  [unwired: 11 in]
              n1616 = Index Array(array=w3448, index #1=w3446, index #2=w3447) -> (element #1=w3445:u16, element #2=w3444:u16)
              n1617 = Greater?(x=w3445, y=w3444) -> (0:w3443:bool)
              n1618 = Select(t=w3445, s=w3443, f=w3444) -> (s? t:f=w3441:u16)
              n1619 = Increment(x=w3441) -> (x+1=w3440:u16)
              n1620 = To Long Integer(number=w3440) -> (32bit integer=w3439:i32)
              n1621 = Array Subset(array=w3442, length (row)=w3439) -> (w3438:u16[][])  [unwired: 3 in]
              n1622 = call "myRIO_BRig_RT_comm_webdav_saveArrayToFile__2D_u16.vi"("Array"=w3438, "input_filename"="dataBlock") -> ()  [unwired: 10 in]
            }
            frame "saveData_dataCurrent" {
              n1623 = call "myRIO_BRig_RT_comm_webdav_saveArrayToFile__1D_u16.vi"("Array"=w3463, "input_filename"="dataCurrent") -> ()  [unwired: 10 in]
            }
            frame "saveData_dataExp" {
              # "runTime"
              n1624 = Get Date/Time In Seconds() -> (seconds since 1Jan1904=w3487:timestamp)
              n1625 = To Double Precision Float(number=w3487) -> (double precision float=w3486:dbl)
              n1626 = call "myRIO_BRig_RT_dataExp_runTime_seconds.vi"() -> ("output_RunTime_minutes"=w3485:i32)  [unwired: 11 in]
              n1627 = Subtract(x=w3486, y=w3484) -> (x-y=w3481:dbl)
              n1628 = To Unsigned Word Integer(number=w3481) -> (unsigned 16bit integer=w3480:u16)
              n1629 = Replace Array Subset(array=w3479, new element=w3480, index=w3485) -> (w3482:u16[])
              n1630 = call "myRIO_BRig_RT_comm_webdav_saveArrayToFile__1D_u16.vi"("Array"=w3482, "input_filename"="dataExp") -> ()  [unwired: 10 in]
            }
            frame "saveData_dataLC" {
              n1631 = call "myRIO_BRig_RT_comm_webdav_saveArrayToFile__1D_u16.vi"("Array"=w3502, "input_filename"="dataLC") -> ()  [unwired: 10 in]
            }
            frame "saveData_dataTrial" {
              # "idxTrial"
              n1632 = call "myRIO_BRig_RT_dataCurrent_idxDataTrial.vi"() -> ("output_idxDataTrial"=w3522:i32)  [unwired: 11 in]
              n1633 = Index Array(array=w3523, index=w3522) -> (element=w3515:u16)
              n1634 = Increment(x=w3515) -> ()  [unwired: 1 out]
              n1635 = To Long Integer(number=w3515) -> (32bit integer=w3519:i32)
              n1636 = Array Subset(array=w3520, length (row)=w3519) -> (w3521:u16[][])  [unwired: 3 in]
              n1637 = call "myRIO_BRig_RT_comm_webdav_saveArrayToFile__2D_u16.vi"("Array"=w3521, "input_filename"="dataTrial") -> ()  [unwired: 10 in]
            }
            frame "dummyState" {
              n1638 = call "myRIO_BRig_RT_dataCurrent_iTrial.vi"() -> ("output_iTrial"=w3541:i32)  [unwired: 11 in]
              n1639 = Index Array(array=w3542, index=w3541) -> (element=w3540:u16)
              n1640 = Equal?(x=w3540, y=u16 1) -> (x = y?=w3538:bool)
              n1641 = Equal To 0?(x=w3549) -> (x = 0?=w3550:bool)
              n1642 = Select(t=u16 13, s=w3538, f=u16 15) -> (s? t:f=w3535:u16)
              n1643 = Select(t=w3535, s=w3550, f=w3549) -> (s? t:f=w3548:u16)
              n1644 = Decrement(x=w3548) -> (x-1=w3547:u16)
              n1645 = Equal To 0?(x=w3547) -> (x = 0?=w3546:bool)
              n1646 = Select(t=myRIO_BRig_RT__Case_Exp_stateList."initTrial" ("Enum"), s=w3546, f=w3544) -> (s? t:f=w3543:T2)
            }
            frame "dummyState_endBlock" {
              n1647 = call "myRIO_BRig_RT_dataCurrent_iTrial.vi"() -> ("output_iTrial"=w3570:i32)  [unwired: 11 in]
              n1648 = Index Array(array=w3571, index=w3570) -> (element=w3569:u16)
              n1649 = Equal?(x=w3569, y=u16 1) -> (x = y?=w3567:bool)
              n1650 = Equal To 0?(x=w3578) -> (x = 0?=w3579:bool)
              n1651 = Select(t=u16 1, s=w3567, f=u16 3) -> (s? t:f=w3564:u16)
              n1652 = Select(t=w3564, s=w3579, f=w3578) -> (s? t:f=w3577:u16)
              n1653 = Decrement(x=w3577) -> (x-1=w3576:u16)
              n1654 = Equal To 0?(x=w3576) -> (x = 0?=w3575:bool)
              n1655 = Select(t=myRIO_BRig_RT__Case_Exp_stateList."initBlock" ("Enum"), s=w3575, f=w3573) -> (s? t:f=w3572:T2)
            }
          }
          n1656 = call "myRIO_BRig_RT_dataMTrig_main.vi"("input_dataMTrig"=w1662, "input_Solenoid_trig_L"=w1659, "input_Solenoid_trig_R"=w1658, "input_Audio_trig_L"=w1657, "input_Audio_trig_R"=w1656, "input_Laser_trig"=w1655) -> ("output_Laser"=w1596:bool, "output_dataMTrig"=w1661:u16[], "output_Solenoid_L"=w1599:bool, "output_Solenoid_R"=w1651:bool, "output_Audio_L"=w1653:bool, "output_Audio_R"=w1654:bool)  [unwired: 8 in]
          n1657 = Compound Arithmetic op=OR(w1659, w1658, w1657, w1656, w1655) -> (w1660:bool)
          n1658 = case shown="True" w1660 {
            frame False {
            }
            frame True {
              w1692 = FALSE
              n1659 = local write "MTrig_Solenoid_trig__L"(w1692) -> ()
              n1660 = local write "MTrig_Solenoid_trig__R"(w1692) -> ()
              n1661 = local write "MTrig_Audio_trig__L"(w1692) -> ()
              n1662 = local write "MTrig_Audio_trig__R"(w1692) -> ()
              n1663 = local write "MTrig_Laser_trig"(w1692) -> ()
            }
          }
          n1664 = local read "MTrig_Laser_Switch"() -> (w1594:bool)
          n1665 = Not(x=w1594) -> (.not. x?=w1595:bool)
          n1666 = And(x=w1596, y=w1595) -> (x .and. y?=w1590:bool)
          n1667 = And(x=w1596, y=w1594) -> (x .and. y?=w1592:bool)
          n1668 = Or(x=w1593, y=w1592) -> (x .or. y?=w1583:bool)
          n1669 = Or(x=w1592, y=w1591) -> (x .or. y?=w1582:bool)
          n1670 = Or(x=w1589, y=w1590) -> (x .or. y?=w1585:bool)
          n1671 = Or(x=w1590, y=w1588) -> (x .or. y?=w1584:bool)
          n1672 = Or(x=w1598, y=w1599) -> (x .or. y?=w1587:bool)
          n1673 = Or(x=w1652, y=w1651) -> (x .or. y?=w1586:bool)
          n1674 = case shown="False" w1672 {
            tunnel: w1669 -> [w1694 w1702]
            tunnel: w1671 -> [_ w1699]
            tunnel: w1670 -> [_ w1698]
            tunnel: w1573 -> [_ w1697]
            tunnel: w1649 -> [_ w1696]
            tunnel: [w1694 w1701] -> w1668
            tunnel: [w1693 w1700] -> w1667
            tunnel: w1581 -> [w1693 w1695]
            frame False {
            }
            frame True {
              n1675 = call "myRIO_BRig_RT__Case_Exp__recordLick.vi"("intput_state__trialEnd"=w1696, "intput_state__trialStart"=w1697, "input_lick__R"=w1698, "input_lick__L"=w1699, "input_dataCurrent"=w1695, "input_dataLick"=w1702) -> ("output_dataCurrent"=w1700:u16[], "output_dataLick"=w1701:u16[][])  [unwired: 4 in]
            }
          }
          n1676 = Or(x=w1653, y=w1639) -> (x .or. y?=w1629:bool)
          n1677 = Or(x=w1638, y=w1654) -> (x .or. y?=w1650:bool)
          n1678 = Or(x=w1673, y="STOP_abort") -> (x .or. y?=w1675:bool)
          n1679 = Select(t=w1619, s=w1620, f=w1618) -> (s? t:f=w1609:u16)
          n1680 = Select(t=w1580, s=w1622, f=w1621) -> (s? t:f=w1608:u16)
          n1681 = Select(t=u16 0, s=w1625, f=w1624) -> (s? t:f=w1611:u16)
          n1682 = xnode "Read/Write Control"("FPGA VI Reference In"=w1631, "error in"=w1630, "audioTrigger_L"=w1629, "audioTrigger_R"=w1650, "CueLed_Event"=w1597, "A3_SL"=w1587, "A1_SR"=w1586, "LC_Event_l1"=w1585, "LC_Laser_l1"=w1584, "LC_Event_l2"=w1583, "LC_Laser_l2"=w1582) -> ("FPGA VI Reference Out"=w1666:refnum<k20>, "error out"=w1665:errorcluster, "AnaIn_0"=w1602:i16, "AnaIn_1"=w1610:i16)
          n1683 = call "myRIO_BRig_RT_dataAnalog_enterData__PortC.vi"("input_iState"=w1573, "input_AI0"=w1602, "input_iEvent"=w1611, "input_AI1"=w1610, "input_iTrial"=w1609, "input_iBlock"=w1608, "input_index"=w1612, "input_dataAnalog"=w1628) -> ("output_dataAnalog"=w1627:u16[][])  [unwired: 3 in]
          n1684 = call "myRIO_BRig_RT_TCP__v3__PortC.vi"("input_hTCP"=w1616, "input_AI1"=w1610, "input_AI0"=w1602, "input_I_connected_TCP"=w1613, "input_iBlock"=w1608, "input_spout"=w1607, "input_iTrial"=w1609, "input_error"=w1614, "input_countTrial"=w1604, "input_iState"=w1573) -> ("output_hTCP"=w1615:refnum<k5>, "output_countTrial"=w1603:u16, "output_error"=w1577:errorcluster)  [unwired: 3 in]
          n1685 = call "test_myRIO_Exp_tLoop.vi"("input_error"=w1577, "input_Threshold"=w1574, "input_timestamp"=w1575, "input_state"=w1573) -> ("output_Threshold"=w1571:bool, "output_duration"=→"tLoop":dbl, "error out"=w1576:errorcluster)  [unwired: 5 in]
          "Threshold" <- w1571
          n1686 = node-c288() -> ()  [unwired: 1 in, 1 out]
          n1687 = Increment(x=w1611) -> (x+1=w1617:u16)
          n1688 = Increment(x=w1612) -> (x+1=w1626:i32)
          "cState" <- w1573
        }
        n1689 = node-c288(w1514) -> ()  [unwired: 1 out]
        n1690 = flat-sequence {
          tunnel: w1510 -> [w1559]
          tunnel: w1509 -> [w1558]
          tunnel: [w1557] -> w1502
          tunnel: [w1556] -> w1501
          tunnel: [w1562] -> w1503
          tunnel: [w1563] -> w1508
          tunnel: w1502 -> [w1563]
          tunnel: w1501 -> [w1562]
          frame #0 {
            w1553 = u8 0
            w1554 = u16 0 ("AudioLeft_phase_inc")
            w1555 = FALSE
            n1691 = xnode "Read/Write Control"("FPGA VI Reference In"=w1559, "error in"=w1558, "Counts_Reset"=TRUE, "audioTrigger_L"=w1555, "audioFreq_L_kHz"=w1553, "audioAmp_L"=w1554, "audioTrigger_R"=w1555, "audioFreq_R_kHz"=w1553, "audioAmp_R"=w1554, "A3_SL"=w1555, "A1_SR"=w1555, "A6_Act"=w1555) -> ("FPGA VI Reference Out"=w1557:refnum<k20>, "error out"=w1556:errorcluster)
          }
          frame #1 {
            w1561 = FALSE ("START")
            n1692 = local write "START"(w1561) -> ()
            n1693 = local write "STOP_endTrial"(w1561) -> ()
            n1694 = local write "STOP_endBlock"(w1561) -> ()
          }
        }
        n1695 = stacked-sequence {
          tunnel: w1487 -> [w1533 _]
          tunnel: w1485 -> [w1534 _]
          tunnel: w1484 -> [_ w1539]
          tunnel: w1483 -> [_ w1538]
          tunnel: w1482 -> [_ w1537]
          tunnel: w1481 -> [w1527 _]
          tunnel: w1463 -> [w1524 _]
          tunnel: w1462 -> [w1523 _]
          frame #0 {
            n1696 = call "myRIO_BRig_RT_dataCurrent_idxDataLick.vi"() -> ("output_idxDataLick"=w1528:i32)  [unwired: 11 in]
            n1697 = Index Array(array=w1527, index=w1528) -> (element=w1530:u16)
            n1698 = Array Subset(array=w1524, length (row)=w1523) -> (w1525:u16[][])  [unwired: 3 in]
            n1699 = Increment(x=w1530) -> (x+1=w1531:u16)
            n1700 = call "myRIO_BRig_RT_comm_webdav_saveArrayToFile__1D_u16.vi"("Array"=w1534, "input_filename"="dataMTrig") -> ()  [unwired: 10 in]
            n1701 = To Long Integer(number=w1531) -> (32bit integer=w1529:i32)
            n1702 = Array Subset(array=w1533, length (row)=w1529) -> (w1532:u16[][])  [unwired: 3 in]
            n1703 = call "myRIO_BRig_RT_comm_webdav_saveArrayToFile__2D_u16.vi"("Array"=w1532, "input_filename"="dataLick") -> ()  [unwired: 10 in]
            n1704 = call "myRIO_BRig_RT_comm_webdav_saveArrayToFile__2D_u16.vi"("Array"=w1525, "input_filename"="dataAnalog") -> ()  [unwired: 10 in]
          }
          frame #1 {
            n1705 = case shown="True" w1539 {
              tunnel: w1538 -> [_ w1541]
              tunnel: w1537 -> [_ w1540]
              frame False {
              }
              frame True {
                n1706 = stacked-sequence {
                  tunnel: w1541 -> [w1543 w1550 w1552]
                  tunnel: w1540 -> [w1544 w1549 _]
                  frame #0 {
                    n1707 = call "myRIO_BRig_RT_comm_webdav_uploadFile__announce.vi"("input_addText"=TRUE, "input_fileName_prefix"=w1544, "intput_fileName"="curExp_end", "intput_hSession"=w1543) -> ("output_Isuccess"=w1542:bool)  [unwired: 6 in, 1 out]
                    n1708 = case shown="True" w1542 {
                      frame False {
                        n1709 = One Button Dialog(message="!!! Warning !!! Your data is located at C:\\BehaviorRig\\commTransfer") -> ()  [unwired: 1 in, 1 out]
                      }
                      frame True {
                        n1710 = Wait (ms)(milliseconds to wait=u32 20) -> ()  [unwired: 1 out]
                      }
                    }
                  }
                  frame #1 {
                    n1711 = call "myRIO_BRig_RT__endExp_sendData.vi"("input_fileName_prefix"=w1549, "input_hSession"=w1550) -> ()  [unwired: 8 in, 2 out]
                  }
                  frame #2 {
                    n1712 = local write "Connected To Host?"(FALSE ("Connected To Host?")) -> ()
                    n1713 = call <vilib>:"Close Session.vi"("session handle"=w1552) -> ()  [unwired: 14 in, 1 out]
                  }
                }
              }
            }
          }
        }
      }
    }
    n1714 = local read "STOP_abort"() -> (w44:bool)
  }
  n1715 = case shown="True" w5 {
    tunnel: w4 -> [_ w3598]
    tunnel: w3 -> [_ w3597]
    frame False {
    }
    frame True {
      n1716 = call "myRIO__TCP_disconnect_forWrite.vi"("input_error"=w3597, "input_hTCP"=w3598) -> ()  [unwired: 9 in, 1 out]
    }
  }
  n1717 = xnode "Read/Write Control"("FPGA VI Reference In"=w16, "error in"=w15, "FPGA_Stop"=TRUE) -> ("FPGA VI Reference Out"=w21:refnum<k20>, "error out"=w22:errorcluster)
  n1718 = xnode "Close FPGA VI Reference"("FPGA VI Reference In"=w21, "error in"=w22) -> ("error out"=w20:errorcluster)
  n1719 = call <vilib>:"Reset myRIO.vi"("error in (no error)"=w20) -> ()  [unwired: 10 in, 1 out]
